vi "WVDIAL+HSRL_v5.6.vi"() -> ()   [LabVIEW 2012]
uses:
  C:/Users/eol-lidar/Desktop/20171016_WVDIALLabviewSlimmed/DLLs/PowerMeterCommands.dll
  DLLs/PowerMeterCommands.dll
  <vilib>/DAQmx/write.llb/DAQmx Write (Digital 1D Bool NChan 1Samp 1Line).vi
  <vilib>/DAQmx/miscellaneous.llb/DAQmx Fill In Error Info.vi
  <vilib>/Analysis/baseanly.llb/Mean (DBL).vi
  WVD-MCSupdate/WVDMCSupdate/Subroutines/AMCS_Data.vi
  Shared Telescope WV DIAL Code/Libraries and VIs/Scalar_Data.vi
  <vilib>/Analysis/NI_AALBase.lvlib
  Shared Telescope WV DIAL Code/Libraries and VIs/Scalar_Data_2.vi
  Shared Telescope WV DIAL Code/Libraries and VIs/Scalar_Data_4.vi
  Shared Telescope WV DIAL Code/Libraries and VIs/Scalar_Data_3.vi
  DLLs/CLDevIFace.dll
panel:
  out "sigma_off_total":dbl[](array[numeric])=[5.561752182192097e-25, 5.543502425482937e-25, 5.525286776509028e-25, 5.507105267834132e-25, 5.488957932126663e-25, 5.470844802256444e-25, 5.452765911101733e-25, 5.434721291706492e-25, 5.416710977203383e-25, 5.398735000734361e-25, 5.380793395556204e-25, 5.362886194923337e-25, 5.345013432148163e-25, 5.327175140545496e-25, 5.309371353401882e-25, 5.2916021040427205e-25, 5.273867425735806e-25, 5.256167351714557e-25, 5.238501915156585e-25, 5.220871149168608e-25, 5.2032750867970615e-25, 5.185713760965108e-25, 5.16818720451498e-25, 5.150695450167362e-25, 5.133238530494676e-25, 5.115816477960978e-25, 5.098429324843519e-25, 5.081077103253636e-25, 5.063759845141784e-25, 5.046477582239893e-25, 5.0292303461145e-25, 5.012018168074178e-25, 4.994841079208481e-25, 4.977699110405206e-25, 4.960592292252991e-25, 4.943520655119366e-25, 4.9264842290519855e-25, 4.909483043867978e-25, 4.892517129052874e-25, 4.875586513787884e-25, 4.858691226971689e-25, 4.841831297166355e-25, 4.825006752543411e-25, 4.808217621002523e-25, 4.791463930057659e-25, 4.774745706846224e-25, 4.7580629781515705e-25, 4.741415770356795e-25, 4.724804109451955e-25, 4.708228021047316e-25, 4.6916875303125385e-25, 4.67518266200415e-25, 4.6587134404804e-25, 4.642279889605549e-25, 4.625882032864318e-25, 4.609519893243784e-25, 4.593193493288615e-25, 4.576902855057731e-25, 4.560648000174122e-25, 4.544428949731033e-25, 4.528245724384268e-25, 4.512098344233702e-25, 4.495986828926446e-25, 4.479911197575997e-25, 4.463871468777747e-25, 4.447867660625189e-25, 4.43189979068954e-25, 4.415967875975391e-25, 4.400071932975711e-25, 4.384211977618739e-25, 4.36838802531331e-25, 4.352600090892456e-25, 4.336848188647951e-25, 4.321132332291639e-25, 4.305452534971783e-25, 4.289808809279486e-25, 4.2742011672071225e-25, 4.258629620199571e-25, 4.243094179083304e-25, 4.227594854132745e-25, 4.212131655002161e-25, 4.196704590788522e-25, 4.181313669960296e-25, 4.165958900404223e-25, 4.150640289409102e-25, 4.1353578436580916e-25, 4.12011156923498e-25, 4.104901471585589e-25, 4.089727555606462e-25, 4.0745898255287632e-25, 4.059488284993571e-25, 4.0444229370438294e-25, 4.0293937840896656e-25, 4.014400827940419e-25, 3.999444069755499e-25, 3.9845235101354183e-25, 3.969639149014037e-25, 3.9547909857346956e-25, 3.939979019023365e-25, 3.925203246968599e-25, 3.9104636670814153e-25, 3.8957602762028764e-25, 3.8810930706173083e-25, 3.866462045949355e-25, 3.85186719722267e-25, 3.837308518864686e-25, 3.8227860046637432e-25, 3.80829964782557e-25, 3.793849440915136e-25, 3.779435375918537e-25, 3.7650574441937656e-25, 3.750715636524266e-25, 3.7364099430430667e-25, 3.7221403533351837e-25, 3.7079068563566637e-25, 3.693709440478561e-25, 3.6795480934616738e-25, 3.6654228024909808e-25, 3.651333554181692e-25, 3.6372803345242974e-25, 3.6232631289607184e-25, 3.609281922331212e-25, 3.5953366989007554e-25, 3.5814274423905253e-25, 3.5675541359037734e-25, 3.5537167620271367e-25, 3.539915302741494e-25, 3.5261497395062725e-25, 3.512420053194509e-25, 3.4987262241518894e-25, 3.4850682321588814e-25, 3.471446056456973e-25, 3.4578596757510757e-25, 3.4443090682164883e-25, 3.430794211490976e-25, 3.4173150826695617e-25, 3.40387165836129e-25, 3.390463914606158e-25, 3.37709182699569e-25, 3.3637553705486374e-25, 3.350454519816831e-25, 3.337189248846164e-25, 3.323959531178655e-25, 3.3107653398769254e-25, 3.29760664750051e-25, 3.2844834261511436e-25, 3.271395647443673e-25, 3.2583432825129606e-25, 3.2453263020474272e-25, 3.2323446762705243e-25, 3.2193983749323496e-25, 3.2064873673450423e-25, 3.193611622390686e-25, 3.180771108479372e-25, 3.167965793620153e-25, 3.1551956453621976e-25, 3.1424606308521448e-25, 3.12976071680503e-25, 3.117095869534258e-25, 3.104466054941991e-25, 3.091871238497953e-25, 3.0793113853283025e-25, 3.0667864601217453e-25, 3.0542964272015646e-25, 3.0418412505014397e-25, 3.029420893588374e-25, 3.0170353196359345e-25, 3.0046844914894554e-25, 2.992368371589509e-25, 2.980086922059933e-25, 2.9678401046518705e-25, 2.9556278807888944e-25, 2.943450211532379e-25, 2.9313070576457556e-25, 2.9191983795267953e-25, 2.907124137258925e-25, 2.895084290635122e-25, 2.8830787991081537e-25, 2.8711076218309027e-25, 2.859170717652124e-25, 2.8472680451222477e-25, 2.8353995625196194e-25, 2.8235652277975173e-25, 2.8117649986558313e-25, 2.7999988325219016e-25, 2.7882666865307774e-25, 2.7765685175696382e-25, 2.7649042822429354e-25, 2.7532739369120183e-25, 2.741677437688488e-25, 2.730114740426547e-25, 2.718585800741375e-25, 2.7070905740222066e-25, 2.69562901540157e-25, 2.6842010798079194e-25, 2.6728067219283387e-25, 2.661445896234197e-25, 2.6501185569798014e-25, 2.6388246582293247e-25, 2.6275641538023513e-25, 2.616336997356157e-25, 2.60514314231774e-25, 2.593982541945556e-25, 2.5828551492935465e-25, 2.5717609172346685e-25, 2.560699798464901e-25, 2.549671745497334e-25, 2.538676710668411e-25, 2.5277146461645525e-25, 2.516785503976567e-25, 2.505889235961241e-25, 2.4950257938010373e-25, 2.4841951290291143e-25, 2.473397193030522e-25, 2.462631937044531e-25, 2.451899312145577e-25, 2.4411992693046025e-25, 2.430531759322844e-25, 2.4198967328846266e-25, 2.4092941405420186e-25, 2.39872393272301e-25, 2.388186059712237e-25, 2.3776804717002872e-25, 2.367207118736947e-25, 2.356765950782586e-25, 2.3463569176525954e-25, 2.335979969081922e-25, 2.325635054684053e-25, 2.3153221239689333e-25, 2.3050411263537554e-25, 2.294792011154746e-25, 2.284574727588212e-25, 2.274389224766938e-25, 2.264235451747459e-25, 2.2541133574601266e-25, 2.244022890765239e-25, 2.23396400044333e-25, 2.2239366351836315e-25, 2.21394074360395e-25, 2.203976274244917e-25, 2.1940431755605105e-25, 2.1841413959462833e-25, 2.1742708837184026e-25, 2.1644315871301047e-25, 2.154623454360858e-25, 2.144846433525735e-25, 2.135100472690121e-25, 2.1253855198334254e-25, 2.115701522900455e-25, 2.1060484297541854e-25, 2.0964261882209755e-25, 2.086834746060555e-25, 2.077274050997275e-25, 2.0677440506727251e-25, 2.058244692709451e-25, 2.048775924672437e-25, 2.0393376940616113e-25, 2.029929948357508e-25, 2.02055263498564e-25, 2.0112057013347119e-25, 2.0018890947358364e-25, 1.9926027625051027e-25, 1.9833466518985033e-25, 1.9741207101473141e-25, 1.9649248844463167e-25, 1.955759121953354e-25, 1.9466233697862308e-25, 1.9375175750525877e-25, 1.9284416848027954e-25, 1.919395646078448e-25, 1.9103794058885478e-25, 1.9013929112014526e-25, 1.8924361089835089e-25, 1.883508946160345e-25, 1.874611369639862e-25, 1.865743326301891e-25, 1.856904763013215e-25, 1.8480956266241805e-25, 1.839315863955293e-25, 1.8305654218173796e-25, 1.821844247006056e-25, 1.813152286297103e-25, 1.8044894864538793e-25, 1.7958557942351787e-25, 1.7872511563801019e-25, 1.7786755196193276e-25, 1.7701288306748196e-25, 1.76161103626729e-25, 1.7531220831027008e-25, 1.7446619178844077e-25, 1.7362304873139562e-25, 1.7278277380850455e-25, 1.719453616897912e-25, 1.711108070452065e-25, 1.7027910454420425e-25, 1.6945024885607005e-25, 1.6862423465142029e-25, 1.6780105660194305e-25, 1.6698070937813746e-25, 1.6616318765208027e-25, 1.6534848609801538e-25, 1.6453659938919535e-25, 1.6372752220073944e-25, 1.6292124920939515e-25, 1.6211777509352618e-25, 1.6131709453201433e-25, 1.6051920220608325e-25, 1.5972409280010035e-25, 1.5893176099733145e-25, 1.5814220148607808e-25, 1.5735540895495118e-25, 1.5657137809645292e-25, 1.5579010360478875e-25, 1.550115801761175e-25, 1.5423580251066348e-25, 1.5346276531215311e-25, 1.526924632848639e-25, 1.5192489113829988e-25, 1.5116004358516276e-25, 1.5039791534159869e-25, 1.4963850112671256e-25, 1.4888179566389964e-25, 1.481277936803633e-25, 1.473764899079385e-25, 1.4662787908173867e-25, 1.458819559412238e-25, 1.4513871523192763e-25, 1.4439815170135076e-25, 1.4366026010455229e-25, 1.4292503519884967e-25, 1.421924717483398e-25, 1.4146256452148893e-25, 1.4073530829242735e-25, 1.4001069783998057e-25, 1.3928872794854995e-25, 1.3856939340929826e-25, 1.3785268901741972e-25, 1.371386095751444e-25, 1.3642714988960654e-25, 1.3571830477488732e-25, 1.3501206905045525e-25, 1.3430843754217699e-25, 1.3360740508330465e-25, 1.3290896651114226e-25, 1.322131166719735e-25, 1.3151985041651617e-25, 1.308291626038556e-25, 1.3014104809867663e-25, 1.294555017723453e-25, 1.2877251850416015e-25, 1.280920931788039e-25, 1.2741422068882974e-25, 1.267388959336285e-25, 1.260661138194001e-25, 1.2539586925949367e-25, 1.2472815717427464e-25, 1.2406297249099328e-25, 1.23400310144304e-25, 1.2274016507553443e-25, 1.220825322337212e-25, 1.2142740657460956e-25, 1.2077478306075468e-25, 1.2012465666234459e-25, 1.1947702235651984e-25, 1.1883187512715506e-25, 1.1818920996493988e-25, 1.1754902186795484e-25, 1.1691130584132554e-25, 1.1627605689635239e-25, 1.156432700517033e-25, 1.1501294033236773e-25, 1.143850627699186e-25, 1.1375963240293268e-25, 1.131366442760479e-25, 1.1251609344039169e-25, 1.1189797495335014e-25, 1.1128228387839706e-25, 1.1066901528543347e-25, 1.100581642493591e-25, 1.0944972585195393e-25, 1.0884369518037427e-25, 1.0824006732660947e-25, 1.0763883738871878e-25, 1.0704000047033016e-25, 1.0644355167879396e-25, 1.058494861281882e-25, 1.0525779893576156e-25, 1.0466848522431205e-25, 1.0408154012094954e-25, 1.0349695875632433e-25, 1.0291473626612958e-25, 1.0233486778924381e-25, 1.0175734846887679e-25, 1.0118217345080934e-25, 1.0060933788495056e-25, 1.0003883692372729e-25, 9.947066572272632e-26, 9.890481943993125e-26, 9.834129323618544e-26, 9.778008227479568e-26, 9.722118172005153e-26, 9.666458673879376e-26, 9.611029249960303e-26, 9.555829417190759e-26, 9.500858692692185e-26, 9.446116593589411e-26, 9.391602637156888e-26, 9.337316340648176e-26, 9.283257221454584e-26, 9.229424796819011e-26, 9.17581858406868e-26, 9.122438100471338e-26, 9.069282863168144e-26, 9.01635238930959e-26, 8.963646195839229e-26, 8.911163799659836e-26, 8.858904717444121e-26, 8.806868465731863e-26, 8.755054560835323e-26, 8.703462518861524e-26, 8.652091855685159e-26, 8.600942086956594e-26, 8.550012727921081e-26, 8.499303293699853e-26, 8.448813298920711e-26, 8.398542258011812e-26, 8.348489684944643e-26, 8.298655093369726e-26, 8.249037996503694e-26, 8.199637907189584e-26, 8.150454337804106e-26, 8.101486800303504e-26, 8.052734806197629e-26, 8.004197866463189e-26, 7.955875491608392e-26, 7.907767191664241e-26, 7.859872476080315e-26, 7.812190853848199e-26, 7.76472183334557e-26, 7.717464922419652e-26, 7.670419628338345e-26, 7.62358545780929e-26, 7.576961916930796e-26, 7.530548511159635e-26, 7.484344745429333e-26, 7.438350123996826e-26, 7.39256415048854e-26, 7.346986327918026e-26, 7.301616158686927e-26, 7.256453144491495e-26, 7.211496786429527e-26, 7.166746584904671e-26, 7.122202039700718e-26, 7.077862649933649e-26, 7.033727914027225e-26, 6.989797329796322e-26, 6.946070394367306e-26, 6.902546604198178e-26, 6.859225455065896e-26, 6.81610644215122e-26, 6.773189059918994e-26, 6.730472802212255e-26, 6.687957162190584e-26, 6.645641632404418e-26, 6.603525704747876e-26, 6.561608870483044e-26, 6.519890620235893e-26, 6.478370444033405e-26, 6.437047831236655e-26, 6.395922270652735e-26, 6.354993250480589e-26, 6.31426025832298e-26, 6.273722781218477e-26, 6.233380305619138e-26, 6.19323231744663e-26, 6.153278302067075e-26, 6.113517744339678e-26, 6.07395012854635e-26, 6.03457493853967e-26, 5.995391657673181e-26, 5.956399768781814e-26, 5.917598754274775e-26, 5.878988096104469e-26, 5.840567275833304e-26, 5.802335774556795e-26, 5.764293073036093e-26, 5.726438651607821e-26, 5.688771990296189e-26, 5.651292568756978e-26, 5.613999866325389e-26, 5.576893362060895e-26, 5.539972534712775e-26, 5.503236862770957e-26, 5.466685824518614e-26, 5.430318897948391e-26, 5.394135560916683e-26, 5.358135291063287e-26, 5.32231756587805e-26, 5.286681862685396e-26, 5.251227658682356e-26, 5.215954431039021e-26, 5.180861656749257e-26, 5.145948812799119e-26, 5.111215376115772e-26, 5.0766608236094594e-26, 5.042284632198532e-26, 5.008086278798998e-26, 4.9740652403889376e-26, 4.940220993989596e-26, 4.906553016678205e-26, 4.8730607856508595e-26, 4.8397437781971205e-26, 4.806601471760013e-26, 4.77363334387833e-26, 4.740838872286381e-26, 4.7082175348572594e-26, 4.6757688096656775e-26, 4.643492174989336e-26, 4.611387109292415e-26, 4.5794530912563533e-26, 4.547689599781122e-26, 4.5160961140154586e-26, 4.484672113314862e-26, 4.453417077278691e-26, 4.422330485756757e-26, 4.3914118187998816e-26, 4.360660556710048e-26, 4.330076179997986e-26, 4.299658169393312e-26, 4.269406005832397e-26, 4.2393191704061123e-26, 4.209397144390232e-26, 4.179639409188714e-26, 4.150045446321139e-26, 4.120614737376086e-26, 4.0913467639878655e-26, 4.0622410078074736e-26, 4.0332969504153414e-26, 4.0045140732752307e-26, 3.975891857729729e-26, 3.9474297848629725e-26, 3.919127335477734e-26, 3.8909839899739583e-26, 3.862999228300389e-26, 3.835172529819719e-26, 3.80750337323718e-26, 3.779991236448816e-26, 3.752635596434186e-26, 3.725435929114848e-26, 3.6983917092082905e-26, 3.6715024100514326e-26, 3.64476750344056e-26, 3.618186459428844e-26, 3.591758746135901e-26, 3.565483829498213e-26, 3.5393611730607343e-26, 3.513390237722922e-26, 3.4875704814322724e-26]
  out "sigma_on_total":dbl[](array[numeric])=[3.4515002360178425e-23, 3.453572235363748e-23, 3.455588140684375e-23, 3.457547684705289e-23, 3.4594506038607345e-23, 3.461296638484173e-23, 3.463085532323546e-23, 3.46481703306302e-23, 3.466490892310268e-23, 3.4681068653051854e-23, 3.469664711519079e-23, 3.471164194154948e-23, 3.4726050806113556e-23, 3.4739871423950697e-23, 3.475310154887194e-23, 3.476573898025495e-23, 3.4777781557893985e-23, 3.4789227163142567e-23, 3.4800073722238876e-23, 3.481031920535573e-23, 3.481996162632877e-23, 3.482899904309283e-23, 3.4837429558845977e-23, 3.484525132322997e-23, 3.485246252980516e-23, 3.4859061420906976e-23, 3.486504628361222e-23, 3.4870415453115073e-23, 3.4875167311632143e-23, 3.4879300290303973e-23, 3.488281286654148e-23, 3.4885703569731826e-23, 3.488797097473508e-23, 3.488961370836255e-23, 3.489063044589183e-23, 3.4891019912944045e-23, 3.4890780885821923e-23, 3.488991219184056e-23, 3.488841270806428e-23, 3.488628136476675e-23, 3.4883517142573345e-23, 3.488011907512697e-23, 3.487608624697385e-23, 3.487141779623187e-23, 3.486611291324836e-23, 3.486017084165558e-23, 3.4853590878616424e-23, 3.4846372374239696e-23, 3.4838514731789615e-23, 3.4830017410372377e-23, 3.482087992184721e-23, 3.4811101831825777e-23, 3.480068276235606e-23, 3.4789622387923395e-23, 3.477792043894559e-23, 3.4765576701942813e-23, 3.4752591015444286e-23, 3.473896327688835e-23, 3.4724693436809294e-23, 3.470978150062252e-23, 3.4694227532161045e-23, 3.4678031646883943e-23, 3.466119402056769e-23, 3.4643714880731176e-23, 3.462559451186541e-23, 3.4606833256372457e-23, 3.4587431510225346e-23, 3.456738972648089e-23, 3.4546708412648005e-23, 3.452538813332637e-23, 3.4503429510209843e-23, 3.448083321760521e-23, 3.4457599987727524e-23, 3.443373060978343e-23, 3.4409225926316653e-23, 3.438408683672287e-23, 3.4358314294459105e-23, 3.433190931148268e-23, 3.4304872951794084e-23, 3.427720633676941e-23, 3.4248910642306304e-23, 3.421998709867614e-23, 3.419043699128879e-23, 3.4160261661462425e-23, 3.412946250347978e-23, 3.409804096531635e-23, 3.4065998551237755e-23, 3.4033336817878806e-23, 3.400005737588303e-23, 3.396616188873896e-23, 3.3931652074420655e-23, 3.3896529703262367e-23, 3.38607965976923e-23, 3.382445463385435e-23, 3.378750573753358e-23, 3.3749951890516246e-23, 3.371179512172702e-23, 3.367303751357746e-23, 3.363368120070749e-23, 3.3593728364854914e-23, 3.355318124026283e-23, 3.3512042110452034e-23, 3.347031330978982e-23, 3.342799721924958e-23, 3.338509627086632e-23, 3.334161294444553e-23, 3.3297549766181377e-23, 3.325290931214395e-23, 3.3207694203964155e-23, 3.3161907110354505e-23, 3.311555074667654e-23, 3.306862787449936e-23, 3.302114129917655e-23, 3.297309387233545e-23, 3.2924488490428247e-23, 3.2875328092275295e-23, 3.282561566055147e-23, 3.27753542222894e-23, 3.2724546846397307e-23, 3.2673196642148416e-23, 3.262130676264614e-23, 3.256888040031936e-23, 3.251592078838197e-23, 3.246243120029814e-23, 3.240841494924143e-23, 3.2353875385536375e-23, 3.2298815898103865e-23, 3.224323991591418e-23, 3.218715090138306e-23, 3.2130552355831734e-23, 3.2073447815888415e-23, 3.2015840852899003e-23, 3.195773507537017e-23, 3.189913412129057e-23, 3.1840041667650374e-23, 3.178046141970931e-23, 3.1720397118491994e-23, 3.16598525330712e-23, 3.1598831468073684e-23, 3.153733775594661e-23, 3.147537525835796e-23, 3.141294786658458e-23, 3.135005950291899e-23, 3.12867141139156e-23, 3.122291567586735e-23, 3.1158668191103796e-23, 3.109397568836599e-23, 3.102884221909099e-23, 3.0963271863917515e-23, 3.0897268723854685e-23, 3.083083692473897e-23, 3.076398061453296e-23, 3.069670396369062e-23, 3.062901116552433e-23, 3.0560906430420534e-23, 3.0492393992351233e-23, 3.0423478103089006e-23, 3.035416303359352e-23, 3.028445307334954e-23, 3.021435252662646e-23, 3.0143865718994697e-23, 3.007299698845757e-23, 3.0001750689917396e-23, 2.993013119246171e-23, 2.9858142879727496e-23, 2.978579014924072e-23, 2.971307741073149e-23, 2.964000908547624e-23, 2.956658960666605e-23, 2.9492823419775624e-23, 2.941871497781172e-23, 2.934426874578359e-23, 2.9269489195956677e-23, 2.9194380809253694e-23, 2.911894807358691e-23, 2.904319548628236e-23, 2.8967127546285775e-23, 2.889074876374468e-23, 2.8814063649158965e-23, 2.8737076719899763e-23, 2.8659792496518843e-23, 2.858221550314507e-23, 2.8504350265844524e-23, 2.842620131099115e-23, 2.8347773170754424e-23, 2.82690703723236e-23, 2.8190097447468315e-23, 2.811085892584043e-23, 2.8031359334384736e-23, 2.795160320181344e-23, 2.787159505092985e-23, 2.7791339403111763e-23, 2.771084077772887e-23, 2.763010368753301e-23, 2.75491326421318e-23, 2.746793214641421e-23, 2.7386506697984487e-23, 2.730486078862673e-23, 2.722299890475956e-23, 2.7140925523887364e-23, 2.7058645116074616e-23, 2.697616214341637e-23, 2.6893481058516993e-23, 2.681060630397897e-23, 2.672754231388484e-23, 2.664429351030695e-23, 2.656086430480396e-23, 2.6477259099906563e-23, 2.63934822816981e-23, 2.630953822627762e-23, 2.62254312982857e-23, 2.614116584649427e-23, 2.6056746207296864e-23, 2.597217670130493e-23, 2.5887461635852605e-23, 2.5802605303570342e-23, 2.5717611979999804e-23, 2.563248592513051e-23, 2.5547231382007618e-23, 2.5461852579237722e-23, 2.5376353725722492e-23, 2.5290739013185455e-23, 2.52050126148148e-23, 2.5119178687776108e-23, 2.5033241368970833e-23, 2.494720477372477e-23, 2.486107300311006e-23, 2.4774850133032473e-23, 2.468854022251904e-23, 2.4602147308589812e-23, 2.4515675408789892e-23, 2.4429128518009252e-23, 2.434251060912738e-23, 2.4255825636481401e-23, 2.4169077528001048e-23, 2.408227019153271e-23, 2.3995407511716315e-23, 2.390849335157963e-23, 2.382153154758751e-23, 2.3734525916855995e-23, 2.364748024942069e-23, 2.3560398311727402e-23, 2.347328384730596e-23, 2.3386140574674015e-23, 2.329897218619409e-23, 2.3211782352450444e-23, 2.3124574714679822e-23, 2.3037352891909005e-23, 2.295012047616546e-23, 2.2862881033206724e-23, 2.2775638104148126e-23, 2.268839520345904e-23, 2.2601155819694246e-23, 2.2513923411731382e-23, 2.2426701417601178e-23, 2.2339493242652746e-23, 2.2252302268385215e-23, 2.2165131848713943e-23, 2.207798530984225e-23, 2.1990865951904698e-23, 2.1903777045307318e-23, 2.1816721834153286e-23, 2.172970353524044e-23, 2.1642725336208165e-23, 2.1555790398068828e-23, 2.146890185249782e-23, 2.138206280436143e-23, 2.1295276329034764e-23, 2.1208545474925844e-23, 2.1121873260820957e-23, 2.103526267755169e-23, 2.0948716689634593e-23, 2.086223822840444e-23, 2.077583020218935e-23, 2.0689495485230986e-23, 2.060323692781895e-23, 2.0517057348655242e-23, 2.0430959539052178e-23, 2.034494626206417e-23, 2.0259020249983245e-23, 2.0173184208498126e-23, 2.0087440813365583e-23, 2.0001792712897014e-23, 1.991624252549357e-23, 1.9830792842125428e-23, 1.974544622308171e-23, 1.9660205201265445e-23, 1.9575072282200615e-23, 1.949004994082927e-23, 1.9405140623986183e-23, 1.9320346750432794e-23, 1.923567071169047e-23, 1.915111486810961e-23, 1.9066681553707904e-23, 1.8982373073047866e-23, 1.8898191704453675e-23, 1.881413969535917e-23, 1.873021926709263e-23, 1.8646432612590997e-23, 1.8562781895712654e-23, 1.8479269254414894e-23, 1.8395896797739073e-23, 1.831266660592076e-23, 1.8229580733541875e-23, 1.8146641207318404e-23, 1.806385002545182e-23, 1.7981209160004765e-23, 1.7898720555487374e-23, 1.7816386128971637e-23, 1.7734207770209112e-23, 1.7652187343968405e-23, 1.7570326685697343e-23, 1.748862760682514e-23, 1.740709188899069e-23, 1.73257212915044e-23, 1.7244517544151243e-23, 1.7163482351713297e-23, 1.7082617393360188e-23, 1.7001924321344786e-23, 1.692140476400989e-23, 1.6841060321633093e-23, 1.6760892570856573e-23, 1.6680903062681705e-23, 1.660109332262017e-23, 1.6521464851544674e-23, 1.6442019124440084e-23, 1.636275759264924e-23, 1.6283681683313138e-23, 1.6204792797459998e-23, 1.6126092313608594e-23, 1.6047581584489582e-23, 1.596926194062211e-23, 1.5891134687741356e-23, 1.5813201107651e-23, 1.57354624590593e-23, 1.5657919978398576e-23, 1.5580574876658608e-23, 1.5503428344213284e-23, 1.5426481547000454e-23, 1.5349735628683665e-23, 1.5273191711461729e-23, 1.5196850893628633e-23, 1.5120714252353987e-23, 1.5044782842549766e-23, 1.496905769768598e-23, 1.4893539828685258e-23, 1.4818230226012358e-23, 1.4743129858566772e-23, 1.466823967323771e-23, 1.4593560597590975e-23, 1.451909353690664e-23, 1.444483937747518e-23, 1.4370798983051104e-23, 1.4296973199357064e-23, 1.4223362849950735e-23, 1.4149968740688154e-23, 1.4076791656234235e-23, 1.4003832362073226e-23, 1.393109160467734e-23, 1.385857011048832e-23, 1.3786268587886926e-23, 1.371418772558386e-23, 1.3642328195156863e-23, 1.3570690647116186e-23, 1.3499275716936324e-23, 1.3428084018813628e-23, 1.3357116150507314e-23, 1.3286372692908264e-23, 1.3215854207921409e-23, 1.3145561240370374e-23, 1.3075494317602393e-23, 1.3005653950228148e-23, 1.2936040632287998e-23, 1.2866654840864186e-23, 1.279749703626037e-23, 1.2728567662180764e-23, 1.2659867146998256e-23, 1.25913959017358e-23, 1.2523154323507594e-23, 1.2455142791347836e-23, 1.2387361670712388e-23, 1.2319811310943876e-23, 1.2252492045988474e-23, 1.2185404195095507e-23, 1.2118548062976809e-23, 1.2051923938926186e-23, 1.1985532098038971e-23, 1.1919372801369668e-23, 1.1853446295576834e-23, 1.178775281309274e-23, 1.1722292572798084e-23, 1.1657065779169588e-23, 1.1592072624964016e-23, 1.1527313286848077e-23, 1.1462787931079687e-23, 1.139849670866529e-23, 1.1334439759006425e-23, 1.127061720758601e-23, 1.1207029169063776e-23, 1.1143675744010233e-23, 1.1080557021981866e-23, 1.1017673079256681e-23, 1.0955023980440454e-23, 1.0892609779081287e-23, 1.0830430516392804e-23, 1.076848622235415e-23, 1.0706776914923493e-23, 1.0645302601586044e-23, 1.0584063279021457e-23, 1.0523058931873951e-23, 1.0462289534286939e-23, 1.0401755050939685e-23, 1.0341455434019563e-23, 1.0281390627428863e-23, 1.0221560563765352e-23, 1.0161965164931961e-23, 1.0102604343605913e-23, 1.0043478003355295e-23, 9.984586037022776e-24, 9.925928328181409e-24, 9.867504750832607e-24, 9.809315169968762e-24, 9.75135944169672e-24, 9.693637412519841e-24, 9.63614892031981e-24, 9.578893794477301e-24, 9.521871855164951e-24, 9.465082914311581e-24, 9.408526775719018e-24, 9.352203234772622e-24, 9.29611207816474e-24, 9.240253085636872e-24, 9.184626028473818e-24, 9.129230670035649e-24, 9.074066766274049e-24, 9.019134065058834e-24, 8.964432307866704e-24, 8.909961227543955e-24, 8.855720551151387e-24, 8.80170999774117e-24, 8.74792927963555e-24, 8.694378102530001e-24, 8.641056164469263e-24, 8.587963157847659e-24, 8.535098768003274e-24, 8.482462674444791e-24, 8.430054549473157e-24, 8.377874059403957e-24, 8.325920865386509e-24, 8.274194620959618e-24, 8.22269497505898e-24, 8.171421569946106e-24, 8.120374042744336e-24, 8.069552024466193e-24, 8.018955141170296e-24, 7.968583012653601e-24, 7.918435254636004e-24, 7.868511476078817e-24, 7.818811281362761e-24, 7.769334270699e-24, 7.720080038178343e-24, 7.671048173562992e-24, 7.62223826136358e-24, 7.573649881599091e-24, 7.525282610203139e-24, 7.477136017792332e-24, 7.429209670743598e-24, 7.381503131591651e-24, 7.334015957500456e-24, 7.286747702596049e-24, 7.239697915806835e-24, 7.192866142852962e-24, 7.146251925366177e-24, 7.099854800662283e-24, 7.053674302444568e-24, 7.007709960568416e-24, 6.961961301421992e-24, 6.916427847693127e-24, 6.871109118744303e-24, 6.826004630381647e-24, 6.781113894340264e-24, 6.736436420426319e-24, 6.691971713924284e-24, 6.647719277729405e-24, 6.603678611242115e-24, 6.559849211017784e-24, 6.5162305705432474e-24, 6.472822180305278e-24, 6.429623528416676e-24, 6.386634099554385e-24, 6.34385337614641e-24, 6.301280837596942e-24, 6.2589159614474176e-24, 6.2167582215217655e-24, 6.174807090439789e-24, 6.133062037235496e-24, 6.091522529571197e-24, 6.0501880321847015e-24, 6.009058008010654e-24, 5.968131917184469e-24, 5.927409218405094e-24, 5.8868893679427144e-24, 5.846571819704099e-24, 5.806456026305333e-24, 5.76654143809886e-24, 5.726827503485023e-24, 5.687313669212257e-24, 5.647999380175983e-24, 5.608884079470536e-24, 5.569967208682166e-24, 5.531248207691008e-24, 5.492726514720866e-24, 5.454401566388544e-24, 5.416272798222205e-24, 5.378339643992548e-24, 5.3406015362316215e-24, 5.3030579058109185e-24, 5.2657081824525174e-24, 5.228551794992721e-24, 5.191588170509665e-24, 5.154816734830585e-24, 5.118236913241346e-24, 5.081848129623247e-24, 5.0456498062843654e-24, 5.0096413655378555e-24, 4.9738222277620295e-24, 4.938191812756974e-24, 4.902749539556105e-24, 4.867494826246496e-24, 4.8324270897980386e-24, 4.7975457465251376e-24, 4.7628502123229794e-24, 4.7283399018695166e-24, 4.6940142290838214e-24, 4.659872607969946e-24, 4.625914450817829e-24, 4.592139170464571e-24, 4.5585461781112564e-24, 4.525134884962285e-24, 4.49190470184733e-24, 4.4588550388605404e-24, 4.4259853055918835e-24, 4.393294911349112e-24, 4.360783264993124e-24, 4.328449775343777e-24, 4.2962938500795836e-24, 4.264314897642654e-24, 4.232512325393204e-24, 4.200885540575948e-24, 4.169433950522323e-24, 4.138156962127184e-24, 4.107053982061292e-24, 4.0761244169749535e-24, 4.0453676735180176e-24, 4.014783158012066e-24, 3.984370276655627e-24, 3.954128435720719e-24, 3.924057041741254e-24]
  out "FileHour":i32=22
  out "L_Count":i32=2279
  out "background start":u32=534
  in  "Tab Control 2":enum32{"WV ND ", "Aerosol Backscatter"}(tab)
  out "Absolute Humdity":dbl[][](graph)=[[2.381637996198332, 3.2289304662519207, 3.7399508862716324, 2.9391297670300416, 3.541243431316799, 3.6903758226189978, 2.985510135495457, 3.271802799342691, 3.0570815242212315, 2.728847864410741, 3.073021424734379, 3.243072414368595, 3.1548970439889157, 3.282553159546102, 3.108115688416444, 2.722753101265902, 2.8449703706793494, 3.206528613382733, 3.3476157130731745, 3.7190707194892743, 3.6779958509768855, 2.7102752010337867, 2.1544952515278166, 1.4465403162714228, 0.7114767801380684, 0.6298686521869906, 0.7518894516657683, 1.0869728077475849, 1.0965823199341656, 1.3419805753992218, 1.7357331019053095, 1.331267180889126, 1.6812045362627965, 1.7505545925065586, 1.0515797250761254, 1.8248068084521747, 1.229507265807658, 0.5932832152277314, 1.3793197306303144, 0.8025994248365454, 1.313331659994041, 1.0877069837557727, 0.6676059805515389, 1.108268188194286, 1.218310374753867, 0.9302230718225697, 0.5379773620409434, 0.40864508327626387, 0.4878195780051225, 0.6158457328090234, 0.11371277866873461, -0.21554539012342172, -0.2406042501222398, -0.20617359320538328, 0.18486916184575064, 0.12017721733703236, 0.2321649548288094, 0.5605674714389408, 0.3258630233758466, -0.3184085423773992, 0.5396974021515508, 1.4630150688505692, 1.3990688136693945, 0.9030393856696112, 0.526395588284596, 0.9275740265066234, 1.1599331759526064, 0.5100558681034059, 0.09120297180026139, 0.8941505360141835, 0.2729880366179525, 0.06592897868761208, 0.4494387103915796, 0.47986401248106203, 0.6036626512429464, 0.8075827814717941, 0.39580615117043777, 0.7330008432298232, 2.3807348332184937, 1.9103595505677082, 0.0038875758198880076, -0.5099538555154887, -0.2631995404689374, -0.06897603937656993, 1.077598454394292, 0.4811274468413941, 0.8743567150048569, 1.2133377410991968, -2.058173207390024, -2.768533001862221, -0.24709157558471373, -0.2813196490058808, -0.762592251504898, -0.9310225611607561, -1.9782833951773926, -2.308433360075538, -2.641473972541387, -2.4409629901461876, 0.7310950717981377, 3.055251966138101, 1.0625831441621862, -0.14282321715115798, 1.6125338803763605, 2.273348316609188, 0.5762806799617023, 3.783642625574112, 3.794462892171507, 0.3213956058161953, 0.6052989532593476, 0.6410723860892351, 1.071873965770129, 0.9457697955061203, 0.6818176903636604, 0.07395127869072624, -0.5063844607054439, -1.1437899792745225, 2.5340085201026783, 4.357418369352322, 0.6619021916765269, -0.598536929925543, 2.0392887388158476, 2.963311635184338, -0.19409867099506645, -1.019543939477428, 3.284669801197826, 5.053322162029661, 0.5318597562673084, -1.046234519869084, -1.4725750000538156, -3.0965262150405803, -2.4717454851967853, -2.5919741810617096, -3.454274629674715, 0.5381779942126864, -3.5639021358857397, -8.604218550497471, -3.291035594836002, -4.988396563367619, -3.4959011235715116, 3.6822742352793214, 4.5654685349418145, 5.450258155777445, 2.2660863701994107, -4.357142477299314, 3.245574805662169, 7.1420821928675515, 4.687963483201633, 9.84865044186338, 11.603666387771154, 1.3270168499770503, -7.363398139201385, -5.662559010638185, -2.185982348357743, 4.237560848170052, -0.7781152449815046, 0.06900190966136914, -5.112922938956167, -10.248000167321203, -0.7763806780948262, 2.4864790924400806, 1.3458208096776678, -6.375691421917362, 2.7130755986099464, 0.4685593105266804, -4.7583718927506125, 4.893114538127965, 4.338410371047717, -1.9047313519649718, -17.235906530849263, -1.7515646091788906, 15.01473259833217, -0.6559241650564018, -3.381324785057165, 20.523279814816366, 9.418262237736784, 0.6649187522986425, 14.442556008930413, 11.661941009672843, 16.26228369553192, 2.257363451517956, -24.30439045179676, -3.526848266787906, 1.507238317359721, -30.281969291655145, -7.1860637324352155, -8.150116400348827, -6.805358486050646, 17.076841478693954, 16.08424187184452, -9.842881804327654, 6.9974061489486985, 18.014302013509113, 33.52813996759658, -4.3504280928807, -20.329535445003472, -12.706033450227912, 14.841641652177197, -11.014476311441456, -28.652963020018287, -8.835026833040136, -1.1989865463180107, 2.1484394027063125, -14.42847616268741, 20.906355235181202, 44.663295303649214, 52.21277086785295, -33.657330483484074, -41.06737656742905, -15.423109696690162, -9.500704088407685, -10.012361466780659, -16.236466802115963, -1.4084185649673422, -10.619205977347402, -17.973707045135473, -33.01855410212323, 6.0910465995465835, 43.68920448903066, 51.12449140459259, 16.703087852725265, 20.806562818676078, 22.660425459835764, -22.723998594167576, 8.62012287770647, -9.242581553788519, -28.14728762961585, -14.597899966279824, -33.224649735096314, -47.41764866110292, 6.700691596414805, 0.26259793424826255, -23.53025640997093, -35.21546365539503, -75.06437932526299, -31.34745866627544, 11.90853495698821, 13.946592746287827, 1.572271714831353, -3.4881021595916346, -23.070503031187805, -20.737126810032358, 0.39821197087017257, 22.83349305653667, 48.52973190147717, 58.32063867763403, 24.980866356079414, -26.425123000085613, -36.01285461898413, 20.42955755833331, 28.179388150526847, 7.326674672301561, -7.570510880112455, -3.7813689490425424, 15.273239476125202, -13.887091245376999, -9.632858013398996, 16.23568393754438, 34.44331113665626, -16.007414207586113, -25.033654717417868, 10.345654751811987, 16.178632683864706, 22.74327279177682, 13.83131940280649, -26.923571079117785, -47.01299670772383, -7.03102275473792, 7.756783960569631, 38.507482457635646, 12.401593380017964, -40.242006647285045, -35.42995801579476, -19.48535326169341, 13.726928327433772, 7.089603424795179, -9.761657671358787, 30.12572887455403, 5.603956914061026, 15.269052044730138, 39.027215874792205, 28.840850555686185, 9.222119781455913, -6.65875991656153, -52.02758693606492, -24.846772329704105, 26.784665497281033, -29.139711335385233, -60.34533371175373, -95.47692172161051, -20.80364767289969, 13.071657310729377, 32.09252154822125, 11.327643976237049, -1.1746406371192744, 14.821401879518556, 21.869358735257315, -48.40890329377097, 71.70201659410256, 54.26836963273803, -43.929656476547315, -34.517339162747625, -11.183500473546477, 8.16745102755325, 3.5594686047745956, -38.42135327716965, -31.872424510428615, 63.202643858023535, 32.06953455083959, -34.96580601597051, 80.98624804001545, 25.430674707201966, 75.40979957665618, -25.683154067233602, -3.039912556079691, 8.10545244225573, -10.025258739410638, 3.4175561609064777, -94.93347989371179, -18.265867245088412, -110.12143596454362, -20.08363221861497, -81.23907731671687, 25.67338142600785, 11.180698708528315, 53.88801706666816, 82.40024181051014, -24.94794083844046, 64.49693631878343, 82.45151274073672, 23.058155973673617, -55.48688090973129, -11.11936432118781, -52.90874007929736, -10.973448949850733, -35.70404161475429, -79.95994214207809, 79.17644734372716, -47.43996392613031, -63.345899291707084, -1.191569829716015, -51.02579528666298, -16.153598403212513, 59.62335798742518, 44.7938082279846, 35.44272396048698, 26.94391947838042, -81.1231522685912, -37.84608979644942, 79.79513034602873, 27.015501282691233, 101.9886816354312, 1.8567663888741248, 61.1787817112004, 53.27385093417791, 23.918505153010667, 78.42963739321138, 52.41899623229256, -27.76254219474436, -139.76423693070285, -57.369729863336204, -15.75787273988757, -13.900964408545683, -71.2248658979622, -22.326171055405933, -12.538393340975478, -91.23134278655108, -96.71489984592516, 83.61518327624235, 94.01183863967185, -115.51887637839579, -2.8131316684122636, 72.2926822594888, -88.46187718011109, -159.9439857495639, -13.689247148005327, -3.39740618852503, 37.93357297565678, -58.040480173884674, -4.0319312642523135, 158.43820753192094, 36.45062064189213, 28.105591708306047, 154.2957712970144, 122.36412897340807, -124.53229738474322, -56.414573288126846, 24.562350024992103, 95.68918845312272, 67.32794654593681, 44.2881958238465, 35.28861431188373, -30.895984285777292, -118.6165047925672, -17.206766248824636, 149.66599715426307, 94.87002753655919, 125.1362981137479, -57.05477535151939, -108.75623218396714, -156.14973267680034, -118.02049838814683, -45.955138077034555, 94.56117041525165, 22.830201855771985, -50.124240804188766, -0.31036721421730357, -57.36131884949238, 38.81579523823493, 44.29287287978949, 38.5229738338614, 80.79744934280897, 66.13977496552239, 64.29527155177475, -3.009742211798789, 7.091320437039029, -24.145705616003966, -90.45440826714311, -42.22868312890451, 17.4251196909393, 102.86666168297742, -8.193221973854076, -38.10169748406272, -331.44637318920684, -36.14864657498966, -52.08585880605683, -90.12533066952986, -35.8680778149411, -95.8562186667981, -81.59466027176232, -20.664876741135952, -97.56611771145663, -11.243026138770166, 214.69116109499527, -1.2842625977559836, 116.96436728507435, 146.3214589160713, -12.741894974641909, 147.18139330660117, 45.02329654566495, -80.50134037378051, 128.14312863671353, -16.284511482675764, -54.726810070514134, 25.585495034388693, -41.53572548733546, -171.02855146077312, 6.859434938582148, 20.665605828627164, 26.300796764085817, 141.9391976593194, 50.921562772433845, -15.402541734093683, 102.3422300212664, 72.80006285923778, -98.31980003330196, 83.10862914577454, -102.53128072443756, -27.06618359203802, -87.0910710676119, 102.23065521840873, -141.36626971150534, 29.471403724026768, 24.368156479861653, -59.406444870838705, 125.46252216898323, 54.36235619467443, 176.91956044616694, 32.004214794350126, 68.89696634113477, -318.953893641183, 10.918586272433357, 27.93870692723572, -59.96302949556338, -123.4612683447811, -0.3712090888008344, 282.51585058458556, 143.28700749891587, -203.76527384318103, -11.250946010935081, 212.27613615561046, 81.29553615072341, -58.95943360687757, -3.1407015001953793, 146.8378190474621, 107.90240668299298, -262.0484867540934, -262.08868454546376, 248.88675628753427, -2.2883295180231973, 175.48444627220957, -15.13787689666532, 179.9025790965365, -3.1161348684158456, -178.09898915184024, -110.33016689473364, 26.144560408860073, 217.1929959862786, -116.84600312970869, -125.72476717428505, -208.87350762275165, -40.086703269976596, -105.61606531370143, 25.31258223173439, 153.0181503103424, 73.43534127268488, 106.93587454995877, -63.047066135509986, -33.78992823908888, 169.32406945401812, -30.4620039262772, -61.53725751389104, -117.9786292018291, 23.125015797048416, 2.8560249402634366, -115.06719331548341, -172.20968894415537, 42.87702950061471, -91.71407795095956, -34.680200011577824, 152.6778383484745, 183.69312698179476, 40.303525079241524, -153.93410879084288, 10.779576458921726, -112.08159639995125, -80.75175743647412, -79.79059986535235, 248.44403429336876, 65.1693445550873, -155.7732008790998, -237.64454159760322, -130.0929874697878, 273.1707767339364, -63.309773797398535, -100.25386201485678, 157.43990871668723, 89.85074006724048, 29.329162137021854, -590.6810937724066, -61.80604440043233, -39.55170394991537, 151.82089601349833, -244.4747118832092, -111.7902591189255, 106.16177698531308, -125.24240636587366, -163.00303972060732, -187.55493907889863, 660.8082006393893, 167.28564433594212, 526.9020197583936, 103.18712729766843, 171.25658826096995, 230.69797456981095, 197.36345656629953, 138.85917774757226, 150.7674633526593, 0.0, 0.0, 0.0]] caption="Water Vapor Number Density"
  out "Backscatter coef":dbl[][](graph)=[[-5.631855190887778, -6.004505832929174, -6.173141462421788, -6.078638032820708, -5.996551688969127, -6.105979495519012, -6.322610972848886, -6.303696465062151, -6.288864858626744, -6.311829041360893, -6.258887612466116, -6.260252489100467, -6.289601096396406, -6.332700564965553, -6.310221686509206, -6.2482411447374595, -6.288055902535426, -6.286567832734827, -6.288434201879805, -6.423709465041304, -6.503944258551364, -6.526852329894633, -6.587215931775179, -6.573298865738327, -6.586513067404876, -6.6601086370892935, -6.630820925781226, -6.534421336016373, -6.562727741301405, -6.624785444539913, -6.652701895089165, -6.6541773323998665, -6.620108344892257, -6.597410791666123, -6.567384053963737, -6.55193578071735, -6.625602824074351, -6.630359347182261, -6.570115275093481, -6.583952405367042, -6.603436398148079, -6.637802785486154, -6.677589288122656, -6.676677525795413, -6.61510175427215, -6.6171486759339615, -6.574656376388106, -6.488298768765658, -6.515881617061782, -6.545811977677873, -6.468302654464445, -6.468495466328282, -6.588155799923826, -6.499010244011781, -6.424944472398059, -6.586199196925285, -6.643764222023246, -6.48814552290357, -6.528263219652093, -6.675590947657935, -6.7804550168819056, -6.751235102841602, -6.649222918507316, -6.539532403878219, -6.656615933093949, -6.761077450990051, -6.585247119876417, -6.670006797218612, -6.75788870154134, -6.5870257008287005, -6.545564027689246, -6.7299359562097125, -7.135024055994977, -7.215149643358638, -6.854636415994818, -6.796590024058724, -6.5604425353718145, -6.410273733030975, -6.8478558149875, -6.892474319695937, -6.579276253604049, -7.068141789335968, -7.367417948315361, -6.932773718138186, -7.261023712130762, -7.055370746341504, -6.5034973786801205, -7.1119104731081935, nan, nan, nan, nan, -6.441762019443648, -5.912355400683733, -6.9229064427310805, -6.902451674354379, -6.164144503892496, -6.247704912397094, -6.105250273825426, -6.218886162995463, -6.513408609804659, -7.176545729189657, -7.086102682274419, -5.561615277652527, -5.929472655508007, -6.326458185475832, -6.632963512267925, -6.751768726712177, -7.939996215141689, nan, -7.1691130442663304, -6.927686116158072, -6.512795857098227, -7.006013506427372, nan, -6.225145208098167, -5.858248272801253, -5.102261787898304, -5.683091032278954, -7.208255278368322, nan, -6.237850707893898, nan, -7.163584196102564, -7.224277394558059, -7.870430197902702, nan, nan, -6.575413882094829, -5.4824337698020775, -5.701309152242779, -6.569531822381552, -6.599583135587987, -6.2615020091653015, -5.893609876994032, nan, nan, nan, nan, nan, -6.986035931251345, -6.3686603148487, -6.6040587369138075, -6.702981929100622, -7.145160152250116, nan, nan, nan, -6.846401330698514, nan, -6.2872744724089324, -7.650475678042142, nan, -6.477813114080004, -6.495952174506119, nan, nan, nan, -7.327276260680452, nan, nan, nan, nan, nan, nan, -6.4360860644722475, nan, -6.739302957071822, -6.620344252274687, nan, nan, -7.342053382683826, nan, nan, nan, -6.813502475183624, -6.299168979184704, nan, nan, -7.061425074297989, nan, -5.773901271518503, nan, nan, -7.759495288610495, -7.293918710005261, -5.164805336225902, nan, nan, nan, nan, nan, -6.5030440314757545, nan, nan, nan, nan, nan, nan, -6.384903928378213, nan, -7.7426075194097645, nan, nan, nan, -6.693585731491109, nan, nan, nan, nan, -6.771954742159877, nan, nan, -7.915242555896809, nan, nan, -6.317201159457019, -7.630453791704001, nan, -6.534738599371669, nan, nan, nan, -6.583623532523205, nan, -5.833878627455628, nan, nan, -7.124785351423516, nan, nan, nan, nan, nan, nan, nan, -6.974027607755967, nan, nan, -6.507767808873869, -7.07367509848339, nan, nan, -6.996616570963682, nan, nan, nan, nan, nan, nan, nan, nan, nan, -7.418158532656198, -7.484831295607282, -7.482545387943841, -6.906082474082935, nan, nan, nan, nan, -7.105790650402792, -8.155656322021034, nan, nan, nan, nan, nan, nan, nan, nan, nan, nan, nan, nan, nan, nan, nan, nan, nan, -7.042938522975961, -7.413375974158198, nan, nan, nan, nan, nan, nan, -6.994090849523267, nan, nan, nan, -6.535157746532564, nan, nan, nan, nan, nan, nan, nan, nan, nan, nan, nan, nan, nan, nan, nan, nan, nan, -7.46469034767263, nan, nan, -8.472193641099159, nan, -7.316818398476609, nan, nan, nan, nan, nan, nan, nan, nan, nan, nan, nan, nan, nan, -7.124072437581559, -7.621081871158111, nan, nan, nan, nan, -7.5903746783508845, nan, -6.76132154536757, nan, nan, nan, -7.271475055397208, nan, nan, nan, nan, nan, nan, nan, nan, nan, nan, nan, nan, nan, nan, nan, nan, nan, nan, nan, -8.255758145797417, -6.310691801166498, nan, nan, nan, nan, -7.3075891148250145, nan, nan, nan, nan, nan, nan, nan, nan, nan, nan, nan, nan, nan, nan, nan, -8.333917805548376, nan, nan, -7.296582116935124, nan, nan, nan, -7.5706519811759225, nan, nan, nan, nan, nan, nan, nan, nan, nan, nan, nan, nan, -7.373591110768092, nan, nan, nan, nan, nan, nan, nan, nan, nan, nan, -6.311706474847402, nan, nan, nan, nan, nan, nan, nan, nan, -8.570267286699906, -7.764743296282475, nan, nan, nan, nan, nan, -8.144558427236914, -6.950431398641365, nan, nan, nan, nan, nan, nan, nan, nan, nan, -6.650097903374695, nan, nan, nan, nan, -8.794277230786085, nan, -7.438402511856436, -7.19132416465763, nan, nan, nan, nan, nan, nan, nan, nan, nan, nan, nan, nan, nan, nan, nan, nan, nan, nan, nan, nan, -7.383162941423935, nan, nan, -9.242717255013817, -6.524427661404665, nan, nan, nan, -7.197402994328144, nan, -7.533421740784625, nan, -8.090441008431089, nan, nan, nan, nan, nan, -7.5924533560723715, nan, nan, nan, nan, nan, nan, nan, nan, nan, nan, nan, -6.993295014332601, nan, -7.656933273874152, nan, nan, nan, nan, nan, nan, nan, nan, nan, -7.379854918316114, -6.977291067186793, nan, nan, -8.680201899389235, nan, -7.879368276945829, nan, nan, nan, nan, -7.6114646321313755, nan, -7.5294829014839095, -7.075963061488881, -6.689275007256416, nan, nan, -6.696788739356793, -8.047336490153569, nan, nan, nan, nan, nan, -8.247890855928638, nan, nan, nan, -8.163907420317033, nan, nan, nan, nan, nan, nan, nan, nan, nan, nan, nan, nan, nan, nan, nan, nan, 0.0, 0.0]] caption="Water Vapor Number Density"
  out "CH3 RingBuffer short":dbl[][](array[numeric])=[[95.56, 39.56, 42.56, 48.56, 64.56, 87.56, 139.56, 208.56, 315.56, 391.56, 464.56, 503.56, 501.56, 545.56, 575.56, 544.56, 504.56, 504.56, 483.56, 432.56, 381.56, 345.56, 328.56, 311.56, 279.56, 293.56, 273.56, 268.56, 256.56, 284.56, 271.56, 284.56, 285.56, 243.56, 257.56, 222.56, 269.56, 211.56, 174.56, 220.56, 219.56, 194.56, 194.56, 170.56, 179.56, 170.56, 152.56, 163.56, 154.56, 144.56, 119.56, 115.56, 127.56, 128.56, 127.56, 106.56, 104.56, 125.56, 84.56, 90.56, 85.56, 66.56, 76.56, 78.56, 94.56, 71.56, 61.56, 51.56, 50.56, 56.56, 75.56, 43.56, 40.56, 24.56, 48.56, 41.56, 25.56, 31.56, 32.56, 37.56, 26.56, 21.56, 26.56, 21.56, 23.56, 26.56, 29.56, 34.56, 14.559999999999999, 31.56, 16.56, 16.56, 18.56, 13.559999999999999, 21.56, 19.56, 7.559999999999999, 15.559999999999999, 16.56, 15.559999999999999, 15.559999999999999, 30.56, 18.56, 16.56, 4.559999999999999, 12.559999999999999, 8.559999999999999, 5.559999999999999, 13.559999999999999, 10.559999999999999, 14.559999999999999, 7.559999999999999, 13.559999999999999, 2.5599999999999987, 7.559999999999999, 11.559999999999999, 9.559999999999999, 8.559999999999999, 10.559999999999999, 7.559999999999999, 9.559999999999999, 8.559999999999999, 1.5599999999999987, 3.5599999999999987, -1.4400000000000013, 18.56, 2.5599999999999987, 2.5599999999999987, 1.5599999999999987, 7.559999999999999, 11.559999999999999, 13.559999999999999, 4.559999999999999, 6.559999999999999, 1.5599999999999987, 13.559999999999999, 5.559999999999999, 7.559999999999999, 1.5599999999999987, 3.5599999999999987, 3.5599999999999987, 0.5599999999999987, 6.559999999999999, 14.559999999999999, -5.440000000000001, 4.559999999999999, -0.4400000000000013, -2.4400000000000013, -1.4400000000000013, 2.5599999999999987, 10.559999999999999, 14.559999999999999, 10.559999999999999, 9.559999999999999, 4.559999999999999, -2.4400000000000013, 7.559999999999999, -5.440000000000001, -0.4400000000000013, 3.5599999999999987, -2.4400000000000013, -3.4400000000000013, 9.559999999999999, -0.4400000000000013, 7.559999999999999, 2.5599999999999987, 0.5599999999999987, 1.5599999999999987, 8.559999999999999, -2.4400000000000013, -3.4400000000000013, -2.4400000000000013, 1.5599999999999987, -0.4400000000000013, -2.4400000000000013, -3.4400000000000013, 9.559999999999999, -4.440000000000001, 9.559999999999999, 5.559999999999999, -2.4400000000000013, 6.559999999999999, 0.5599999999999987, 1.5599999999999987, -7.440000000000001, 8.559999999999999, -0.4400000000000013, 4.559999999999999, 2.5599999999999987, 2.5599999999999987, 2.5599999999999987, -7.440000000000001, -0.4400000000000013, 0.5599999999999987, 2.5599999999999987, -4.440000000000001, -2.4400000000000013, -6.440000000000001, -1.4400000000000013, 1.5599999999999987, 4.559999999999999, -1.4400000000000013, 3.5599999999999987, -1.4400000000000013, -4.440000000000001, 2.5599999999999987, 9.559999999999999, 7.559999999999999, 7.559999999999999, 1.5599999999999987, -4.440000000000001, -5.440000000000001, -8.440000000000001, 2.5599999999999987, 3.5599999999999987, -9.440000000000001, 3.5599999999999987, 1.5599999999999987, 1.5599999999999987, 6.559999999999999, 6.559999999999999, -1.4400000000000013, 1.5599999999999987, 2.5599999999999987, 7.559999999999999, -1.4400000000000013, -2.4400000000000013, 3.5599999999999987, -3.4400000000000013, -1.4400000000000013, 7.559999999999999, 0.5599999999999987, 3.5599999999999987, -5.440000000000001, 6.559999999999999, -3.4400000000000013, 0.5599999999999987, 0.5599999999999987, -0.4400000000000013, 10.559999999999999, 1.5599999999999987, -0.4400000000000013, -2.4400000000000013, -1.4400000000000013, 2.5599999999999987, 7.559999999999999, 12.559999999999999, 2.5599999999999987, -3.4400000000000013, 8.559999999999999, -1.4400000000000013, 2.5599999999999987, -2.4400000000000013, -2.4400000000000013, 6.559999999999999, -5.440000000000001, -3.4400000000000013, 10.559999999999999, 1.5599999999999987, -2.4400000000000013, 0.5599999999999987, 1.5599999999999987, 5.559999999999999, 1.5599999999999987, 3.5599999999999987, 1.5599999999999987, -2.4400000000000013, 1.5599999999999987, -3.4400000000000013, -0.4400000000000013, -4.440000000000001, 0.5599999999999987, 3.5599999999999987, -3.4400000000000013, 3.5599999999999987, -4.440000000000001, -5.440000000000001, -0.4400000000000013, -0.4400000000000013, 4.559999999999999, -0.4400000000000013, -1.4400000000000013, 8.559999999999999, -1.4400000000000013, 1.5599999999999987, -1.4400000000000013, -0.4400000000000013, 5.559999999999999, -3.4400000000000013, 7.559999999999999, 2.5599999999999987, 9.559999999999999, -3.4400000000000013, -1.4400000000000013, -1.4400000000000013, -1.4400000000000013, 2.5599999999999987, -4.440000000000001, -2.4400000000000013, -5.440000000000001, 3.5599999999999987, -4.440000000000001, -5.440000000000001, 3.5599999999999987, 3.5599999999999987, -5.440000000000001, 4.559999999999999, 1.5599999999999987, 3.5599999999999987, -0.4400000000000013, -5.440000000000001, 11.559999999999999, 2.5599999999999987, 1.5599999999999987, -8.440000000000001, 6.559999999999999, -2.4400000000000013, -3.4400000000000013, 4.559999999999999, 3.5599999999999987, 6.559999999999999, -2.4400000000000013, 5.559999999999999, -3.4400000000000013, 10.559999999999999, -1.4400000000000013, -2.4400000000000013, -1.4400000000000013, -5.440000000000001, 3.5599999999999987, -4.440000000000001, -2.4400000000000013, 6.559999999999999, 8.559999999999999, -4.440000000000001, 1.5599999999999987, 6.559999999999999, 3.5599999999999987, 2.5599999999999987, 5.559999999999999, 4.559999999999999, 5.559999999999999, 2.5599999999999987, 1.5599999999999987, 5.559999999999999, -3.4400000000000013, -7.440000000000001, 3.5599999999999987, 2.5599999999999987, 0.5599999999999987, 1.5599999999999987, 1.5599999999999987, -6.440000000000001, -0.4400000000000013, -0.4400000000000013, -0.4400000000000013, 1.5599999999999987, 2.5599999999999987, -1.4400000000000013, 9.559999999999999, 2.5599999999999987, -3.4400000000000013, 9.559999999999999, 1.5599999999999987, 2.5599999999999987, 2.5599999999999987, 2.5599999999999987, -1.4400000000000013, -3.4400000000000013, -0.4400000000000013, 6.559999999999999, -7.440000000000001, -0.4400000000000013, 3.5599999999999987, 0.5599999999999987, 2.5599999999999987, 7.559999999999999, -3.4400000000000013, 3.5599999999999987, 8.559999999999999, 3.5599999999999987, 3.5599999999999987, -0.4400000000000013, -1.4400000000000013, 3.5599999999999987, -1.4400000000000013, 3.5599999999999987, 1.5599999999999987, -1.4400000000000013, 2.5599999999999987, -4.440000000000001, 0.5599999999999987, 6.559999999999999, -0.4400000000000013, -2.4400000000000013, 5.559999999999999, -3.4400000000000013, 4.559999999999999, 2.5599999999999987, 8.559999999999999, -1.4400000000000013, -2.4400000000000013, -2.4400000000000013, 16.56, -4.440000000000001, 2.5599999999999987, -1.4400000000000013, 8.559999999999999, 0.5599999999999987, -9.440000000000001, -4.440000000000001, 4.559999999999999, -0.4400000000000013, 6.559999999999999, -2.4400000000000013, 1.5599999999999987, -1.4400000000000013, -6.440000000000001, -3.4400000000000013, 6.559999999999999, -4.440000000000001, -1.4400000000000013, 3.5599999999999987, 2.5599999999999987, -0.4400000000000013, -0.4400000000000013, -1.4400000000000013, -2.4400000000000013, -0.4400000000000013, 6.559999999999999, 0.5599999999999987, -5.440000000000001, 4.559999999999999, -5.440000000000001, -0.4400000000000013, 0.5599999999999987, 0.5599999999999987, -0.4400000000000013, 0.5599999999999987, 5.559999999999999, -7.440000000000001, -5.440000000000001, -1.4400000000000013, 3.5599999999999987, -7.440000000000001, 4.559999999999999, -3.4400000000000013, 6.559999999999999, 4.559999999999999, -3.4400000000000013, -5.440000000000001, 2.5599999999999987, -1.4400000000000013, -4.440000000000001, 3.5599999999999987, 3.5599999999999987, -3.4400000000000013, 6.559999999999999, -3.4400000000000013, -0.4400000000000013, 4.559999999999999, 3.5599999999999987, -3.4400000000000013, 2.5599999999999987, 1.5599999999999987, -3.4400000000000013, -6.440000000000001, -5.440000000000001, 3.5599999999999987, -2.4400000000000013, 1.5599999999999987, 6.559999999999999, -7.440000000000001, -1.4400000000000013, -7.440000000000001, 4.559999999999999, -2.4400000000000013, 0.5599999999999987, 11.559999999999999, 3.5599999999999987, 4.559999999999999, -10.440000000000001, -0.4400000000000013, 3.5599999999999987, 2.5599999999999987, -0.4400000000000013, 1.5599999999999987, 4.559999999999999, 7.559999999999999, -1.4400000000000013, -6.440000000000001, 0.5599999999999987, 4.559999999999999, -0.4400000000000013, -4.440000000000001, -1.4400000000000013, 4.559999999999999, 5.559999999999999, -3.4400000000000013, 2.5599999999999987, -4.440000000000001, 4.559999999999999, 2.5599999999999987, -0.4400000000000013, -5.440000000000001, 4.559999999999999, 5.559999999999999, 2.5599999999999987, 1.5599999999999987, 2.5599999999999987, 2.5599999999999987, 2.5599999999999987, 4.559999999999999, 2.5599999999999987, 1.5599999999999987, -6.440000000000001, 1.5599999999999987, 9.559999999999999, 3.5599999999999987, -1.4400000000000013, 8.559999999999999, 7.559999999999999, 2.5599999999999987, 0.5599999999999987, 9.559999999999999, -1.4400000000000013, -3.4400000000000013, -2.4400000000000013, -1.4400000000000013, 8.559999999999999, -0.4400000000000013, -4.440000000000001, 1.5599999999999987, 2.5599999999999987, -5.440000000000001, 0.5599999999999987, 0.5599999999999987, -1.4400000000000013, 0.5599999999999987, -2.4400000000000013, -4.440000000000001, 0.5599999999999987, 0.5599999999999987, 9.559999999999999, -3.4400000000000013, 7.559999999999999, 2.5599999999999987, 2.5599999999999987, 2.5599999999999987, -2.4400000000000013, -1.4400000000000013, 4.559999999999999, 2.5599999999999987, -5.440000000000001, -6.440000000000001, -1.4400000000000013, -1.4400000000000013, 1.5599999999999987, -0.4400000000000013, -17.44], [76.12, 28.119999999999997, 40.12, 58.12, 70.12, 116.12, 132.12, 257.12, 262.12, 355.12, 466.12, 503.12, 544.12, 558.12, 548.12, 556.12, 557.12, 510.12, 474.12, 512.12, 387.12, 341.12, 329.12, 329.12, 291.12, 265.12, 291.12, 283.12, 296.12, 259.12, 234.12, 254.12, 226.12, 239.12, 234.12, 246.12, 237.12, 233.12, 235.12, 175.12, 211.12, 186.12, 165.12, 148.12, 171.12, 175.12, 127.12, 122.12, 136.12, 135.12, 122.12, 117.12, 133.12, 116.12, 127.12, 101.12, 97.12, 96.12, 85.12, 80.12, 84.12, 88.12, 81.12, 56.12, 65.12, 67.12, 74.12, 62.12, 55.12, 50.12, 46.12, 48.12, 53.12, 43.12, 40.12, 33.12, 38.12, 31.119999999999997, 31.119999999999997, 28.119999999999997, 28.119999999999997, 29.119999999999997, 18.119999999999997, 31.119999999999997, 27.119999999999997, 23.119999999999997, 33.12, 34.12, 28.119999999999997, 24.119999999999997, 29.119999999999997, 15.12, 11.12, 16.119999999999997, 16.119999999999997, 22.119999999999997, 19.119999999999997, 10.12, 20.119999999999997, 23.119999999999997, 10.12, 19.119999999999997, 14.12, 13.12, 10.12, 15.12, 8.12, 15.12, 21.119999999999997, 3.119999999999999, -1.8800000000000008, 13.12, 13.12, 15.12, 9.12, 3.119999999999999, 20.119999999999997, 17.119999999999997, 9.12, 24.119999999999997, 2.119999999999999, 14.12, 5.119999999999999, 7.119999999999999, -2.880000000000001, 10.12, 11.12, 7.119999999999999, 2.119999999999999, 20.119999999999997, 10.12, 2.119999999999999, 12.12, 12.12, -0.8800000000000008, 8.12, 15.12, 6.119999999999999, 0.11999999999999922, -1.8800000000000008, 11.12, 12.12, 10.12, 5.119999999999999, 7.119999999999999, 7.119999999999999, 7.119999999999999, 7.119999999999999, 5.119999999999999, 11.12, 7.119999999999999, 4.119999999999999, 5.119999999999999, 2.119999999999999, 3.119999999999999, 12.12, 3.119999999999999, -4.880000000000001, 10.12, 8.12, 6.119999999999999, 3.119999999999999, 8.12, -3.880000000000001, 0.11999999999999922, 10.12, 12.12, 3.119999999999999, 11.12, -3.880000000000001, -0.8800000000000008, 5.119999999999999, 8.12, -4.880000000000001, 8.12, 5.119999999999999, 15.12, 3.119999999999999, 6.119999999999999, 10.12, 8.12, -2.880000000000001, 2.119999999999999, 13.12, 3.119999999999999, 8.12, 4.119999999999999, -1.8800000000000008, -0.8800000000000008, -0.8800000000000008, -5.880000000000001, 7.119999999999999, -5.880000000000001, 7.119999999999999, 11.12, -1.8800000000000008, -2.880000000000001, 5.119999999999999, -3.880000000000001, 0.11999999999999922, 7.119999999999999, 2.119999999999999, 0.11999999999999922, -3.880000000000001, 6.119999999999999, 7.119999999999999, 4.119999999999999, 1.1199999999999992, 4.119999999999999, 10.12, 1.1199999999999992, 2.119999999999999, 2.119999999999999, 3.119999999999999, 2.119999999999999, 8.12, 9.12, 3.119999999999999, -1.8800000000000008, -1.8800000000000008, -0.8800000000000008, 3.119999999999999, 0.11999999999999922, 7.119999999999999, 2.119999999999999, 8.12, 4.119999999999999, 0.11999999999999922, 2.119999999999999, -1.8800000000000008, 2.119999999999999, 1.1199999999999992, 6.119999999999999, 2.119999999999999, -2.880000000000001, 2.119999999999999, 1.1199999999999992, 4.119999999999999, 7.119999999999999, 2.119999999999999, 1.1199999999999992, 5.119999999999999, 4.119999999999999, 2.119999999999999, 2.119999999999999, 1.1199999999999992, 2.119999999999999, 8.12, 16.119999999999997, 7.119999999999999, -5.880000000000001, -2.880000000000001, 5.119999999999999, 6.119999999999999, 7.119999999999999, 1.1199999999999992, 11.12, 6.119999999999999, 1.1199999999999992, 7.119999999999999, 5.119999999999999, 1.1199999999999992, 8.12, 5.119999999999999, -5.880000000000001, 3.119999999999999, 4.119999999999999, 1.1199999999999992, -4.880000000000001, 2.119999999999999, -0.8800000000000008, -1.8800000000000008, -1.8800000000000008, 3.119999999999999, -3.880000000000001, 0.11999999999999922, 3.119999999999999, 0.11999999999999922, 1.1199999999999992, 3.119999999999999, -2.880000000000001, 1.1199999999999992, -0.8800000000000008, 6.119999999999999, 5.119999999999999, -4.880000000000001, 3.119999999999999, -2.880000000000001, 4.119999999999999, 1.1199999999999992, 6.119999999999999, 4.119999999999999, -2.880000000000001, -0.8800000000000008, -0.8800000000000008, 8.12, 1.1199999999999992, 4.119999999999999, 2.119999999999999, 5.119999999999999, 6.119999999999999, 4.119999999999999, 6.119999999999999, 8.12, -5.880000000000001, -1.8800000000000008, 4.119999999999999, 5.119999999999999, 6.119999999999999, -0.8800000000000008, 4.119999999999999, 2.119999999999999, 5.119999999999999, -1.8800000000000008, 5.119999999999999, 1.1199999999999992, -0.8800000000000008, 4.119999999999999, -0.8800000000000008, 9.12, 7.119999999999999, -4.880000000000001, 2.119999999999999, 10.12, -5.880000000000001, -2.880000000000001, 4.119999999999999, 7.119999999999999, 9.12, 1.1199999999999992, -10.88, 5.119999999999999, 4.119999999999999, 2.119999999999999, -0.8800000000000008, -3.880000000000001, 3.119999999999999, 2.119999999999999, 2.119999999999999, -4.880000000000001, 10.12, 1.1199999999999992, 0.11999999999999922, 1.1199999999999992, -2.880000000000001, -5.880000000000001, 2.119999999999999, 11.12, 3.119999999999999, 2.119999999999999, 2.119999999999999, 9.12, 6.119999999999999, 9.12, 3.119999999999999, 3.119999999999999, -3.880000000000001, 3.119999999999999, -0.8800000000000008, 0.11999999999999922, 5.119999999999999, 5.119999999999999, 1.1199999999999992, 5.119999999999999, 12.12, 9.12, 6.119999999999999, 4.119999999999999, 3.119999999999999, 1.1199999999999992, 6.119999999999999, -0.8800000000000008, -0.8800000000000008, 3.119999999999999, 3.119999999999999, 5.119999999999999, 1.1199999999999992, -1.8800000000000008, -2.880000000000001, 0.11999999999999922, -4.880000000000001, -0.8800000000000008, 0.11999999999999922, 1.1199999999999992, -3.880000000000001, 2.119999999999999, 3.119999999999999, 6.119999999999999, 5.119999999999999, 1.1199999999999992, 3.119999999999999, -0.8800000000000008, -0.8800000000000008, 2.119999999999999, 6.119999999999999, 2.119999999999999, 7.119999999999999, 1.1199999999999992, 0.11999999999999922, 5.119999999999999, -2.880000000000001, -3.880000000000001, -0.8800000000000008, 2.119999999999999, 2.119999999999999, 6.119999999999999, 8.12, 8.12, 2.119999999999999, 6.119999999999999, 6.119999999999999, -2.880000000000001, -3.880000000000001, 5.119999999999999, 4.119999999999999, -0.8800000000000008, 5.119999999999999, 2.119999999999999, 6.119999999999999, -8.88, 5.119999999999999, 10.12, 1.1199999999999992, -1.8800000000000008, -1.8800000000000008, -1.8800000000000008, 2.119999999999999, -3.880000000000001, -2.880000000000001, 7.119999999999999, 7.119999999999999, 6.119999999999999, 6.119999999999999, -1.8800000000000008, 1.1199999999999992, 2.119999999999999, -1.8800000000000008, -0.8800000000000008, -4.880000000000001, -1.8800000000000008, 4.119999999999999, -1.8800000000000008, 0.11999999999999922, 0.11999999999999922, -0.8800000000000008, 2.119999999999999, 1.1199999999999992, -0.8800000000000008, 1.1199999999999992, -0.8800000000000008, 0.11999999999999922, -3.880000000000001, 3.119999999999999, 7.119999999999999, 7.119999999999999, -1.8800000000000008, -3.880000000000001, 0.11999999999999922, 2.119999999999999, 4.119999999999999, 0.11999999999999922, 8.12, 7.119999999999999, 0.11999999999999922, 5.119999999999999, 2.119999999999999, 2.119999999999999, 2.119999999999999, 7.119999999999999, 0.11999999999999922, 8.12, 9.12, 1.1199999999999992, -1.8800000000000008, 9.12, 4.119999999999999, 3.119999999999999, -1.8800000000000008, -2.880000000000001, -0.8800000000000008, 5.119999999999999, 1.1199999999999992, 10.12, 14.12, 3.119999999999999, 7.119999999999999, -8.88, 4.119999999999999, 1.1199999999999992, -1.8800000000000008, -1.8800000000000008, 7.119999999999999, 6.119999999999999, 6.119999999999999, -2.880000000000001, 2.119999999999999, 6.119999999999999, 1.1199999999999992, 1.1199999999999992, -0.8800000000000008, -0.8800000000000008, 11.12, 4.119999999999999, 7.119999999999999, 9.12, 1.1199999999999992, 4.119999999999999, 4.119999999999999, -0.8800000000000008, 0.11999999999999922, 1.1199999999999992, 0.11999999999999922, -2.880000000000001, -4.880000000000001, 7.119999999999999, -0.8800000000000008, 3.119999999999999, 7.119999999999999, -1.8800000000000008, -0.8800000000000008, 9.12, -0.8800000000000008, 5.119999999999999, 12.12, 7.119999999999999, 2.119999999999999, -7.880000000000001, 2.119999999999999, 5.119999999999999, 2.119999999999999, 6.119999999999999, 1.1199999999999992, -0.8800000000000008, -5.880000000000001, -5.880000000000001, -0.8800000000000008, -4.880000000000001, 0.11999999999999922, 8.12, 0.11999999999999922, 0.11999999999999922, 0.11999999999999922, -2.880000000000001, 10.12, -3.880000000000001, 3.119999999999999, -5.880000000000001, -6.880000000000001, -1.8800000000000008, 0.11999999999999922, -1.8800000000000008, 0.11999999999999922, -2.880000000000001, 5.119999999999999, 3.119999999999999, 5.119999999999999, 5.119999999999999, 3.119999999999999, -5.880000000000001, -15.88], [76.12, 28.119999999999997, 40.12, 58.12, 70.12, 116.12, 132.12, 257.12, 262.12, 355.12, 466.12, 503.12, 544.12, 558.12, 548.12, 556.12, 557.12, 510.12, 474.12, 512.12, 387.12, 341.12, 329.12, 329.12, 291.12, 265.12, 291.12, 283.12, 296.12, 259.12, 234.12, 254.12, 226.12, 239.12, 234.12, 246.12, 237.12, 233.12, 235.12, 175.12, 211.12, 186.12, 165.12, 148.12, 171.12, 175.12, 127.12, 122.12, 136.12, 135.12, 122.12, 117.12, 133.12, 116.12, 127.12, 101.12, 97.12, 96.12, 85.12, 80.12, 84.12, 88.12, 81.12, 56.12, 65.12, 67.12, 74.12, 62.12, 55.12, 50.12, 46.12, 48.12, 53.12, 43.12, 40.12, 33.12, 38.12, 31.119999999999997, 31.119999999999997, 28.119999999999997, 28.119999999999997, 29.119999999999997, 18.119999999999997, 31.119999999999997, 27.119999999999997, 23.119999999999997, 33.12, 34.12, 28.119999999999997, 24.119999999999997, 29.119999999999997, 15.12, 11.12, 16.119999999999997, 16.119999999999997, 22.119999999999997, 19.119999999999997, 10.12, 20.119999999999997, 23.119999999999997, 10.12, 19.119999999999997, 14.12, 13.12, 10.12, 15.12, 8.12, 15.12, 21.119999999999997, 3.119999999999999, -1.8800000000000008, 13.12, 13.12, 15.12, 9.12, 3.119999999999999, 20.119999999999997, 17.119999999999997, 9.12, 24.119999999999997, 2.119999999999999, 14.12, 5.119999999999999, 7.119999999999999, -2.880000000000001, 10.12, 11.12, 7.119999999999999, 2.119999999999999, 20.119999999999997, 10.12, 2.119999999999999, 12.12, 12.12, -0.8800000000000008, 8.12, 15.12, 6.119999999999999, 0.11999999999999922, -1.8800000000000008, 11.12, 12.12, 10.12, 5.119999999999999, 7.119999999999999, 7.119999999999999, 7.119999999999999, 7.119999999999999, 5.119999999999999, 11.12, 7.119999999999999, 4.119999999999999, 5.119999999999999, 2.119999999999999, 3.119999999999999, 12.12, 3.119999999999999, -4.880000000000001, 10.12, 8.12, 6.119999999999999, 3.119999999999999, 8.12, -3.880000000000001, 0.11999999999999922, 10.12, 12.12, 3.119999999999999, 11.12, -3.880000000000001, -0.8800000000000008, 5.119999999999999, 8.12, -4.880000000000001, 8.12, 5.119999999999999, 15.12, 3.119999999999999, 6.119999999999999, 10.12, 8.12, -2.880000000000001, 2.119999999999999, 13.12, 3.119999999999999, 8.12, 4.119999999999999, -1.8800000000000008, -0.8800000000000008, -0.8800000000000008, -5.880000000000001, 7.119999999999999, -5.880000000000001, 7.119999999999999, 11.12, -1.8800000000000008, -2.880000000000001, 5.119999999999999, -3.880000000000001, 0.11999999999999922, 7.119999999999999, 2.119999999999999, 0.11999999999999922, -3.880000000000001, 6.119999999999999, 7.119999999999999, 4.119999999999999, 1.1199999999999992, 4.119999999999999, 10.12, 1.1199999999999992, 2.119999999999999, 2.119999999999999, 3.119999999999999, 2.119999999999999, 8.12, 9.12, 3.119999999999999, -1.8800000000000008, -1.8800000000000008, -0.8800000000000008, 3.119999999999999, 0.11999999999999922, 7.119999999999999, 2.119999999999999, 8.12, 4.119999999999999, 0.11999999999999922, 2.119999999999999, -1.8800000000000008, 2.119999999999999, 1.1199999999999992, 6.119999999999999, 2.119999999999999, -2.880000000000001, 2.119999999999999, 1.1199999999999992, 4.119999999999999, 7.119999999999999, 2.119999999999999, 1.1199999999999992, 5.119999999999999, 4.119999999999999, 2.119999999999999, 2.119999999999999, 1.1199999999999992, 2.119999999999999, 8.12, 16.119999999999997, 7.119999999999999, -5.880000000000001, -2.880000000000001, 5.119999999999999, 6.119999999999999, 7.119999999999999, 1.1199999999999992, 11.12, 6.119999999999999, 1.1199999999999992, 7.119999999999999, 5.119999999999999, 1.1199999999999992, 8.12, 5.119999999999999, -5.880000000000001, 3.119999999999999, 4.119999999999999, 1.1199999999999992, -4.880000000000001, 2.119999999999999, -0.8800000000000008, -1.8800000000000008, -1.8800000000000008, 3.119999999999999, -3.880000000000001, 0.11999999999999922, 3.119999999999999, 0.11999999999999922, 1.1199999999999992, 3.119999999999999, -2.880000000000001, 1.1199999999999992, -0.8800000000000008, 6.119999999999999, 5.119999999999999, -4.880000000000001, 3.119999999999999, -2.880000000000001, 4.119999999999999, 1.1199999999999992, 6.119999999999999, 4.119999999999999, -2.880000000000001, -0.8800000000000008, -0.8800000000000008, 8.12, 1.1199999999999992, 4.119999999999999, 2.119999999999999, 5.119999999999999, 6.119999999999999, 4.119999999999999, 6.119999999999999, 8.12, -5.880000000000001, -1.8800000000000008, 4.119999999999999, 5.119999999999999, 6.119999999999999, -0.8800000000000008, 4.119999999999999, 2.119999999999999, 5.119999999999999, -1.8800000000000008, 5.119999999999999, 1.1199999999999992, -0.8800000000000008, 4.119999999999999, -0.8800000000000008, 9.12, 7.119999999999999, -4.880000000000001, 2.119999999999999, 10.12, -5.880000000000001, -2.880000000000001, 4.119999999999999, 7.119999999999999, 9.12, 1.1199999999999992, -10.88, 5.119999999999999, 4.119999999999999, 2.119999999999999, -0.8800000000000008, -3.880000000000001, 3.119999999999999, 2.119999999999999, 2.119999999999999, -4.880000000000001, 10.12, 1.1199999999999992, 0.11999999999999922, 1.1199999999999992, -2.880000000000001, -5.880000000000001, 2.119999999999999, 11.12, 3.119999999999999, 2.119999999999999, 2.119999999999999, 9.12, 6.119999999999999, 9.12, 3.119999999999999, 3.119999999999999, -3.880000000000001, 3.119999999999999, -0.8800000000000008, 0.11999999999999922, 5.119999999999999, 5.119999999999999, 1.1199999999999992, 5.119999999999999, 12.12, 9.12, 6.119999999999999, 4.119999999999999, 3.119999999999999, 1.1199999999999992, 6.119999999999999, -0.8800000000000008, -0.8800000000000008, 3.119999999999999, 3.119999999999999, 5.119999999999999, 1.1199999999999992, -1.8800000000000008, -2.880000000000001, 0.11999999999999922, -4.880000000000001, -0.8800000000000008, 0.11999999999999922, 1.1199999999999992, -3.880000000000001, 2.119999999999999, 3.119999999999999, 6.119999999999999, 5.119999999999999, 1.1199999999999992, 3.119999999999999, -0.8800000000000008, -0.8800000000000008, 2.119999999999999, 6.119999999999999, 2.119999999999999, 7.119999999999999, 1.1199999999999992, 0.11999999999999922, 5.119999999999999, -2.880000000000001, -3.880000000000001, -0.8800000000000008, 2.119999999999999, 2.119999999999999, 6.119999999999999, 8.12, 8.12, 2.119999999999999, 6.119999999999999, 6.119999999999999, -2.880000000000001, -3.880000000000001, 5.119999999999999, 4.119999999999999, -0.8800000000000008, 5.119999999999999, 2.119999999999999, 6.119999999999999, -8.88, 5.119999999999999, 10.12, 1.1199999999999992, -1.8800000000000008, -1.8800000000000008, -1.8800000000000008, 2.119999999999999, -3.880000000000001, -2.880000000000001, 7.119999999999999, 7.119999999999999, 6.119999999999999, 6.119999999999999, -1.8800000000000008, 1.1199999999999992, 2.119999999999999, -1.8800000000000008, -0.8800000000000008, -4.880000000000001, -1.8800000000000008, 4.119999999999999, -1.8800000000000008, 0.11999999999999922, 0.11999999999999922, -0.8800000000000008, 2.119999999999999, 1.1199999999999992, -0.8800000000000008, 1.1199999999999992, -0.8800000000000008, 0.11999999999999922, -3.880000000000001, 3.119999999999999, 7.119999999999999, 7.119999999999999, -1.8800000000000008, -3.880000000000001, 0.11999999999999922, 2.119999999999999, 4.119999999999999, 0.11999999999999922, 8.12, 7.119999999999999, 0.11999999999999922, 5.119999999999999, 2.119999999999999, 2.119999999999999, 2.119999999999999, 7.119999999999999, 0.11999999999999922, 8.12, 9.12, 1.1199999999999992, -1.8800000000000008, 9.12, 4.119999999999999, 3.119999999999999, -1.8800000000000008, -2.880000000000001, -0.8800000000000008, 5.119999999999999, 1.1199999999999992, 10.12, 14.12, 3.119999999999999, 7.119999999999999, -8.88, 4.119999999999999, 1.1199999999999992, -1.8800000000000008, -1.8800000000000008, 7.119999999999999, 6.119999999999999, 6.119999999999999, -2.880000000000001, 2.119999999999999, 6.119999999999999, 1.1199999999999992, 1.1199999999999992, -0.8800000000000008, -0.8800000000000008, 11.12, 4.119999999999999, 7.119999999999999, 9.12, 1.1199999999999992, 4.119999999999999, 4.119999999999999, -0.8800000000000008, 0.11999999999999922, 1.1199999999999992, 0.11999999999999922, -2.880000000000001, -4.880000000000001, 7.119999999999999, -0.8800000000000008, 3.119999999999999, 7.119999999999999, -1.8800000000000008, -0.8800000000000008, 9.12, -0.8800000000000008, 5.119999999999999, 12.12, 7.119999999999999, 2.119999999999999, -7.880000000000001, 2.119999999999999, 5.119999999999999, 2.119999999999999, 6.119999999999999, 1.1199999999999992, -0.8800000000000008, -5.880000000000001, -5.880000000000001, -0.8800000000000008, -4.880000000000001, 0.11999999999999922, 8.12, 0.11999999999999922, 0.11999999999999922, 0.11999999999999922, -2.880000000000001, 10.12, -3.880000000000001, 3.119999999999999, -5.880000000000001, -6.880000000000001, -1.8800000000000008, 0.11999999999999922, -1.8800000000000008, 0.11999999999999922, -2.880000000000001, 5.119999999999999, 3.119999999999999, 5.119999999999999, 5.119999999999999, 3.119999999999999, -5.880000000000001, -15.88], [70.08, 46.08, 28.08, 50.08, 46.08, 91.08, 142.07999999999998, 203.07999999999998, 328.08, 371.08, 455.08, 481.08, 539.08, 538.08, 552.08, 571.08, 535.08, 512.08, 483.08, 480.08, 372.08, 326.08, 354.08, 282.08, 289.08, 290.08, 252.07999999999998, 250.07999999999998, 287.08, 265.08, 240.07999999999998, 248.07999999999998, 240.07999999999998, 269.08, 232.07999999999998, 217.07999999999998, 218.07999999999998, 191.07999999999998, 221.07999999999998, 229.07999999999998, 181.07999999999998, 215.07999999999998, 177.07999999999998, 168.07999999999998, 183.07999999999998, 157.07999999999998, 147.07999999999998, 153.07999999999998, 157.07999999999998, 135.07999999999998, 133.07999999999998, 123.08, 107.08, 124.08, 130.07999999999998, 100.08, 74.08, 78.08, 95.08, 77.08, 83.08, 56.08, 78.08, 72.08, 58.08, 45.08, 50.08, 45.08, 49.08, 52.08, 46.08, 50.08, 41.08, 32.08, 29.08, 48.08, 32.08, 23.08, 26.08, 21.08, 25.08, 26.08, 18.08, 23.08, 32.08, 17.08, 20.08, 11.079999999999998, 17.08, 8.079999999999998, 17.08, 10.079999999999998, 20.08, 20.08, 21.08, 5.079999999999998, 12.079999999999998, 21.08, 4.079999999999998, 7.079999999999998, 7.079999999999998, 16.08, 8.079999999999998, 6.079999999999998, 8.079999999999998, 15.079999999999998, 9.079999999999998, 4.079999999999998, 4.079999999999998, 4.079999999999998, 6.079999999999998, 7.079999999999998, -0.9200000000000017, 11.079999999999998, 3.0799999999999983, 7.079999999999998, 14.079999999999998, 13.079999999999998, 11.079999999999998, 8.079999999999998, -0.9200000000000017, 15.079999999999998, 5.079999999999998, 10.079999999999998, 0.0799999999999983, -0.9200000000000017, -2.9200000000000017, 4.079999999999998, 3.0799999999999983, -5.920000000000002, 5.079999999999998, 2.0799999999999983, 10.079999999999998, 8.079999999999998, 8.079999999999998, 4.079999999999998, 14.079999999999998, -4.920000000000002, -0.9200000000000017, 7.079999999999998, -0.9200000000000017, 11.079999999999998, 1.0799999999999983, 0.0799999999999983, 0.0799999999999983, 15.079999999999998, 3.0799999999999983, -2.9200000000000017, 2.0799999999999983, 4.079999999999998, -1.9200000000000017, 2.0799999999999983, -1.9200000000000017, -5.920000000000002, 19.08, -4.920000000000002, 0.0799999999999983, 6.079999999999998, 7.079999999999998, -2.9200000000000017, 2.0799999999999983, -4.920000000000002, -3.9200000000000017, -2.9200000000000017, 2.0799999999999983, 5.079999999999998, -2.9200000000000017, 4.079999999999998, 2.0799999999999983, 1.0799999999999983, 3.0799999999999983, 6.079999999999998, 0.0799999999999983, 7.079999999999998, -2.9200000000000017, -5.920000000000002, 5.079999999999998, 5.079999999999998, -4.920000000000002, 3.0799999999999983, 0.0799999999999983, 3.0799999999999983, 4.079999999999998, 1.0799999999999983, 0.0799999999999983, 9.079999999999998, 4.079999999999998, 0.0799999999999983, 0.0799999999999983, 3.0799999999999983, 2.0799999999999983, 7.079999999999998, -5.920000000000002, 1.0799999999999983, 5.079999999999998, 6.079999999999998, 1.0799999999999983, 7.079999999999998, -1.9200000000000017, 3.0799999999999983, 0.0799999999999983, 5.079999999999998, -8.920000000000002, -0.9200000000000017, -1.9200000000000017, 2.0799999999999983, 2.0799999999999983, -0.9200000000000017, 4.079999999999998, -1.9200000000000017, 5.079999999999998, -5.920000000000002, 4.079999999999998, -1.9200000000000017, 1.0799999999999983, 7.079999999999998, 1.0799999999999983, -5.920000000000002, -2.9200000000000017, 1.0799999999999983, 2.0799999999999983, -1.9200000000000017, 1.0799999999999983, 7.079999999999998, -0.9200000000000017, 2.0799999999999983, -1.9200000000000017, -5.920000000000002, 0.0799999999999983, -3.9200000000000017, 1.0799999999999983, 2.0799999999999983, -5.920000000000002, -2.9200000000000017, -2.9200000000000017, -0.9200000000000017, 5.079999999999998, 3.0799999999999983, -4.920000000000002, 3.0799999999999983, 0.0799999999999983, -0.9200000000000017, -9.920000000000002, 7.079999999999998, 8.079999999999998, -2.9200000000000017, -4.920000000000002, -3.9200000000000017, 5.079999999999998, 0.0799999999999983, -4.920000000000002, -1.9200000000000017, -0.9200000000000017, 0.0799999999999983, 7.079999999999998, -7.920000000000002, 2.0799999999999983, -2.9200000000000017, -2.9200000000000017, -5.920000000000002, 1.0799999999999983, 10.079999999999998, -0.9200000000000017, -2.9200000000000017, 5.079999999999998, 9.079999999999998, -0.9200000000000017, 2.0799999999999983, -1.9200000000000017, -2.9200000000000017, 4.079999999999998, 2.0799999999999983, -4.920000000000002, -4.920000000000002, 4.079999999999998, 6.079999999999998, -1.9200000000000017, 0.0799999999999983, 1.0799999999999983, -4.920000000000002, -2.9200000000000017, -7.920000000000002, -3.9200000000000017, -0.9200000000000017, 2.0799999999999983, -4.920000000000002, 0.0799999999999983, -1.9200000000000017, -2.9200000000000017, 0.0799999999999983, 0.0799999999999983, 3.0799999999999983, 1.0799999999999983, -4.920000000000002, 2.0799999999999983, -3.9200000000000017, -5.920000000000002, -7.920000000000002, -3.9200000000000017, -4.920000000000002, -4.920000000000002, -1.9200000000000017, 3.0799999999999983, 2.0799999999999983, 5.079999999999998, -0.9200000000000017, -1.9200000000000017, -1.9200000000000017, 3.0799999999999983, -0.9200000000000017, 0.0799999999999983, 1.0799999999999983, -9.920000000000002, -5.920000000000002, 0.0799999999999983, -0.9200000000000017, 3.0799999999999983, 3.0799999999999983, -6.920000000000002, -2.9200000000000017, -0.9200000000000017, -3.9200000000000017, -4.920000000000002, -0.9200000000000017, -6.920000000000002, 8.079999999999998, -5.920000000000002, -1.9200000000000017, -2.9200000000000017, -1.9200000000000017, -6.920000000000002, -7.920000000000002, -8.920000000000002, 5.079999999999998, 4.079999999999998, 2.0799999999999983, 1.0799999999999983, 4.079999999999998, 0.0799999999999983, -1.9200000000000017, 3.0799999999999983, -3.9200000000000017, 0.0799999999999983, -0.9200000000000017, 6.079999999999998, 1.0799999999999983, 7.079999999999998, -8.920000000000002, 5.079999999999998, 8.079999999999998, 2.0799999999999983, -2.9200000000000017, -3.9200000000000017, 5.079999999999998, -3.9200000000000017, 1.0799999999999983, -1.9200000000000017, 1.0799999999999983, 0.0799999999999983, 3.0799999999999983, 3.0799999999999983, -7.920000000000002, 11.079999999999998, 6.079999999999998, -6.920000000000002, -4.920000000000002, -3.9200000000000017, 3.0799999999999983, 11.079999999999998, 4.079999999999998, -6.920000000000002, 1.0799999999999983, -7.920000000000002, -1.9200000000000017, -5.920000000000002, 4.079999999999998, -1.9200000000000017, -5.920000000000002, -7.920000000000002, -0.9200000000000017, 11.079999999999998, -0.9200000000000017, -4.920000000000002, -0.9200000000000017, -2.9200000000000017, 6.079999999999998, 8.079999999999998, 5.079999999999998, -1.9200000000000017, 5.079999999999998, -0.9200000000000017, -5.920000000000002, -0.9200000000000017, -2.9200000000000017, -2.9200000000000017, -1.9200000000000017, 5.079999999999998, 1.0799999999999983, -2.9200000000000017, 8.079999999999998, 1.0799999999999983, 3.0799999999999983, 1.0799999999999983, 3.0799999999999983, 7.079999999999998, -3.9200000000000017, -0.9200000000000017, -3.9200000000000017, 1.0799999999999983, -1.9200000000000017, -1.9200000000000017, 0.0799999999999983, 1.0799999999999983, 0.0799999999999983, -3.9200000000000017, -3.9200000000000017, 3.0799999999999983, -0.9200000000000017, 7.079999999999998, -8.920000000000002, -7.920000000000002, -3.9200000000000017, 0.0799999999999983, -6.920000000000002, 2.0799999999999983, 5.079999999999998, -4.920000000000002, -1.9200000000000017, -10.920000000000002, 4.079999999999998, 9.079999999999998, 1.0799999999999983, -0.9200000000000017, -5.920000000000002, -2.9200000000000017, -5.920000000000002, 5.079999999999998, -4.920000000000002, -5.920000000000002, 3.0799999999999983, -3.9200000000000017, -5.920000000000002, -3.9200000000000017, -6.920000000000002, -9.920000000000002, 1.0799999999999983, 2.0799999999999983, -0.9200000000000017, -4.920000000000002, -7.920000000000002, -4.920000000000002, -0.9200000000000017, 1.0799999999999983, 1.0799999999999983, 5.079999999999998, 1.0799999999999983, 6.079999999999998, 5.079999999999998, 2.0799999999999983, 1.0799999999999983, 0.0799999999999983, 2.0799999999999983, -1.9200000000000017, 4.079999999999998, -3.9200000000000017, 1.0799999999999983, -2.9200000000000017, 0.0799999999999983, -7.920000000000002, -4.920000000000002, 0.0799999999999983, 0.0799999999999983, -1.9200000000000017, 1.0799999999999983, 3.0799999999999983, -0.9200000000000017, -5.920000000000002, -5.920000000000002, -4.920000000000002, -3.9200000000000017, -4.920000000000002, -2.9200000000000017, -2.9200000000000017, -2.9200000000000017, -2.9200000000000017, 1.0799999999999983, -5.920000000000002, -8.920000000000002, -1.9200000000000017, -5.920000000000002, 11.079999999999998, 0.0799999999999983, -0.9200000000000017, -2.9200000000000017, -1.9200000000000017, -2.9200000000000017, 2.0799999999999983, -4.920000000000002, -1.9200000000000017, 3.0799999999999983, -0.9200000000000017, -2.9200000000000017, 1.0799999999999983, -3.9200000000000017, 6.079999999999998, -1.9200000000000017, 1.0799999999999983, 3.0799999999999983, -4.920000000000002, -0.9200000000000017, -3.9200000000000017, -2.9200000000000017, -4.920000000000002, -9.920000000000002, -5.920000000000002, 2.0799999999999983, 2.0799999999999983, 3.0799999999999983, 2.0799999999999983, -9.920000000000002, -1.9200000000000017, -9.920000000000002, -0.9200000000000017, -1.9200000000000017, 2.0799999999999983, -6.920000000000002, 0.0799999999999983, 1.0799999999999983, 1.0799999999999983, 2.0799999999999983, -6.920000000000002, -7.920000000000002, 3.0799999999999983, -1.9200000000000017, 1.0799999999999983, -0.9200000000000017, 10.079999999999998, -4.920000000000002, 3.0799999999999983, -1.9200000000000017, -4.920000000000002, -3.9200000000000017, 2.0799999999999983, 5.079999999999998, -3.9200000000000017, 0.0799999999999983, 6.079999999999998, 1.0799999999999983, -10.920000000000002, 6.079999999999998, -3.9200000000000017, -0.9200000000000017, 2.0799999999999983, 1.0799999999999983, 1.0799999999999983, 5.079999999999998, -6.920000000000002, 1.0799999999999983, -1.9200000000000017, -18.92], [70.08, 46.08, 28.08, 50.08, 46.08, 91.08, 142.07999999999998, 203.07999999999998, 328.08, 371.08, 455.08, 481.08, 539.08, 538.08, 552.08, 571.08, 535.08, 512.08, 483.08, 480.08, 372.08, 326.08, 354.08, 282.08, 289.08, 290.08, 252.07999999999998, 250.07999999999998, 287.08, 265.08, 240.07999999999998, 248.07999999999998, 240.07999999999998, 269.08, 232.07999999999998, 217.07999999999998, 218.07999999999998, 191.07999999999998, 221.07999999999998, 229.07999999999998, 181.07999999999998, 215.07999999999998, 177.07999999999998, 168.07999999999998, 183.07999999999998, 157.07999999999998, 147.07999999999998, 153.07999999999998, 157.07999999999998, 135.07999999999998, 133.07999999999998, 123.08, 107.08, 124.08, 130.07999999999998, 100.08, 74.08, 78.08, 95.08, 77.08, 83.08, 56.08, 78.08, 72.08, 58.08, 45.08, 50.08, 45.08, 49.08, 52.08, 46.08, 50.08, 41.08, 32.08, 29.08, 48.08, 32.08, 23.08, 26.08, 21.08, 25.08, 26.08, 18.08, 23.08, 32.08, 17.08, 20.08, 11.079999999999998, 17.08, 8.079999999999998, 17.08, 10.079999999999998, 20.08, 20.08, 21.08, 5.079999999999998, 12.079999999999998, 21.08, 4.079999999999998, 7.079999999999998, 7.079999999999998, 16.08, 8.079999999999998, 6.079999999999998, 8.079999999999998, 15.079999999999998, 9.079999999999998, 4.079999999999998, 4.079999999999998, 4.079999999999998, 6.079999999999998, 7.079999999999998, -0.9200000000000017, 11.079999999999998, 3.0799999999999983, 7.079999999999998, 14.079999999999998, 13.079999999999998, 11.079999999999998, 8.079999999999998, -0.9200000000000017, 15.079999999999998, 5.079999999999998, 10.079999999999998, 0.0799999999999983, -0.9200000000000017, -2.9200000000000017, 4.079999999999998, 3.0799999999999983, -5.920000000000002, 5.079999999999998, 2.0799999999999983, 10.079999999999998, 8.079999999999998, 8.079999999999998, 4.079999999999998, 14.079999999999998, -4.920000000000002, -0.9200000000000017, 7.079999999999998, -0.9200000000000017, 11.079999999999998, 1.0799999999999983, 0.0799999999999983, 0.0799999999999983, 15.079999999999998, 3.0799999999999983, -2.9200000000000017, 2.0799999999999983, 4.079999999999998, -1.9200000000000017, 2.0799999999999983, -1.9200000000000017, -5.920000000000002, 19.08, -4.920000000000002, 0.0799999999999983, 6.079999999999998, 7.079999999999998, -2.9200000000000017, 2.0799999999999983, -4.920000000000002, -3.9200000000000017, -2.9200000000000017, 2.0799999999999983, 5.079999999999998, -2.9200000000000017, 4.079999999999998, 2.0799999999999983, 1.0799999999999983, 3.0799999999999983, 6.079999999999998, 0.0799999999999983, 7.079999999999998, -2.9200000000000017, -5.920000000000002, 5.079999999999998, 5.079999999999998, -4.920000000000002, 3.0799999999999983, 0.0799999999999983, 3.0799999999999983, 4.079999999999998, 1.0799999999999983, 0.0799999999999983, 9.079999999999998, 4.079999999999998, 0.0799999999999983, 0.0799999999999983, 3.0799999999999983, 2.0799999999999983, 7.079999999999998, -5.920000000000002, 1.0799999999999983, 5.079999999999998, 6.079999999999998, 1.0799999999999983, 7.079999999999998, -1.9200000000000017, 3.0799999999999983, 0.0799999999999983, 5.079999999999998, -8.920000000000002, -0.9200000000000017, -1.9200000000000017, 2.0799999999999983, 2.0799999999999983, -0.9200000000000017, 4.079999999999998, -1.9200000000000017, 5.079999999999998, -5.920000000000002, 4.079999999999998, -1.9200000000000017, 1.0799999999999983, 7.079999999999998, 1.0799999999999983, -5.920000000000002, -2.9200000000000017, 1.0799999999999983, 2.0799999999999983, -1.9200000000000017, 1.0799999999999983, 7.079999999999998, -0.9200000000000017, 2.0799999999999983, -1.9200000000000017, -5.920000000000002, 0.0799999999999983, -3.9200000000000017, 1.0799999999999983, 2.0799999999999983, -5.920000000000002, -2.9200000000000017, -2.9200000000000017, -0.9200000000000017, 5.079999999999998, 3.0799999999999983, -4.920000000000002, 3.0799999999999983, 0.0799999999999983, -0.9200000000000017, -9.920000000000002, 7.079999999999998, 8.079999999999998, -2.9200000000000017, -4.920000000000002, -3.9200000000000017, 5.079999999999998, 0.0799999999999983, -4.920000000000002, -1.9200000000000017, -0.9200000000000017, 0.0799999999999983, 7.079999999999998, -7.920000000000002, 2.0799999999999983, -2.9200000000000017, -2.9200000000000017, -5.920000000000002, 1.0799999999999983, 10.079999999999998, -0.9200000000000017, -2.9200000000000017, 5.079999999999998, 9.079999999999998, -0.9200000000000017, 2.0799999999999983, -1.9200000000000017, -2.9200000000000017, 4.079999999999998, 2.0799999999999983, -4.920000000000002, -4.920000000000002, 4.079999999999998, 6.079999999999998, -1.9200000000000017, 0.0799999999999983, 1.0799999999999983, -4.920000000000002, -2.9200000000000017, -7.920000000000002, -3.9200000000000017, -0.9200000000000017, 2.0799999999999983, -4.920000000000002, 0.0799999999999983, -1.9200000000000017, -2.9200000000000017, 0.0799999999999983, 0.0799999999999983, 3.0799999999999983, 1.0799999999999983, -4.920000000000002, 2.0799999999999983, -3.9200000000000017, -5.920000000000002, -7.920000000000002, -3.9200000000000017, -4.920000000000002, -4.920000000000002, -1.9200000000000017, 3.0799999999999983, 2.0799999999999983, 5.079999999999998, -0.9200000000000017, -1.9200000000000017, -1.9200000000000017, 3.0799999999999983, -0.9200000000000017, 0.0799999999999983, 1.0799999999999983, -9.920000000000002, -5.920000000000002, 0.0799999999999983, -0.9200000000000017, 3.0799999999999983, 3.0799999999999983, -6.920000000000002, -2.9200000000000017, -0.9200000000000017, -3.9200000000000017, -4.920000000000002, -0.9200000000000017, -6.920000000000002, 8.079999999999998, -5.920000000000002, -1.9200000000000017, -2.9200000000000017, -1.9200000000000017, -6.920000000000002, -7.920000000000002, -8.920000000000002, 5.079999999999998, 4.079999999999998, 2.0799999999999983, 1.0799999999999983, 4.079999999999998, 0.0799999999999983, -1.9200000000000017, 3.0799999999999983, -3.9200000000000017, 0.0799999999999983, -0.9200000000000017, 6.079999999999998, 1.0799999999999983, 7.079999999999998, -8.920000000000002, 5.079999999999998, 8.079999999999998, 2.0799999999999983, -2.9200000000000017, -3.9200000000000017, 5.079999999999998, -3.9200000000000017, 1.0799999999999983, -1.9200000000000017, 1.0799999999999983, 0.0799999999999983, 3.0799999999999983, 3.0799999999999983, -7.920000000000002, 11.079999999999998, 6.079999999999998, -6.920000000000002, -4.920000000000002, -3.9200000000000017, 3.0799999999999983, 11.079999999999998, 4.079999999999998, -6.920000000000002, 1.0799999999999983, -7.920000000000002, -1.9200000000000017, -5.920000000000002, 4.079999999999998, -1.9200000000000017, -5.920000000000002, -7.920000000000002, -0.9200000000000017, 11.079999999999998, -0.9200000000000017, -4.920000000000002, -0.9200000000000017, -2.9200000000000017, 6.079999999999998, 8.079999999999998, 5.079999999999998, -1.9200000000000017, 5.079999999999998, -0.9200000000000017, -5.920000000000002, -0.9200000000000017, -2.9200000000000017, -2.9200000000000017, -1.9200000000000017, 5.079999999999998, 1.0799999999999983, -2.9200000000000017, 8.079999999999998, 1.0799999999999983, 3.0799999999999983, 1.0799999999999983, 3.0799999999999983, 7.079999999999998, -3.9200000000000017, -0.9200000000000017, -3.9200000000000017, 1.0799999999999983, -1.9200000000000017, -1.9200000000000017, 0.0799999999999983, 1.0799999999999983, 0.0799999999999983, -3.9200000000000017, -3.9200000000000017, 3.0799999999999983, -0.9200000000000017, 7.079999999999998, -8.920000000000002, -7.920000000000002, -3.9200000000000017, 0.0799999999999983, -6.920000000000002, 2.0799999999999983, 5.079999999999998, -4.920000000000002, -1.9200000000000017, -10.920000000000002, 4.079999999999998, 9.079999999999998, 1.0799999999999983, -0.9200000000000017, -5.920000000000002, -2.9200000000000017, -5.920000000000002, 5.079999999999998, -4.920000000000002, -5.920000000000002, 3.0799999999999983, -3.9200000000000017, -5.920000000000002, -3.9200000000000017, -6.920000000000002, -9.920000000000002, 1.0799999999999983, 2.0799999999999983, -0.9200000000000017, -4.920000000000002, -7.920000000000002, -4.920000000000002, -0.9200000000000017, 1.0799999999999983, 1.0799999999999983, 5.079999999999998, 1.0799999999999983, 6.079999999999998, 5.079999999999998, 2.0799999999999983, 1.0799999999999983, 0.0799999999999983, 2.0799999999999983, -1.9200000000000017, 4.079999999999998, -3.9200000000000017, 1.0799999999999983, -2.9200000000000017, 0.0799999999999983, -7.920000000000002, -4.920000000000002, 0.0799999999999983, 0.0799999999999983, -1.9200000000000017, 1.0799999999999983, 3.0799999999999983, -0.9200000000000017, -5.920000000000002, -5.920000000000002, -4.920000000000002, -3.9200000000000017, -4.920000000000002, -2.9200000000000017, -2.9200000000000017, -2.9200000000000017, -2.9200000000000017, 1.0799999999999983, -5.920000000000002, -8.920000000000002, -1.9200000000000017, -5.920000000000002, 11.079999999999998, 0.0799999999999983, -0.9200000000000017, -2.9200000000000017, -1.9200000000000017, -2.9200000000000017, 2.0799999999999983, -4.920000000000002, -1.9200000000000017, 3.0799999999999983, -0.9200000000000017, -2.9200000000000017, 1.0799999999999983, -3.9200000000000017, 6.079999999999998, -1.9200000000000017, 1.0799999999999983, 3.0799999999999983, -4.920000000000002, -0.9200000000000017, -3.9200000000000017, -2.9200000000000017, -4.920000000000002, -9.920000000000002, -5.920000000000002, 2.0799999999999983, 2.0799999999999983, 3.0799999999999983, 2.0799999999999983, -9.920000000000002, -1.9200000000000017, -9.920000000000002, -0.9200000000000017, -1.9200000000000017, 2.0799999999999983, -6.920000000000002, 0.0799999999999983, 1.0799999999999983, 1.0799999999999983, 2.0799999999999983, -6.920000000000002, -7.920000000000002, 3.0799999999999983, -1.9200000000000017, 1.0799999999999983, -0.9200000000000017, 10.079999999999998, -4.920000000000002, 3.0799999999999983, -1.9200000000000017, -4.920000000000002, -3.9200000000000017, 2.0799999999999983, 5.079999999999998, -3.9200000000000017, 0.0799999999999983, 6.079999999999998, 1.0799999999999983, -10.920000000000002, 6.079999999999998, -3.9200000000000017, -0.9200000000000017, 2.0799999999999983, 1.0799999999999983, 1.0799999999999983, 5.079999999999998, -6.920000000000002, 1.0799999999999983, -1.9200000000000017, -18.92]]
  in  "?":T1(tab)=enum."Raw Counts WV offline"
  out "NRB WV Offline":dbl[][](graph)=[[9.748472800266532e-06, 5.0372226189685124e-05, 0.000162213658027644, 0.00041985973250955786, 0.00097235721004923, 0.0020663692899652686, 0.0039991701845159015, 0.007118970291173257, 0.011413712157636093, 0.016761938699585737, 0.0230665756726796, 0.029878933075533045, 0.036990509612321254, 0.04453154822122842, 0.05242772133561194, 0.06019117437993257, 0.06744770267689784, 0.07276552005008248, 0.07535935355283363, 0.07605240361408463, 0.0759353796130153, 0.07471657915495665, 0.07335374037200824, 0.07317369073855624, 0.0731757502428157, 0.07518525639035022, 0.07904902658339757, 0.08273246616274091, 0.08638094095490742, 0.09062262702857289, 0.09505525269332155, 0.09818753152237104, 0.10099769100794488, 0.10468329665790409, 0.10801375071302727, 0.11105164191489127, 0.11347115936903837, 0.11556294945398175, 0.11797676358119881, 0.11926310547926207, 0.11986753704005482, 0.1219901747922792, 0.1234448273935287, 0.12412304257965061, 0.12560043000434015, 0.12703408169589148, 0.13025640560830024, 0.1296860630926595, 0.129349131296115, 0.1316453203933485, 0.13153215096874696, 0.13114775871807402, 0.13172337235506895, 0.13045895604723456, 0.1301834688356291, 0.13132484659257573, 0.12886828674000286, 0.12605778630708728, 0.1260438382374272, 0.1281232178323105, 0.12655214582716462, 0.12385574007297452, 0.12117459587987349, 0.11717694477798667, 0.114218332332916, 0.11099050914498809, 0.10910378733993187, 0.10831552582575234, 0.10660143067413612, 0.10241438367180009, 0.09925430543004427, 0.09715011398665005, 0.09514422305653167, 0.09322280424225186, 0.08944537027147066, 0.08590613256337537, 0.08261821446827151, 0.08220558040753174, 0.08253512853431853, 0.081004795716341, 0.07805112992468188, 0.0748749703034283, 0.07186727370506621, 0.07215479691729551, 0.07297799487388945, 0.06965827982465335, 0.06626109791761776, 0.0691570762709819, 0.07058274042480488, 0.06712632642257751, 0.06871274070671493, 0.06663135367863768, 0.06663213869580317, 0.0670698941239992, 0.06366541771127536, 0.06354600421305173, 0.06348974794659003, 0.06310163873444442, 0.06337313737412924, 0.062037777537366876, 0.06356419136068275, 0.06382478038488479, 0.05932521540718684, 0.05627826387200987, 0.05332457615047566, 0.05553229602731323, 0.0583323481464287, 0.05775412770205614, 0.05642643685199394, 0.05525686662474926, 0.053887528866082425, 0.05193402457019617, 0.05189953915486178, 0.05177118534183911, 0.05154492591190042, 0.05504287888892559, 0.05646022821425235, 0.0490750663985394, 0.04682579602965382, 0.05002021513993977, 0.04705715240227577, 0.04564447259794862, 0.047836302578748685, 0.04921894106606058, 0.051707525119877064, 0.05117147541386723, 0.04836856602745608, 0.04791521241764385, 0.04669169312328514, 0.04318629873950716, 0.04226410740200536, 0.04811597627603741, 0.04379517584139457, 0.03890590645577133, 0.040891174567268394, 0.039352249497504654, 0.03897840020564977, 0.039524666919816286, 0.041863500703495087, 0.04218682659121029, 0.041598892131525914, 0.03827257870901242, 0.037133323081506596, 0.040196645183117705, 0.03946807364535187, 0.038290698899193544, 0.04059253970744207, 0.03717582402988755, 0.03504503243887363, 0.036279969763350475, 0.03786558697329307, 0.03972473366481077, 0.03518116861915791, 0.03391046804993847, 0.0378929450599597, 0.03882780868536266, 0.03000461012404495, 0.02449520904567828, 0.029389157689312925, 0.03099530463875866, 0.03182342742056474, 0.03057709818142377, 0.03078250613511755, 0.030845672220814774, 0.02696228995931792, 0.03002134001274165, 0.031402543803566704, 0.028724629173382973, 0.028955862617072562, 0.027829635072127466, 0.026480077875895947, 0.02883554088733459, 0.03467535948353092, 0.02643024306237674, 0.019386083541421684, 0.02611218976005994, 0.02342716537295639, 0.025138841136918055, 0.028305336743879344, 0.025284390525779278, 0.019157393189434564, 0.02524461019397857, 0.03670352061357465, 0.02933473354672988, 0.02336102810701446, 0.022531434654566553, 0.018943615608582424, 0.02011471672631707, 0.031137015808314343, 0.03076118390354845, 0.024139692621457647, 0.02876801766488665, 0.027028192782106407, 0.028928728908742027, 0.03126092313096124, 0.02572069117183131, 0.023250766050392273, 0.02134007898366918, 0.017992705358663083, 0.012957531153950595, 0.015827178373507365, 0.018060368685652486, 0.02049676988282659, 0.027863189395224194, 0.022053558088049794, 0.017122467003644202, 0.024050623767124184, 0.03190052840146169, 0.0285621799387345, 0.026133083780907996, 0.0355562700258741, 0.040934862619831584, 0.02599757169418167, 0.007369729072920344, 0.005389180728984952, 0.013105795540254494, 0.027474455348150392, 0.02791419178848161, 0.021040507313989598, 0.018960803774108484, 0.025311932831042848, 0.03171169266410968, 0.020519080396121145, 0.017562628912759885, 0.0199644939596786, 0.030400189615917044, 0.038733902333224136, 0.033449002342567105, 0.017192813873118808, 0.01803317211882512, 0.02570593072652359, 0.016382767836578962, 0.018011078426507874, 0.016809262465707787, 0.012488042811980272, 0.009689219637239717, 0.020099805984051894, 0.01997430182546375, 0.004201290612045081, 0.00078120129582252, 0.006089733807262544, 0.013243091701961305, 0.013737795050055337, 0.015326278741908395, 0.021401377635119977, 0.012106116168599837, 0.016182844587705008, 0.02650057523747294, 0.01563741720313049, 0.015681764566359703, 0.021476519407525554, 0.02131672276965664, 0.010718029714751016, 0.00264182792514413, 0.010718556354803522, 0.014990603273134308, 0.021223529007125257, 0.022083468554994008, 0.011057462188951556, 0.017225869168403254, 0.018780023230657462, 0.018745168890085692, 0.01906894242364831, 0.024667703442812286, 0.023755958744844145, 0.012309150112261805, 0.01770106029198504, 0.025046206272770908, 0.024006698337057895, 0.01829121019020196, 0.00731711795518149, 0.0009069279347923446, 0.017339228899483035, 0.025886509440764673, 0.026371677285841763, 0.025073690059648858, 0.011046818891248514, 0.009614935284226241, 0.013541700405457794, 0.023045190924709608, 0.021974409435864078, 0.006471287780504446, 0.02333277247614725, 0.028336438419634614, 0.015401508878097863, 0.025750158498142994, 0.021956075126148302, 0.004478090960507314, -0.010848270783005341, -0.00916870510774881, 0.008105692215866368, 0.0011563949181772881, -0.004993170685271582, -0.0013075534607345678, -0.0013164635096536848, 0.007015517067404128, 0.010744053048286012, 0.03861091282234107, 0.036422104360270734, 0.009553777102586609, -0.00680552437150194, -0.021717954324143224, 0.001963524509800547, 0.02559834111471714, 0.033167232894744464, 0.017876936132595368, 0.004473893631059187, 0.018235097523713967, 0.02408148629815813, 0.005814990866969563, 0.003456039730618414, 0.007413612507405712, 0.013849259404667105, 0.006480336547268271, -0.0039595793931106555, 0.012813793099451305, 0.02731029063179255, 0.025768473280852237, 0.0008493142537772154, 0.007130976195850999, 0.005697489461299915, 0.0111415896791271, 0.02250349596491675, -0.005968742418450371, -0.0036639955667015574, 0.00532198901782691, 0.02808438707007371, 0.02390709428856152, -0.017587939328537826, 0.0031811431250178533, 0.014202043236324029, 0.006957115726611781, 0.02174931191882205, 0.0034042082277176387, -0.013552087535458198, -0.018344324224966575, -0.001421797901953285, 0.026429967974688624, -0.002787526731116808, -0.013808894769244861, -0.0032754363512004373, 0.005094553812464665, 0.017551851934552432, -0.005802446529902196, -0.007543635793354201, 0.003497095779197744, 0.0005338815277823271, -0.011781570354678925, 0.005940595620726085, 0.02738144968528805, 0.0170948157280786, 0.02914952792061579, 0.04036562498906577, 0.0026801406993885767, -0.008480327336336538, 0.011800658677393985, -0.0069141073825147205, 0.006418075581323811, 0.0353626453255764, 0.02119392455338507, 0.02726014334962578, 0.03715240203822589, 0.016221597767418012, -0.0009676040738129287, -0.002362824209170887, 0.003563687547521733, -0.007833814796078515, -0.016000349245178243, 0.02670605795145352, 0.043275954257899006, 0.01586749531826351, 0.002598696513423454, -0.0068220033063375665, 0.01703720894899675, 0.017861993255752016, -0.0001106200648171446, -0.003818181694018804, -0.010173781497964754, -0.0017982765757774916, 0.002523359733844531, 0.014841375717479207, 0.024053742676176063, 0.00677186536028385, -0.002615219415181097, 0.014188144078326805, 0.028640544259606236, 0.014531249230272996, 0.012643207205608986, 0.032047534584016275, 0.026063546754845356, 0.002870933935055271, 0.007895432414462644, 0.023041980632556927, 0.028018028547576075, 0.017783363411377685, 0.008466390722209139, -0.0173882987487479, -0.05156012755205645, -0.00697576024151881, 0.04452711477486673, 0.034055257423916054, 0.02453091786336174, 0.011733502220623736, 0.013920294725557588, 0.01719785450898298, -0.0016337008066818904, -0.001641758504974932, 0.02201236824432719, 0.05004381677091647, 0.014775275641376505, 0.014406860266983098, 0.04945246077727454, 0.026781528614159122, -0.016003671008945928, -0.03135353468814051, 0.006183645864102918, 0.046804957571617345, 0.04657399349683907, 0.03580750840753616, 0.029997502117489704, 0.006102046168893726, -0.004319610083311249, 0.004060104574077678, 0.005017100292681805, 0.037782578345210344, 0.01689761657412853, -0.01892668738759807, 0.0027233253992371737, -0.00014400341889012812, 0.018904322580871644, 0.00833336631525141, -0.0025797651895792645, 0.017946506629120673, -0.004077502885129058, 0.015398237390799681, 0.020675082408243638, 0.0020919401846347377, 0.006604797677880668, 0.03277295127882503, 0.03595211477706779, -0.03464438211342852, -0.05238073192311515, 0.004964967943170736, 0.0278678725106764, 0.01998798953230833, -0.008456561449478909, 0.00870300009160727, 0.03884177942378451, -0.01672075283552095, -0.05508624895335171, -0.02880635231545434, 0.005968046510685425, 0.019642670657239764, 0.06381208503756766, 0.013876938243529195, -0.059547800684956465, -0.031212049526229073, -0.007823544195646693, 0.013572505722628291, 0.029084715646215443, 0.003990906331145688, 0.010131945720249514, -0.00296329348810934, -0.027402570370228786, 0.004342440069432064, 0.013706447078023905, -0.008702854222868333, -0.03301830652102339, -0.03660171505376773, -0.03963867022817906, 0.0061910296481667605, 0.0262639928898694, -0.019431328572938753, -0.05086403326518871, -0.036661512837107425, 0.00484579430483467, 0.022669306398666794, 0.011739769756000634, 0.02196216539366083, 0.010335902579303058, 0.05050740762742822, 0.06798721484383423, 0.009248584639812932, 0.003177102270038192, 0.017607723197185652, 0.01090393629132112, -0.028949385778199433, -0.020993860637128294, 0.006985106751123873, 0.022043108867765174, 0.030307382629946224, 0.02474881525806438, 0.010586387346240927, 0.01285709468635182, 0.001405950780664786, 0.028040326441361917, 0.020100426580335815, -0.02024599210711805, 0.017989482026473484, -0.004433897934266949, -0.021145306490160394, 0.04581200111698051, 0.054573388133573784, 0.009739032580745858, 0.0027936316658016664, 0.05188733210953194, 0.037343046621283814, 0.025375047934424612, 0.0568967079202993, 0.03371593400724599, 0.07266852960704986, 0.10987466426863662, 0.057794472488052966, 0.03459142269009697, 0.05409542220304495, 0.015069427617235008, -0.01868323405453398, 0.023584539328951236, 0.045805879636446376, 0.06079298876091565, 0.049345468306829676, -0.03894546595711354, -0.04658558846697308, -0.006302051629734852, 0.007692007098669576, 0.043080880568933805, 0.060991990126627586, 0.0423184290340551, 0.014743489624987206, 0.02029407713718578, -0.008310059279973242, 0.0112202950807729, 0.05016283549672845, 0.03510450813898451, 0.05165979683211343, 0.020381505809218502, -0.007746802108806152, 0.011852272955009888, -0.030157573104291565, -0.06829645362083113, -0.005954233658534257, 0.035398014148402275, 0.0562924168242942, 0.05765773801544471, -0.00023240808024213095, -0.025891994103805105, 0.0060090052063114605, -0.02960661547686603, -0.034431382977071524, 0.030138862235568695, 0.019162680466278333, 0.006516722458955687, -0.007417710967674415, 0.037383053717509, 0.0628249313755978, 0.019915180434260406, -0.04434312424850089, -0.11758979067019729, 0.0, 0.0]] caption="Water Vapor Number Density"
  out "NRB HSRL Combined":dbl[][](graph)=[[2.2695626807423936e-05, 5.7825220079270064e-05, 0.00015742286300517112, 0.0003542975828255901, 0.000787270089794345, 0.0016891836112965734, 0.003512942899764533, 0.006634370426473158, 0.010691718725240969, 0.01641864087933985, 0.02288715998769279, 0.029306160747604223, 0.03618401554830513, 0.04280809034115865, 0.049688752204761856, 0.05564745303160648, 0.05994336531955179, 0.06345015108229356, 0.06880014197975923, 0.06831276544962156, 0.062408931809091274, 0.0645581523002176, 0.06749774663492815, 0.06767261425724833, 0.07021014995851434, 0.07379697578736114, 0.07759052058673033, 0.08540069780735585, 0.09154305295739187, 0.09072999692552892, 0.09520538831179273, 0.1013656610331658, 0.10654976621096018, 0.11182385097761598, 0.1131165329759155, 0.11915977926971602, 0.12105031551464815, 0.12236890579968368, 0.1270288883228458, 0.1283739421123255, 0.13274544080657835, 0.13058061282624647, 0.12269322623506652, 0.12915487746624588, 0.1376534068193933, 0.12820258580391822, 0.12327800278556038, 0.13222013776268257, 0.1350362182134283, 0.12964395195602393, 0.1257405333817877, 0.12837108710285464, 0.1347977143498602, 0.14384710863009556, 0.1372807166618981, 0.11818130233159549, 0.11795246438646964, 0.12186196955566032, 0.11662334493842298, 0.11705945410110956, 0.11365438076835246, 0.11362049990668613, 0.11418412691962952, 0.10911395522018633, 0.10605205539888528, 0.10401517142140292, 0.10188066873852607, 0.09564626200142483, 0.09754151805368302, 0.10058248637126148, 0.09930314624039749, 0.09578457808853226, 0.08480933424052038, 0.07808357516197806, 0.08663774502206754, 0.08418258659642527, 0.07145749334654686, 0.06877014355133508, 0.06956101889032913, 0.06780237035863111, 0.06847385580175683, 0.06116654476402323, 0.06212461587547134, 0.07558626305787428, 0.0708484643167193, 0.07077669377961161, 0.07780080206708481, 0.07014009337275298, 0.06269232459309353, 0.06538563673643384, 0.05738494090087131, 0.049316232061406146, 0.056868288743986604, 0.06331969189182361, 0.06040723355940888, 0.05224553138283072, 0.05482235674217514, 0.054066747330198776, 0.05440354599136194, 0.049598911730383534, 0.06064265809513942, 0.06717796214159229, 0.04927603462951031, 0.04086389679124908, 0.049470990510644984, 0.05130303224260035, 0.03919648766728223, 0.049581399212128695, 0.0416114863928341, 0.022837286828631048, 0.03441655232170179, 0.04245117768151879, 0.046733538752661834, 0.04449275515101755, 0.033295226586791904, 0.05825898705557959, 0.07922085545187625, 0.06577038232944504, 0.06856343329673217, 0.047597757977041744, 0.04551076083527019, 0.05212906013558983, 0.035705059003115075, 0.018724814824564274, 0.018412630634695896, 0.034966662381579264, 0.027900391666778344, 0.023824237393078, 0.0314078752161363, 0.051867041579319775, 0.04320449024241481, 0.048670887724481145, 0.06683075724301081, 0.04449870664398313, 0.03870458789403695, 0.07425126588903734, 0.05464584185513839, 0.007440379200439226, 0.01059243630105301, 0.029272662551022042, 0.05553408625174526, 0.06029590482388896, 0.043427715656798996, 0.02770236542948132, 0.047963557215643146, 0.0578632414001878, 0.022059826500649637, 0.016322017466696988, 0.04015280067782085, 0.047783441844490064, 0.04303413032889391, 0.03996594017417364, 0.017443485522183607, 0.04756346808605609, 0.057646304120309876, 0.02484371964088155, 0.010601019131733226, 0.030401032601484287, 0.04771483043922493, 0.02815066801250639, 0.007064504749934788, 0.011286995257138494, 0.004101888025226123, -0.0022032859026500547, 0.04816689073466177, 0.056350138384117766, 0.038356913529105405, 0.05660445788753782, 0.030281775858684964, -0.008058397290816501, 0.02409262253491745, 0.044183798413746735, 0.02583826699439479, 0.014213494870408875, 0.0035219324630137924, 0.0548032179025485, 0.07640576142115349, 0.0298492006624736, 0.05542541071332661, 0.05859874518991917, 0.026992866415869177, 0.025987340421971553, 0.05661114896579767, 0.03856272457002181, 0.056507274068756934, 0.08028527588214339, 0.023303006006329362, 0.0026726282337830192, 0.011142255551226802, 0.0027297951346640726, 0.022873768594151526, -0.00447169885568289, -0.010386409712305329, 0.07696305008799015, 0.05828815793782281, -0.003146989561131933, 0.01821943197336828, 0.007596585989011763, -0.007922975986752023, 0.04240996583969043, 0.05079139295392891, -0.0017355885208677874, -0.04070324949782166, -0.011604092098775765, 0.041246560182902306, 0.07173551666256352, 0.050493619844229405, 0.05439070381324177, 0.0721196271321365, 0.045020054082958436, -0.008907320873366499, -0.01607215991125327, 0.01593855099450408, 0.02691062876160374, 0.05629257058178222, 0.08254451622098732, 0.036943541635376706, -0.02260972321680323, -0.005817793750472192, 0.02653454360390071, 0.01908189248732684, 0.009549794507765936, 0.06839438319369222, 0.08086690804949875, 0.057662982377048484, 0.042083197858946125, -0.012338811176529182, -0.014495076981515746, -0.024949004612666827, 0.0019167464789003363, 0.04396588458280258, 0.023148576159130553, -0.006585396570534078, -0.026050374641429123, -0.013223832157112, 0.02614727210669483, 0.06176542467165903, 0.042208927930222066, 0.056062933116182344, 0.05653306047674415, 0.027266943967770442, -0.014023368156615788, 0.006790745796195966, 0.09360712606321431, 0.06364145498818546, 0.02602666533230426, 0.04305868249759223, 0.12092641147685072, 0.15120921873896193, -0.00019692040896413662, -0.07463327489665034, -0.0027011276695713153, 0.04013396162229779, 0.11414270422910705, 0.040770998679715564, 0.010117856660815957, 0.10384737082352256, 0.039114313321848886, -0.005495189680088796, 0.03439820534707865, 0.09905583956627603, 0.11874229559019975, 0.07061206623274723, 0.021739890901662975, 0.0772219008272758, 0.08337946196406672, 0.03346762570407511, -0.02568455886137983, -0.05437447847890524, -0.0002296879650157666, 0.008445852800528848, -0.026456983777014987, -0.050133293290274196, -0.00910691360919185, 0.03550322200999707, 0.014760675806013677, -0.009307426798439995, 0.01193158621482087, 0.015083303998843608, -0.03421145913542102, -0.0842112034454656, -0.05036139892242393, 0.0249817223717758, 0.07916198829535202, -0.016250693783589624, -0.04857886705351524, 0.006228545580253325, -0.01659461428360798, 0.029341702872269056, 0.082542194203024, 0.1298066930265029, 0.056819111330711956, -0.06789076045865451, -0.04112225477585228, 0.027145230798284268, -0.00027605405682882487, -0.06628319636469578, -0.06323296967110408, -0.03901197268068591, 0.003261005351626281, 0.021124095529170838, 0.046409081663830794, 0.1335009406018737, 0.09434406617076388, -0.033266123970815575, -0.00767054129909802, 0.06280662910264909, 0.11178853072190664, 0.06738818966959964, -0.0040875908453924725, 0.07969161602543522, 0.04186561752442042, -0.08133370491689472, -0.046907420888055114, 0.03485866389891042, 0.03508034005834819, 0.05113374640713886, -0.0003186140709774208, 0.019718298817157087, 0.14083502260319097, -0.004382824644121588, -0.08199496333556747, 0.06130576880228309, -0.0003307506696227073, -0.025292300074150387, 0.012221939410261349, 0.012297035635513527, 0.06745570352877385, 0.038026068421083026, -0.1633158904927156, -0.20745292864672107, -0.04809851877222762, 0.0869976510099023, 0.10948961969693873, -0.00035359028633600014, 0.05744703832638745, 0.1383037522639789, 0.10312859223945016, -0.004888137643531199, 0.10435265977102022, 0.1416064121107673, 0.013451079464618619, 0.02279692748243152, 0.06487586264279327, -0.005062700316054524, -0.009806981525938945, 0.08972415089241771, 0.12840041257624676, 0.19150499801171667, 0.14917987877270572, 0.1160665121454807, 0.05816847894117919, 0.12720870565132353, 0.127930455724717, 0.02938338582425972, -0.010382050942826342, 0.004617909678437976, 0.0399774933643356, 0.06558099265291191, 0.17824432548216354, 0.05091565100716451, 0.12861663849157048, 0.30059976079657946, 0.19266456040242083, 0.12551002898175878, 0.09454291780962588, 0.10566987362923938, 0.20225617618926578, 0.18726794445969808, 0.08044512790338788, -0.011275374588290303, -0.1366856385378571, -0.06619114934413384, 0.005068182050711975, 0.08817257499938486, 0.14989378326380184, -0.07321588540862344, -0.2086543287157022, -0.06268071685804862, 0.13035055424684536, 0.09101666957856502, -0.057929993842317534, -0.06401077460606856, -0.06434547089633473, 0.02872165998931917, 0.2401316532155436, 0.29446910315550945, 0.17147290901669907, 0.11871846214204677, 0.08937694634116361, -0.07875463682398216, -0.06100267655619283, 0.005596211283925861, 0.011738572784618059, 0.06095805317940195, 0.16626403007792231, 0.18572776330904223, 0.03693271849320402, 0.20014456448252368, 0.18854533769928597, -0.057503101323634676, -0.03869668034256092, 0.15940065657929758, 0.2630495309352477, 0.1351455973219054, 0.12932161712945606, 0.19520216652843134, 0.15682418062990805, 0.039002437326466896, 0.019331815413309993, 0.01942623195378785, -0.04733095466201925, 0.0733581578271169, 0.10071565480006625, -0.06837116025803253, 0.04716465159541355, 0.07478602035774103, 0.13019759769225553, -0.042038736031412234, -0.27149154538968495, 0.006422042772528818, 0.11867346854731783, -0.06398574894892836, -0.10676945576082887, 0.042113660499955664, -0.007719038878859979, -0.15136924010444625, -0.30357436336047927, 0.006668429843540581, 0.4509376388257295, 0.3067011756986518, 0.1758167284570595, -0.0448949401051113, -0.18604434134319436, -0.0825722366696434, -0.0005989405129991361, -0.03820718671786184, -0.24993069436785284, -0.09927768894339166, 0.007014784845276089, -0.21507127333461495, -0.23143529653353428, -0.14746807018983532, -0.30340565358243154, -0.1410038829232961, 0.10905258833705608, 0.04658651012227343, -0.0006323634201718005, -0.1911873214082381, -0.28773724447124255, -0.17687358435342376, -0.0006437060357281345, 0.15291384597897287, 0.3240715935844779, 0.2439599908574667, 0.023913030159322, 0.14740059304265993, 0.1810931951556093, 0.12380029212427801, 0.12434031456798303, 0.2420660677086958, 0.25993102077356245, 0.15129647606625826, 0.12651215673548424, 0.05892992321108944, -0.04344642239789708, -0.07798952658609189, 0.007935982623717718, -0.08732175225151453, 0.051503986737385224, 0.3750089252507248, 0.13968667696826992, -0.10643992015765022, 0.1231751057592974, 0.2481052527469435, 0.026056665134361258, -0.2068154296884945, -0.17169052861035897, -0.09108519309486565, -0.009800009685519518, -0.08273564856771688, -0.000731989393474925, 0.3667950959446587, 0.26682270814257514, 0.17528061352281768, -0.1123711426840345, -0.30897923757078294, 0.008628765093974323, -0.10434538673368633, -0.04803683074718216, 0.25560592436496027, 0.2852502414052497, 0.20025607244927168, -0.07765731720559793, -0.16482054218424283, 0.1736321662923118, 0.1840615966230531, -0.06915275992081855, 0.018828856463337634, -0.010633691065016833, 0.12772165592192442, 0.3366660348037716, 0.1885325656150264, 0.3093393966230825, 0.2804345355425564, 0.19078816947147695, 0.3332815874968885, 0.07033271686228043, -0.09264843498503487, -0.021307059164161174, -0.06252639704295594, -0.14536404553755367, -0.39467107057004114, -0.24014437395664504, -0.0008356514474802043, 0.08305177329994802, 0.4413081892933228, 0.358468822410308, -0.20240687521671055, -0.0008519564573424408, 0.09535974388898107, -0.03305301624869506, 0.34387561999196115, 0.5290440071679154, 0.18367385485700277, -0.3277604476961577, -0.1649440090946469, 0.16381895206295172, 0.3077230893471797, 0.16506235520863155, -0.22297926253867476, -0.13464974126152085, -0.07921460304327922, -0.3153463012788162, -0.2038067738402748, 0.08961466506663462, -0.0009085718626012407, 0.13588356484577313, 0.19360040630171899, -0.23060193770158832, -0.24298329153897322, -0.09348179830674685, 0.4519712052546777, 0.24383141282765058, -0.059425821127370985, 0.19866164141333423, -0.07164671065454638, -0.3794039084431849, -0.15526276184342755, -0.03669403493500633, -0.12052578095804288, 0.047042105041156995, 0.09538932358738884, 0.1078224408082438, 0.25379193790629423, 0.16947898081684817, 0.06011716168005588, -0.07455727072461783, 0.0, 0.0]] caption="Water Vapor Number Density"
  out "CH 1 (WV off) counts display":dbl[][](graph)=[[15.08, 29.08, 26.08, 43.08, 60.08, 105.08, 122.08, 179.08, 259.08, 310.08, 381.08, 419.08, 425.08, 421.08, 491.08, 482.08, 490.08, 476.08, 466.08, 430.08, 412.08, 353.08, 298.08, 309.08, 286.08, 233.08, 228.08, 234.08, 227.08, 238.08, 217.08, 205.08, 199.08, 219.08, 217.08, 173.08, 208.08, 160.08, 176.08, 145.08, 159.08, 169.08, 167.08, 136.08, 132.08, 146.08, 137.08, 149.08, 137.08, 124.08, 101.08, 121.08, 84.08, 96.08, 96.08, 98.08, 95.08, 85.08, 87.08, 87.08, 78.08, 75.08, 79.08, 74.08, 58.08, 51.08, 71.08, 59.08, 56.08, 52.08, 50.08, 56.08, 39.08, 48.08, 37.08, 47.08, 26.08, 34.08, 29.08, 39.08, 37.08, 35.08, 35.08, 28.08, 25.08, 25.08, 32.08, 22.08, 12.08, 18.08, 26.08, 7.08, 21.08, 17.08, 21.08, 24.08, 12.08, 14.08, 22.08, 9.08, 13.08, 19.08, 8.08, 10.08, 9.08, 6.08, 6.08, 6.08, 12.08, 18.08, 10.08, 5.08, 11.08, 5.08, 6.08, 4.08, 8.08, 9.08, 7.08, 3.08, 4.08, 13.08, 2.08, 9.08, -3.92, 14.08, 11.08, -1.92, 1.08, 14.08, 2.08, 6.08, 8.08, -1.92, 5.08, 4.08, 9.08, 5.08, 8.08, 8.08, 17.08, 5.08, 7.08, 5.08, 3.08, 9.08, -1.92, 1.08, -8.92, 1.08, -2.92, 4.08, -5.92, -1.92, -2.92, 6.08, 1.08, 8.08, 0.08000000000000007, 4.08, 11.08, -1.92, 4.08, 0.08000000000000007, 7.08, 6.08, 4.08, 0.08000000000000007, -1.92, 3.08, 4.08, -1.92, 1.08, 2.08, 5.08, -7.92, 0.08000000000000007, -3.92, 1.08, 1.08, 0.08000000000000007, 8.08, -1.92, -0.9199999999999999, -1.92, 1.08, -5.92, 3.08, 7.08, 9.08, 2.08, 3.08, 3.08, 5.08, 4.08, 0.08000000000000007, 0.08000000000000007, 1.08, -1.92, -1.92, 2.08, -2.92, 0.08000000000000007, -5.92, -3.92, -0.9199999999999999, -1.92, 2.08, -3.92, -0.9199999999999999, -0.9199999999999999, -3.92, 1.08, -4.92, 0.08000000000000007, 2.08, 0.08000000000000007, 0.08000000000000007, 1.08, 3.08, -1.92, -1.92, -4.92, -2.92, -3.92, 3.08, 6.08, -5.92, -2.92, 4.08, -2.92, 5.08, 4.08, -1.92, -3.92, 9.08, -8.92, -3.92, 7.08, -2.92, 2.08, 4.08, 4.08, 0.08000000000000007, -5.92, 1.08, -4.92, -5.92, -3.92, 0.08000000000000007, 1.08, -0.9199999999999999, -0.9199999999999999, -1.92, 4.08, -4.92, -4.92, -2.92, -1.92, -0.9199999999999999, -3.92, 0.08000000000000007, 6.08, 8.08, -1.92, 5.08, -0.9199999999999999, 11.08, 6.08, 8.08, -4.92, 1.08, -0.9199999999999999, -1.92, 0.08000000000000007, -5.92, -3.92, 3.08, 0.08000000000000007, -1.92, 0.08000000000000007, -1.92, -2.92, 2.08, -5.92, 2.08, 6.08, -2.92, -4.92, -3.92, 1.08, -3.92, -1.92, -8.92, -2.92, 2.08, -2.92, -3.92, -4.92, 3.08, -4.92, 2.08, 4.08, -0.9199999999999999, -4.92, 9.08, 8.08, 2.08, -0.9199999999999999, 5.08, 3.08, 3.08, -3.92, -1.92, 5.08, 6.08, 5.08, -0.9199999999999999, -1.92, 2.08, 4.08, -4.92, -1.92, -0.9199999999999999, -2.92, 0.08000000000000007, 3.08, 0.08000000000000007, -1.92, 5.08, -1.92, 2.08, -1.92, 0.08000000000000007, 4.08, 2.08, 0.08000000000000007, 1.08, -1.92, -0.9199999999999999, -8.92, -0.9199999999999999, -1.92, -1.92, 1.08, 2.08, -3.92, 3.08, -1.92, -0.9199999999999999, -0.9199999999999999, -3.92, 1.08, -3.92, 6.08, -0.9199999999999999, 0.08000000000000007, -1.92, -1.92, -3.92, -0.9199999999999999, 0.08000000000000007, 2.08, -0.9199999999999999, -2.92, 3.08, -2.92, -5.92, -2.92, 3.08, -2.92, 3.08, -2.92, 5.08, -0.9199999999999999, 1.08, 1.08, 0.08000000000000007, -4.92, 6.08, -2.92, -2.92, -1.92, 2.08, -4.92, -2.92, -0.9199999999999999, 5.08, 2.08, -3.92, -1.92, 0.08000000000000007, -2.92, 3.08, -1.92, -1.92, 2.08, 5.08, 3.08, -0.9199999999999999, 6.08, 4.08, -8.92, -0.9199999999999999, 3.08, 10.08, 6.08, -0.9199999999999999, 0.08000000000000007, -2.92, 3.08, -2.92, 0.08000000000000007, -0.9199999999999999, -2.92, -0.9199999999999999, 1.08, -3.92, 4.08, 2.08, -5.92, 0.08000000000000007, -2.92, 7.08, 2.08, 2.08, -1.92, 2.08, 4.08, -2.92, -0.9199999999999999, 2.08, -2.92, -2.92, 1.08, -2.92, -4.92, 7.08, 2.08, 1.08, -2.92, 8.08, 0.08000000000000007, -0.9199999999999999, 0.08000000000000007, 2.08, -0.9199999999999999, -1.92, -2.92, 0.08000000000000007, 7.08, 6.08, 1.08, -3.92, 0.08000000000000007, 1.08, -2.92, -3.92, -2.92, 5.08, 3.08, -5.92, -0.9199999999999999, 0.08000000000000007, -3.92, -0.9199999999999999, 1.08, 0.08000000000000007, -3.92, -1.92, 3.08, -0.9199999999999999, -2.92, 1.08, 0.08000000000000007, 4.08, 0.08000000000000007, 2.08, -1.92, 7.08, 0.08000000000000007, -3.92, -4.92, 3.08, -1.92, 2.08, -1.92, 0.08000000000000007, -2.92, -1.92, 1.08, -4.92, 0.08000000000000007, -5.92, 11.08, -2.92, -1.92, -7.92, 0.08000000000000007, 4.08, 1.08, 3.08, -3.92, 11.08, 0.08000000000000007, 2.08, -6.92, -2.92, -0.9199999999999999, 0.08000000000000007, -5.92, -1.92, -3.92, -4.92, -0.9199999999999999, 3.08, -0.9199999999999999, -5.92, 0.08000000000000007, 7.08, 0.08000000000000007, 6.08, -4.92, 6.08, 1.08, 8.08, 4.08, -2.92, 2.08, 3.08, -2.92, -4.92, 0.08000000000000007, 2.08, 1.08, 3.08, 2.08, -4.92, 0.08000000000000007, 3.08, -2.92, -5.92, 4.08, 1.08, 3.08, 3.08, -1.92, 2.08, -0.9199999999999999, -0.9199999999999999, -1.92, 2.08, -1.92, -1.92, -3.92, -0.9199999999999999, 10.08, -3.92, -2.92, -15.92]] caption="Water Vapor Number Density"
  out "CH 3 (HSRL comb) counts display":dbl[][](graph)=[[95.56, 39.56, 42.56, 48.56, 64.56, 87.56, 139.56, 208.56, 315.56, 391.56, 464.56, 503.56, 501.56, 545.56, 575.56, 544.56, 504.56, 504.56, 483.56, 432.56, 381.56, 345.56, 328.56, 311.56, 279.56, 293.56, 273.56, 268.56, 256.56, 284.56, 271.56, 284.56, 285.56, 243.56, 257.56, 222.56, 269.56, 211.56, 174.56, 220.56, 219.56, 194.56, 194.56, 170.56, 179.56, 170.56, 152.56, 163.56, 154.56, 144.56, 119.56, 115.56, 127.56, 128.56, 127.56, 106.56, 104.56, 125.56, 84.56, 90.56, 85.56, 66.56, 76.56, 78.56, 94.56, 71.56, 61.56, 51.56, 50.56, 56.56, 75.56, 43.56, 40.56, 24.56, 48.56, 41.56, 25.56, 31.56, 32.56, 37.56, 26.56, 21.56, 26.56, 21.56, 23.56, 26.56, 29.56, 34.56, 14.559999999999999, 31.56, 16.56, 16.56, 18.56, 13.559999999999999, 21.56, 19.56, 7.559999999999999, 15.559999999999999, 16.56, 15.559999999999999, 15.559999999999999, 30.56, 18.56, 16.56, 4.559999999999999, 12.559999999999999, 8.559999999999999, 5.559999999999999, 13.559999999999999, 10.559999999999999, 14.559999999999999, 7.559999999999999, 13.559999999999999, 2.5599999999999987, 7.559999999999999, 11.559999999999999, 9.559999999999999, 8.559999999999999, 10.559999999999999, 7.559999999999999, 9.559999999999999, 8.559999999999999, 1.5599999999999987, 3.5599999999999987, -1.4400000000000013, 18.56, 2.5599999999999987, 2.5599999999999987, 1.5599999999999987, 7.559999999999999, 11.559999999999999, 13.559999999999999, 4.559999999999999, 6.559999999999999, 1.5599999999999987, 13.559999999999999, 5.559999999999999, 7.559999999999999, 1.5599999999999987, 3.5599999999999987, 3.5599999999999987, 0.5599999999999987, 6.559999999999999, 14.559999999999999, -5.440000000000001, 4.559999999999999, -0.4400000000000013, -2.4400000000000013, -1.4400000000000013, 2.5599999999999987, 10.559999999999999, 14.559999999999999, 10.559999999999999, 9.559999999999999, 4.559999999999999, -2.4400000000000013, 7.559999999999999, -5.440000000000001, -0.4400000000000013, 3.5599999999999987, -2.4400000000000013, -3.4400000000000013, 9.559999999999999, -0.4400000000000013, 7.559999999999999, 2.5599999999999987, 0.5599999999999987, 1.5599999999999987, 8.559999999999999, -2.4400000000000013, -3.4400000000000013, -2.4400000000000013, 1.5599999999999987, -0.4400000000000013, -2.4400000000000013, -3.4400000000000013, 9.559999999999999, -4.440000000000001, 9.559999999999999, 5.559999999999999, -2.4400000000000013, 6.559999999999999, 0.5599999999999987, 1.5599999999999987, -7.440000000000001, 8.559999999999999, -0.4400000000000013, 4.559999999999999, 2.5599999999999987, 2.5599999999999987, 2.5599999999999987, -7.440000000000001, -0.4400000000000013, 0.5599999999999987, 2.5599999999999987, -4.440000000000001, -2.4400000000000013, -6.440000000000001, -1.4400000000000013, 1.5599999999999987, 4.559999999999999, -1.4400000000000013, 3.5599999999999987, -1.4400000000000013, -4.440000000000001, 2.5599999999999987, 9.559999999999999, 7.559999999999999, 7.559999999999999, 1.5599999999999987, -4.440000000000001, -5.440000000000001, -8.440000000000001, 2.5599999999999987, 3.5599999999999987, -9.440000000000001, 3.5599999999999987, 1.5599999999999987, 1.5599999999999987, 6.559999999999999, 6.559999999999999, -1.4400000000000013, 1.5599999999999987, 2.5599999999999987, 7.559999999999999, -1.4400000000000013, -2.4400000000000013, 3.5599999999999987, -3.4400000000000013, -1.4400000000000013, 7.559999999999999, 0.5599999999999987, 3.5599999999999987, -5.440000000000001, 6.559999999999999, -3.4400000000000013, 0.5599999999999987, 0.5599999999999987, -0.4400000000000013, 10.559999999999999, 1.5599999999999987, -0.4400000000000013, -2.4400000000000013, -1.4400000000000013, 2.5599999999999987, 7.559999999999999, 12.559999999999999, 2.5599999999999987, -3.4400000000000013, 8.559999999999999, -1.4400000000000013, 2.5599999999999987, -2.4400000000000013, -2.4400000000000013, 6.559999999999999, -5.440000000000001, -3.4400000000000013, 10.559999999999999, 1.5599999999999987, -2.4400000000000013, 0.5599999999999987, 1.5599999999999987, 5.559999999999999, 1.5599999999999987, 3.5599999999999987, 1.5599999999999987, -2.4400000000000013, 1.5599999999999987, -3.4400000000000013, -0.4400000000000013, -4.440000000000001, 0.5599999999999987, 3.5599999999999987, -3.4400000000000013, 3.5599999999999987, -4.440000000000001, -5.440000000000001, -0.4400000000000013, -0.4400000000000013, 4.559999999999999, -0.4400000000000013, -1.4400000000000013, 8.559999999999999, -1.4400000000000013, 1.5599999999999987, -1.4400000000000013, -0.4400000000000013, 5.559999999999999, -3.4400000000000013, 7.559999999999999, 2.5599999999999987, 9.559999999999999, -3.4400000000000013, -1.4400000000000013, -1.4400000000000013, -1.4400000000000013, 2.5599999999999987, -4.440000000000001, -2.4400000000000013, -5.440000000000001, 3.5599999999999987, -4.440000000000001, -5.440000000000001, 3.5599999999999987, 3.5599999999999987, -5.440000000000001, 4.559999999999999, 1.5599999999999987, 3.5599999999999987, -0.4400000000000013, -5.440000000000001, 11.559999999999999, 2.5599999999999987, 1.5599999999999987, -8.440000000000001, 6.559999999999999, -2.4400000000000013, -3.4400000000000013, 4.559999999999999, 3.5599999999999987, 6.559999999999999, -2.4400000000000013, 5.559999999999999, -3.4400000000000013, 10.559999999999999, -1.4400000000000013, -2.4400000000000013, -1.4400000000000013, -5.440000000000001, 3.5599999999999987, -4.440000000000001, -2.4400000000000013, 6.559999999999999, 8.559999999999999, -4.440000000000001, 1.5599999999999987, 6.559999999999999, 3.5599999999999987, 2.5599999999999987, 5.559999999999999, 4.559999999999999, 5.559999999999999, 2.5599999999999987, 1.5599999999999987, 5.559999999999999, -3.4400000000000013, -7.440000000000001, 3.5599999999999987, 2.5599999999999987, 0.5599999999999987, 1.5599999999999987, 1.5599999999999987, -6.440000000000001, -0.4400000000000013, -0.4400000000000013, -0.4400000000000013, 1.5599999999999987, 2.5599999999999987, -1.4400000000000013, 9.559999999999999, 2.5599999999999987, -3.4400000000000013, 9.559999999999999, 1.5599999999999987, 2.5599999999999987, 2.5599999999999987, 2.5599999999999987, -1.4400000000000013, -3.4400000000000013, -0.4400000000000013, 6.559999999999999, -7.440000000000001, -0.4400000000000013, 3.5599999999999987, 0.5599999999999987, 2.5599999999999987, 7.559999999999999, -3.4400000000000013, 3.5599999999999987, 8.559999999999999, 3.5599999999999987, 3.5599999999999987, -0.4400000000000013, -1.4400000000000013, 3.5599999999999987, -1.4400000000000013, 3.5599999999999987, 1.5599999999999987, -1.4400000000000013, 2.5599999999999987, -4.440000000000001, 0.5599999999999987, 6.559999999999999, -0.4400000000000013, -2.4400000000000013, 5.559999999999999, -3.4400000000000013, 4.559999999999999, 2.5599999999999987, 8.559999999999999, -1.4400000000000013, -2.4400000000000013, -2.4400000000000013, 16.56, -4.440000000000001, 2.5599999999999987, -1.4400000000000013, 8.559999999999999, 0.5599999999999987, -9.440000000000001, -4.440000000000001, 4.559999999999999, -0.4400000000000013, 6.559999999999999, -2.4400000000000013, 1.5599999999999987, -1.4400000000000013, -6.440000000000001, -3.4400000000000013, 6.559999999999999, -4.440000000000001, -1.4400000000000013, 3.5599999999999987, 2.5599999999999987, -0.4400000000000013, -0.4400000000000013, -1.4400000000000013, -2.4400000000000013, -0.4400000000000013, 6.559999999999999, 0.5599999999999987, -5.440000000000001, 4.559999999999999, -5.440000000000001, -0.4400000000000013, 0.5599999999999987, 0.5599999999999987, -0.4400000000000013, 0.5599999999999987, 5.559999999999999, -7.440000000000001, -5.440000000000001, -1.4400000000000013, 3.5599999999999987, -7.440000000000001, 4.559999999999999, -3.4400000000000013, 6.559999999999999, 4.559999999999999, -3.4400000000000013, -5.440000000000001, 2.5599999999999987, -1.4400000000000013, -4.440000000000001, 3.5599999999999987, 3.5599999999999987, -3.4400000000000013, 6.559999999999999, -3.4400000000000013, -0.4400000000000013, 4.559999999999999, 3.5599999999999987, -3.4400000000000013, 2.5599999999999987, 1.5599999999999987, -3.4400000000000013, -6.440000000000001, -5.440000000000001, 3.5599999999999987, -2.4400000000000013, 1.5599999999999987, 6.559999999999999, -7.440000000000001, -1.4400000000000013, -7.440000000000001, 4.559999999999999, -2.4400000000000013, 0.5599999999999987, 11.559999999999999, 3.5599999999999987, 4.559999999999999, -10.440000000000001, -0.4400000000000013, 3.5599999999999987, 2.5599999999999987, -0.4400000000000013, 1.5599999999999987, 4.559999999999999, 7.559999999999999, -1.4400000000000013, -6.440000000000001, 0.5599999999999987, 4.559999999999999, -0.4400000000000013, -4.440000000000001, -1.4400000000000013, 4.559999999999999, 5.559999999999999, -3.4400000000000013, 2.5599999999999987, -4.440000000000001, 4.559999999999999, 2.5599999999999987, -0.4400000000000013, -5.440000000000001, 4.559999999999999, 5.559999999999999, 2.5599999999999987, 1.5599999999999987, 2.5599999999999987, 2.5599999999999987, 2.5599999999999987, 4.559999999999999, 2.5599999999999987, 1.5599999999999987, -6.440000000000001, 1.5599999999999987, 9.559999999999999, 3.5599999999999987, -1.4400000000000013, 8.559999999999999, 7.559999999999999, 2.5599999999999987, 0.5599999999999987, 9.559999999999999, -1.4400000000000013, -3.4400000000000013, -2.4400000000000013, -1.4400000000000013, 8.559999999999999, -0.4400000000000013, -4.440000000000001, 1.5599999999999987, 2.5599999999999987, -5.440000000000001, 0.5599999999999987, 0.5599999999999987, -1.4400000000000013, 0.5599999999999987, -2.4400000000000013, -4.440000000000001, 0.5599999999999987, 0.5599999999999987, 9.559999999999999, -3.4400000000000013, 7.559999999999999, 2.5599999999999987, 2.5599999999999987, 2.5599999999999987, -2.4400000000000013, -1.4400000000000013, 4.559999999999999, 2.5599999999999987, -5.440000000000001, -6.440000000000001, -1.4400000000000013, -1.4400000000000013, 1.5599999999999987, -0.4400000000000013, -17.44]] caption="Water Vapor Number Density"
  out "CH3 (HSRL combined) smooth":dbl[](array[numeric])=[57.592, 36.69199999999999, 44.391999999999996, 56.19199999999999, 79.892, 118.992, 181.692, 262.49199999999996, 333.992, 415.092, 477.892, 513.992, 540.5919999999999, 551.3919999999998, 557.492, 548.7919999999999, 523.792, 494.692, 481.49199999999996, 431.692, 357.992, 337.492, 322.89200000000005, 297.39200000000005, 284.39200000000005, 276.39200000000005, 269.492, 275.79200000000003, 275.592, 255.29199999999997, 250.892, 250.692, 247.79199999999997, 244.99199999999996, 233.89199999999997, 232.89199999999997, 223.99199999999996, 214.69199999999995, 211.59199999999998, 203.29199999999997, 200.09199999999998, 187.59199999999998, 168.192, 169.09199999999998, 172.29199999999997, 153.59199999999998, 141.49200000000002, 145.49200000000002, 142.592, 131.49200000000002, 122.59200000000001, 120.39200000000001, 121.69200000000001, 125.092, 115.092, 95.592, 92.092, 91.892, 84.99199999999999, 82.49199999999999, 77.49199999999999, 74.99199999999999, 72.99199999999999, 67.59199999999998, 63.69199999999999, 60.592, 57.592, 52.49199999999999, 51.99199999999999, 52.092, 49.992, 46.891999999999996, 40.391999999999996, 36.19199999999999, 39.092, 36.99199999999999, 30.591999999999995, 28.691999999999997, 28.291999999999998, 26.891999999999996, 26.491999999999997, 23.092, 22.891999999999996, 27.191999999999997, 24.891999999999996, 24.291999999999994, 26.092, 22.991999999999997, 20.092, 20.491999999999997, 17.592, 14.792, 16.692, 18.192, 16.991999999999997, 14.392, 14.791999999999998, 14.291999999999998, 14.091999999999997, 12.591999999999999, 15.091999999999999, 16.391999999999996, 11.791999999999998, 9.591999999999999, 11.392, 11.591999999999999, 8.691999999999998, 10.791999999999998, 8.892, 4.791999999999999, 7.091999999999999, 8.591999999999999, 9.291999999999998, 8.691999999999998, 6.391999999999999, 10.991999999999999, 14.691999999999998, 11.991999999999997, 12.291999999999998, 8.392, 7.8919999999999995, 8.892, 5.991999999999999, 3.0919999999999987, 2.9919999999999987, 5.591999999999999, 4.3919999999999995, 3.691999999999999, 4.791999999999998, 7.791999999999999, 6.3919999999999995, 7.091999999999999, 9.591999999999999, 6.291999999999999, 5.391999999999999, 10.191999999999998, 7.391999999999999, 0.9919999999999987, 1.3919999999999988, 3.791999999999999, 7.091999999999999, 7.591999999999999, 5.3919999999999995, 3.391999999999999, 5.791999999999998, 6.891999999999999, 2.5919999999999987, 1.8919999999999988, 4.591999999999999, 5.391999999999999, 4.791999999999998, 4.391999999999999, 1.8919999999999986, 5.091999999999999, 6.091999999999999, 2.5919999999999987, 1.0919999999999987, 3.0919999999999987, 4.791999999999999, 2.791999999999999, 0.6919999999999988, 1.0919999999999987, 0.3919999999999988, -0.2080000000000013, 4.491999999999999, 5.191999999999998, 3.491999999999999, 5.091999999999999, 2.691999999999999, -0.7080000000000012, 2.0919999999999987, 3.791999999999999, 2.191999999999999, 1.1919999999999988, 0.2919999999999987, 4.491999999999999, 6.191999999999998, 2.3919999999999986, 4.391999999999999, 4.591999999999999, 2.0919999999999987, 1.9919999999999987, 4.291999999999999, 2.891999999999999, 4.191999999999998, 5.891999999999999, 1.6919999999999988, 0.19199999999999875, 0.7919999999999988, 0.19199999999999873, 1.5919999999999985, -0.3080000000000016, -0.7080000000000015, 5.191999999999998, 3.891999999999999, -0.2080000000000013, 1.1919999999999988, 0.49199999999999866, -0.5080000000000013, 2.691999999999999, 3.191999999999999, -0.1080000000000012, -2.508000000000001, -0.7080000000000012, 2.4919999999999987, 4.291999999999998, 2.9919999999999987, 3.191999999999999, 4.191999999999998, 2.5919999999999987, -0.5080000000000013, -0.9080000000000014, 0.8919999999999988, 1.4919999999999987, 3.0919999999999987, 4.491999999999999, 1.9919999999999989, -1.2080000000000013, -0.3080000000000012, 1.3919999999999988, 0.9919999999999988, 0.4919999999999987, 3.4919999999999987, 4.091999999999999, 2.8919999999999986, 2.0919999999999987, -0.6080000000000012, -0.7080000000000012, -1.2080000000000013, 0.09199999999999875, 2.0919999999999987, 1.0919999999999987, -0.3080000000000013, -1.2080000000000013, -0.6080000000000013, 1.1919999999999988, 2.791999999999999, 1.8919999999999986, 2.4919999999999987, 2.4919999999999987, 1.1919999999999988, -0.6080000000000012, 0.2919999999999987, 3.9919999999999987, 2.691999999999999, 1.0919999999999987, 1.791999999999999, 4.991999999999999, 6.191999999999998, -0.00800000000000134, -3.0080000000000013, -0.1080000000000012, 1.5919999999999987, 4.491999999999999, 1.591999999999999, 0.3919999999999988, 3.9919999999999987, 1.4919999999999987, -0.20800000000000124, 1.2919999999999987, 3.691999999999999, 4.391999999999999, 2.5919999999999987, 0.7919999999999988, 2.7919999999999985, 2.9919999999999987, 1.1919999999999988, -0.9080000000000013, -1.9080000000000013, -0.008000000000001256, 0.29199999999999876, -0.9080000000000013, -1.7080000000000013, -0.3080000000000013, 1.1919999999999988, 0.49199999999999877, -0.3080000000000012, 0.39199999999999874, 0.4919999999999987, -1.1080000000000012, -2.708000000000001, -1.6080000000000012, 0.7919999999999987, 2.4919999999999987, -0.5080000000000011, -1.5080000000000011, 0.19199999999999878, -0.5080000000000012, 0.8919999999999987, 2.4919999999999987, 3.8919999999999986, 1.6919999999999988, -2.0080000000000013, -1.2080000000000013, 0.7919999999999988, -0.008000000000001228, -1.9080000000000013, -1.8080000000000012, -1.1080000000000014, 0.09199999999999875, 0.5919999999999987, 1.2919999999999987, 3.691999999999999, 2.5919999999999987, -0.9080000000000011, -0.20800000000000118, 1.6919999999999988, 2.9919999999999987, 1.7919999999999987, -0.10800000000000126, 2.0919999999999987, 1.0919999999999987, -2.1080000000000014, -1.2080000000000013, 0.8919999999999988, 0.8919999999999988, 1.2919999999999987, -0.008000000000001117, 0.4919999999999989, 3.491999999999999, -0.10800000000000098, -2.008000000000001, 1.4919999999999987, -0.00800000000000134, -0.6080000000000013, 0.2919999999999987, 0.2919999999999987, 1.5919999999999987, 0.8919999999999988, -3.808000000000001, -4.808000000000001, -1.1080000000000012, 1.9919999999999987, 2.4919999999999987, -0.008000000000001256, 1.2919999999999987, 3.0919999999999987, 2.291999999999999, -0.1080000000000012, 2.2919999999999985, 3.0919999999999987, 0.29199999999999876, 0.49199999999999877, 1.3919999999999986, -0.10800000000000143, -0.2080000000000013, 1.8919999999999988, 2.691999999999999, 3.9919999999999987, 3.0919999999999987, 2.3919999999999986, 1.1919999999999988, 2.5919999999999987, 2.5919999999999987, 0.5919999999999987, -0.2080000000000013, 0.09199999999999875, 0.7919999999999988, 1.291999999999999, 3.491999999999999, 0.9919999999999989, 2.491999999999999, 5.791999999999999, 3.691999999999999, 2.3919999999999986, 1.791999999999999, 1.9919999999999987, 3.791999999999999, 3.491999999999999, 1.4919999999999987, -0.20800000000000124, -2.5080000000000013, -1.2080000000000013, 0.09199999999999875, 1.5919999999999985, 2.6919999999999984, -1.3080000000000012, -3.708000000000001, -1.1080000000000014, 2.291999999999999, 1.5919999999999987, -1.0080000000000013, -1.1080000000000012, -1.1080000000000012, 0.49199999999999866, 4.091999999999999, 4.991999999999999, 2.891999999999999, 1.9919999999999987, 1.4919999999999987, -1.3080000000000014, -1.0080000000000013, 0.09199999999999875, 0.19199999999999873, 0.9919999999999988, 2.6919999999999984, 2.9919999999999987, 0.5919999999999987, 3.191999999999999, 2.991999999999999, -0.9080000000000013, -0.6080000000000012, 2.4919999999999987, 4.091999999999999, 2.0919999999999987, 1.9919999999999987, 2.9919999999999987, 2.3919999999999986, 0.5919999999999987, 0.2919999999999987, 0.2919999999999987, -0.7080000000000013, 1.0919999999999987, 1.4919999999999987, -1.0080000000000013, 0.6919999999999987, 1.0919999999999987, 1.8919999999999988, -0.6080000000000014, -3.9080000000000013, 0.09199999999999875, 1.6919999999999988, -0.9080000000000013, -1.5080000000000013, 0.5919999999999987, -0.1080000000000012, -2.1080000000000014, -4.208000000000001, 0.09199999999999875, 6.191999999999998, 4.191999999999998, 2.3919999999999986, -0.6080000000000012, -2.5080000000000013, -1.1080000000000012, -0.008000000000001228, -0.5080000000000012, -3.308000000000001, -1.3080000000000012, 0.09199999999999875, -2.808000000000001, -3.008000000000001, -1.9080000000000013, -3.9080000000000013, -1.8080000000000014, 1.3919999999999988, 0.5919999999999987, -0.008000000000001228, -2.4080000000000013, -3.6080000000000014, -2.208000000000001, -0.008000000000001228, 1.8919999999999986, 3.9919999999999987, 2.9919999999999987, 0.29199999999999876, 1.7919999999999987, 2.191999999999999, 1.4919999999999987, 1.4919999999999987, 2.891999999999999, 3.0919999999999987, 1.791999999999999, 1.4919999999999987, 0.6919999999999987, -0.5080000000000012, -0.9080000000000013, 0.09199999999999875, -1.0080000000000013, 0.5919999999999987, 4.291999999999999, 1.591999999999999, -1.208000000000001, 1.3919999999999986, 2.791999999999999, 0.2919999999999988, -2.308000000000001, -1.9080000000000013, -1.0080000000000013, -0.10800000000000126, -0.9080000000000013, -0.008000000000001117, 3.9919999999999987, 2.8919999999999986, 1.8919999999999988, -1.2080000000000013, -3.3080000000000016, 0.09199999999999875, -1.1080000000000012, -0.5080000000000013, 2.6919999999999984, 2.9919999999999987, 2.0919999999999987, -0.8080000000000012, -1.708000000000001, 1.7919999999999985, 1.8919999999999986, -0.7080000000000013, 0.19199999999999873, -0.1080000000000012, 1.2919999999999985, 3.3919999999999986, 1.8919999999999988, 3.0919999999999987, 2.791999999999999, 1.8919999999999988, 3.291999999999999, 0.6919999999999986, -0.9080000000000013, -0.20800000000000124, -0.6080000000000012, -1.4080000000000013, -3.808000000000001, -2.308000000000001, -0.008000000000001284, 0.7919999999999987, 4.191999999999998, 3.391999999999999, -1.9080000000000013, -0.00800000000000134, 0.8919999999999988, -0.30800000000000116, 3.1919999999999984, 4.891999999999999, 1.6919999999999988, -3.008000000000001, -1.5080000000000013, 1.4919999999999987, 2.791999999999999, 1.4919999999999987, -2.0080000000000013, -1.2080000000000013, -0.7080000000000013, -2.8080000000000016, -1.8080000000000012, 0.7919999999999988, -0.008000000000001117, 1.1919999999999988, 1.6919999999999988, -2.0080000000000013, -2.1080000000000014, -0.8080000000000013, 3.891999999999999, 2.0919999999999987, -0.5080000000000011, 1.6919999999999988, -0.6080000000000012, -3.208000000000001, -1.3080000000000014, -0.3080000000000014, -1.0080000000000013, 0.39199999999999874, 0.7919999999999988, 0.8919999999999988, 2.0919999999999987, 1.3919999999999988, 0.49199999999999866, -0.6080000000000012]
  out "CH3 Bin Readings":dbl[](array[numeric])=[113.0, 57.0, 60.0, 66.0, 82.0, 105.0, 157.0, 226.0, 333.0, 409.0, 482.0, 521.0, 519.0, 563.0, 593.0, 562.0, 522.0, 522.0, 501.0, 450.0, 399.0, 363.0, 346.0, 329.0, 297.0, 311.0, 291.0, 286.0, 274.0, 302.0, 289.0, 302.0, 303.0, 261.0, 275.0, 240.0, 287.0, 229.0, 192.0, 238.0, 237.0, 212.0, 212.0, 188.0, 197.0, 188.0, 170.0, 181.0, 172.0, 162.0, 137.0, 133.0, 145.0, 146.0, 145.0, 124.0, 122.0, 143.0, 102.0, 108.0, 103.0, 84.0, 94.0, 96.0, 112.0, 89.0, 79.0, 69.0, 68.0, 74.0, 93.0, 61.0, 58.0, 42.0, 66.0, 59.0, 43.0, 49.0, 50.0, 55.0, 44.0, 39.0, 44.0, 39.0, 41.0, 44.0, 47.0, 52.0, 32.0, 49.0, 34.0, 34.0, 36.0, 31.0, 39.0, 37.0, 25.0, 33.0, 34.0, 33.0, 33.0, 48.0, 36.0, 34.0, 22.0, 30.0, 26.0, 23.0, 31.0, 28.0, 32.0, 25.0, 31.0, 20.0, 25.0, 29.0, 27.0, 26.0, 28.0, 25.0, 27.0, 26.0, 19.0, 21.0, 16.0, 36.0, 20.0, 20.0, 19.0, 25.0, 29.0, 31.0, 22.0, 24.0, 19.0, 31.0, 23.0, 25.0, 19.0, 21.0, 21.0, 18.0, 24.0, 32.0, 12.0, 22.0, 17.0, 15.0, 16.0, 20.0, 28.0, 32.0, 28.0, 27.0, 22.0, 15.0, 25.0, 12.0, 17.0, 21.0, 15.0, 14.0, 27.0, 17.0, 25.0, 20.0, 18.0, 19.0, 26.0, 15.0, 14.0, 15.0, 19.0, 17.0, 15.0, 14.0, 27.0, 13.0, 27.0, 23.0, 15.0, 24.0, 18.0, 19.0, 10.0, 26.0, 17.0, 22.0, 20.0, 20.0, 20.0, 10.0, 17.0, 18.0, 20.0, 13.0, 15.0, 11.0, 16.0, 19.0, 22.0, 16.0, 21.0, 16.0, 13.0, 20.0, 27.0, 25.0, 25.0, 19.0, 13.0, 12.0, 9.0, 20.0, 21.0, 8.0, 21.0, 19.0, 19.0, 24.0, 24.0, 16.0, 19.0, 20.0, 25.0, 16.0, 15.0, 21.0, 14.0, 16.0, 25.0, 18.0, 21.0, 12.0, 24.0, 14.0, 18.0, 18.0, 17.0, 28.0, 19.0, 17.0, 15.0, 16.0, 20.0, 25.0, 30.0, 20.0, 14.0, 26.0, 16.0, 20.0, 15.0, 15.0, 24.0, 12.0, 14.0, 28.0, 19.0, 15.0, 18.0, 19.0, 23.0, 19.0, 21.0, 19.0, 15.0, 19.0, 14.0, 17.0, 13.0, 18.0, 21.0, 14.0, 21.0, 13.0, 12.0, 17.0, 17.0, 22.0, 17.0, 16.0, 26.0, 16.0, 19.0, 16.0, 17.0, 23.0, 14.0, 25.0, 20.0, 27.0, 14.0, 16.0, 16.0, 16.0, 20.0, 13.0, 15.0, 12.0, 21.0, 13.0, 12.0, 21.0, 21.0, 12.0, 22.0, 19.0, 21.0, 17.0, 12.0, 29.0, 20.0, 19.0, 9.0, 24.0, 15.0, 14.0, 22.0, 21.0, 24.0, 15.0, 23.0, 14.0, 28.0, 16.0, 15.0, 16.0, 12.0, 21.0, 13.0, 15.0, 24.0, 26.0, 13.0, 19.0, 24.0, 21.0, 20.0, 23.0, 22.0, 23.0, 20.0, 19.0, 23.0, 14.0, 10.0, 21.0, 20.0, 18.0, 19.0, 19.0, 11.0, 17.0, 17.0, 17.0, 19.0, 20.0, 16.0, 27.0, 20.0, 14.0, 27.0, 19.0, 20.0, 20.0, 20.0, 16.0, 14.0, 17.0, 24.0, 10.0, 17.0, 21.0, 18.0, 20.0, 25.0, 14.0, 21.0, 26.0, 21.0, 21.0, 17.0, 16.0, 21.0, 16.0, 21.0, 19.0, 16.0, 20.0, 13.0, 18.0, 24.0, 17.0, 15.0, 23.0, 14.0, 22.0, 20.0, 26.0, 16.0, 15.0, 15.0, 34.0, 13.0, 20.0, 16.0, 26.0, 18.0, 8.0, 13.0, 22.0, 17.0, 24.0, 15.0, 19.0, 16.0, 11.0, 14.0, 24.0, 13.0, 16.0, 21.0, 20.0, 17.0, 17.0, 16.0, 15.0, 17.0, 24.0, 18.0, 12.0, 22.0, 12.0, 17.0, 18.0, 18.0, 17.0, 18.0, 23.0, 10.0, 12.0, 16.0, 21.0, 10.0, 22.0, 14.0, 24.0, 22.0, 14.0, 12.0, 20.0, 16.0, 13.0, 21.0, 21.0, 14.0, 24.0, 14.0, 17.0, 22.0, 21.0, 14.0, 20.0, 19.0, 14.0, 11.0, 12.0, 21.0, 15.0, 19.0, 24.0, 10.0, 16.0, 10.0, 22.0, 15.0, 18.0, 29.0, 21.0, 22.0, 7.0, 17.0, 21.0, 20.0, 17.0, 19.0, 22.0, 25.0, 16.0, 11.0, 18.0, 22.0, 17.0, 13.0, 16.0, 22.0, 23.0, 14.0, 20.0, 13.0, 22.0, 20.0, 17.0, 12.0, 22.0, 23.0, 20.0, 19.0, 20.0, 20.0, 20.0, 22.0, 20.0, 19.0, 11.0, 19.0, 27.0, 21.0, 16.0, 26.0, 25.0, 20.0, 18.0, 27.0, 16.0, 14.0, 15.0, 16.0, 26.0, 17.0, 13.0, 19.0, 20.0, 12.0, 18.0, 18.0, 16.0, 18.0, 15.0, 13.0, 18.0, 18.0, 27.0, 14.0, 25.0, 20.0, 20.0, 20.0, 15.0, 16.0, 22.0, 20.0, 12.0, 11.0, 16.0, 16.0, 19.0, 17.0, 0.0]
  out "CH2 (molecular) smoothed":dbl[](array[numeric])=[5.228, 6.728, 10.728, 11.628, 14.328000000000003, 25.628, 54.228, 76.128, 94.628, 121.228, 129.028, 138.728, 151.928, 164.32800000000003, 160.62800000000001, 144.128, 145.52800000000002, 136.828, 133.228, 143.428, 131.028, 126.62799999999999, 129.328, 117.128, 113.428, 118.728, 112.228, 103.228, 106.328, 105.128, 106.128, 106.02799999999999, 101.02799999999999, 97.328, 89.728, 87.62799999999999, 91.228, 87.728, 80.828, 78.72800000000001, 79.02799999999999, 76.728, 71.52799999999999, 71.72800000000001, 68.428, 61.02799999999999, 53.528, 49.528, 50.128, 47.828, 40.428, 39.628, 46.228, 42.628, 35.528000000000006, 36.028000000000006, 36.928000000000004, 30.628000000000004, 29.728, 34.028000000000006, 35.328, 33.228, 29.128, 23.728, 25.528000000000006, 26.928000000000004, 21.228, 21.228, 22.928000000000004, 19.128000000000004, 17.428000000000004, 20.028000000000002, 23.328000000000003, 21.728, 18.628000000000004, 16.728, 10.728, 8.228, 13.328000000000001, 13.128000000000002, 9.428, 12.728000000000002, 14.528, 13.628, 15.128, 13.228000000000002, 8.328, 12.928, 18.128000000000004, 16.428, 14.328, 12.228000000000002, 4.828, 2.128, 8.328, 6.928000000000001, 2.728, 3.028, 2.3280000000000003, 2.5280000000000005, 4.728, 9.428, 6.428, 0.5280000000000001, 1.3280000000000003, 2.728, 3.128, 4.428, 6.328, 4.928, 4.0280000000000005, 4.128, 2.8280000000000003, 4.428, 5.328, 2.128, 1.4280000000000002, 0.2280000000000002, 0.8280000000000001, 4.828, 7.128, 1.7280000000000002, -2.9719999999999995, 1.728, 1.728, 3.928, 6.0280000000000005, 3.528, 1.528, 0.3280000000000002, 0.42800000000000016, 2.228, 3.128, 1.2280000000000002, 0.528, -1.5719999999999998, -2.372, -0.6719999999999999, 1.6280000000000001, 4.728, 3.428, 1.728, 1.728, 1.228, 3.128, -1.8719999999999997, -3.0719999999999996, -1.3719999999999999, 1.928, 4.828, 0.9280000000000002, 2.928, 4.128, 1.328, 1.6280000000000001, 3.428, 2.528, 2.528, 2.8280000000000003, 5.428000000000001, 6.428000000000001, 3.928, -0.6720000000000002, -4.172000000000001, -1.572, 1.228, 2.8280000000000003, 1.828, 0.8280000000000001, 4.228, 4.628, 2.228, 4.328, 1.9280000000000002, -1.7719999999999998, 1.728, 1.128, 2.8280000000000003, 4.728, 2.228, 1.7280000000000002, 0.1280000000000001, -0.7719999999999999, -0.8719999999999999, 2.828, 3.328, 0.02800000000000008, -0.9719999999999999, 0.6280000000000001, 3.2279999999999998, -0.07200000000000006, -1.672, -0.17199999999999988, -0.9719999999999999, -0.0719999999999999, 1.828, -0.8719999999999999, -0.5719999999999998, 3.028, 0.528, -0.4719999999999999, -0.0719999999999999, 0.1280000000000001, 5.228000000000001, 7.228, 1.328, -2.1719999999999997, -3.072, -0.8719999999999999, 2.428, -0.17199999999999993, -2.972, -2.072, 1.028, 4.328, 5.128, 0.32799999999999985, -0.772, 0.8280000000000001, 0.32800000000000007, 5.428, 7.128, 2.928, 1.028, -0.2719999999999999, 0.1280000000000001, 0.6280000000000001, -2.1719999999999997, -0.5719999999999998, 1.4280000000000002, 1.7280000000000002, 4.0280000000000005, 1.428, -2.072, -1.3719999999999999, 1.428, 1.1280000000000001, -0.07199999999999984, 2.028, 0.528, 0.528, -0.472, -2.472, 1.6280000000000001, 3.928, 2.228, -2.672, -1.372, -0.5719999999999998, -2.372, 3.728, 2.3280000000000003, -0.9719999999999999, 2.528, 0.9280000000000002, 0.2280000000000002, 1.4280000000000002, 2.128, 1.9280000000000002, -2.672, -1.8719999999999999, 1.928, 1.828, -0.7719999999999998, -4.272, -0.07200000000000006, 5.628, 1.7280000000000002, 1.8279999999999998, 3.828, 0.5280000000000001, -0.7719999999999999, 0.928, 2.7279999999999998, 1.028, -2.772, -0.47199999999999975, -1.0719999999999998, -4.4719999999999995, -2.6719999999999997, -1.0719999999999998, -0.8719999999999999, 0.8280000000000001, 3.2279999999999998, 2.628, 1.2280000000000002, -2.372, -2.372, 0.3280000000000001, -2.6719999999999997, -0.2719999999999998, 2.3280000000000003, -0.3719999999999999, -0.9719999999999999, -1.2719999999999998, -0.7719999999999999, 0.5280000000000001, 4.928, 3.928, -0.9719999999999999, -3.1719999999999997, -3.272, -2.372, -3.5719999999999996, -1.2719999999999998, 2.128, 1.9280000000000002, -1.372, -0.972, 1.9280000000000002, 1.1280000000000001, -0.8719999999999999, -2.072, -0.8719999999999999, 1.028, 0.42800000000000016, -0.9719999999999999, 2.028, 3.428, -0.07199999999999984, -3.9719999999999995, -4.572, -0.272, 2.028, 2.928, 3.7279999999999998, 1.9280000000000002, 4.128, 0.9279999999999999, -1.472, -2.772, -4.872, -1.8719999999999999, -1.7719999999999998, -0.17199999999999993, 0.7280000000000001, -0.47199999999999986, 0.5280000000000001, 4.328, 5.428000000000001, 3.8280000000000003, 0.1280000000000001, -2.872, -1.7719999999999998, 1.6280000000000001, 3.728, -1.1719999999999997, -5.172, -3.072, -2.2720000000000002, -4.272, -2.1719999999999997, 2.628, 2.228, -0.572, -2.072, -2.6719999999999997, -3.372, -5.272, -3.0719999999999996, 1.5280000000000002, 1.7280000000000002, 0.5280000000000001, 3.028, 3.7279999999999998, -0.7719999999999998, -3.4719999999999995, 1.6280000000000001, 3.828, 1.7280000000000002, 1.6280000000000001, 0.22800000000000012, 2.028, 3.628, 4.0280000000000005, 3.428, 0.2280000000000001, 0.8280000000000001, 3.528, 7.327999999999999, 4.628, -1.572, -2.6719999999999997, -0.7719999999999998, -1.3719999999999999, -2.572, 2.028, 4.228, 4.228, 1.3280000000000003, -0.6719999999999999, -1.7719999999999998, 0.2280000000000002, 3.228, 0.9280000000000002, -2.2720000000000002, -3.972, 2.228, 3.8280000000000003, 3.228, 3.028, 0.9280000000000002, 3.428, 1.7280000000000002, -2.072, -2.072, 3.228, 2.128, 0.6280000000000001, 1.4280000000000002, -0.8719999999999999, 1.528, -1.172, -5.372, -0.07200000000000006, 3.428, 0.9280000000000002, -0.4719999999999999, 0.32800000000000007, 0.6280000000000001, 1.028, 1.6280000000000001, -1.3719999999999999, -1.0719999999999998, 0.3280000000000002, -1.972, 0.1280000000000001, 4.328, 2.128, -0.6719999999999998, 2.728, 0.5280000000000005, -1.7719999999999998, 0.9280000000000002, 1.028, -0.3719999999999999, 0.2280000000000002, 1.9280000000000002, 0.7280000000000001, -1.072, -4.172000000000001, -0.3719999999999999, 2.128, 0.7280000000000002, 2.8280000000000003, -0.7719999999999998, 0.4280000000000004, 2.3280000000000003, -0.9719999999999999, -1.0719999999999998, -4.372, -2.072, 2.728, -1.4719999999999998, -1.4719999999999998, -0.7719999999999998, -0.7719999999999998, 1.9280000000000002, 5.428, 3.028, -2.6719999999999997, -2.572, -1.7719999999999998, -1.572, -3.972, -0.7719999999999998, 5.128, 4.728, 2.228, 1.2280000000000002, 1.528, -0.3719999999999999, -1.972, 1.028, 0.2280000000000002, -3.272, 1.328, 3.128, -0.2719999999999999, 1.1280000000000001, -0.3719999999999999, -0.2719999999999998, 2.428, 3.2279999999999998, 3.8280000000000003, 1.5280000000000002, 3.128, 2.928, -0.47199999999999986, 0.7280000000000002, 2.0280000000000005, -3.4720000000000004, -7.472, -1.572, 2.428, 2.0280000000000005, -2.372, -2.972, 3.728, 3.628, 0.22800000000000015, -2.1719999999999997, 0.8280000000000003, 3.3280000000000003, -0.6719999999999999, -0.572, 2.8280000000000003, 3.3280000000000003, 2.228, 4.5280000000000005, 3.628, 0.7280000000000001, -1.172, -0.3719999999999999, -0.6719999999999999, -0.3719999999999999, 2.928, -1.4719999999999998, -0.9719999999999998, 3.628, 1.7280000000000002, 1.0280000000000002, 3.3280000000000003, 1.9280000000000002, -0.7719999999999998, -1.0719999999999998, -0.27199999999999985, 0.1280000000000001, -0.7719999999999998, -2.272, -0.17199999999999993, -0.6720000000000002, -4.4719999999999995, -4.672, -2.272, -0.0719999999999999, 0.1280000000000001, 0.7280000000000002, -1.1719999999999997, 1.5280000000000002, 3.4280000000000004, -0.4719999999999999, -1.2719999999999998, -3.472, -5.072, -4.772, -3.372, 1.9280000000000002, 1.3280000000000003, 1.7280000000000002, 6.228, 4.0280000000000005, -1.672, -0.07200000000000006, 3.528, -1.6719999999999997, -0.3719999999999999, 2.928]
  out "CH 2 Bin Readings":dbl[](array[numeric])=[41.0, 46.0, 34.0, 46.0, 41.0, 51.0, 78.0, 91.0, 123.0, 152.0, 145.0, 176.0, 186.0, 184.0, 212.0, 161.0, 183.0, 143.0, 154.0, 175.0, 160.0, 155.0, 166.0, 176.0, 146.0, 167.0, 159.0, 152.0, 139.0, 149.0, 139.0, 135.0, 112.0, 141.0, 109.0, 133.0, 122.0, 97.0, 115.0, 96.0, 110.0, 105.0, 101.0, 117.0, 119.0, 100.0, 81.0, 91.0, 83.0, 81.0, 78.0, 77.0, 88.0, 89.0, 78.0, 74.0, 75.0, 79.0, 60.0, 78.0, 63.0, 73.0, 76.0, 62.0, 60.0, 78.0, 50.0, 51.0, 52.0, 56.0, 56.0, 53.0, 48.0, 46.0, 64.0, 51.0, 41.0, 43.0, 44.0, 60.0, 46.0, 53.0, 57.0, 41.0, 46.0, 52.0, 41.0, 31.0, 43.0, 45.0, 46.0, 56.0, 45.0, 32.0, 32.0, 44.0, 30.0, 42.0, 43.0, 31.0, 39.0, 35.0, 36.0, 33.0, 29.0, 39.0, 39.0, 41.0, 42.0, 40.0, 50.0, 31.0, 35.0, 46.0, 37.0, 29.0, 37.0, 32.0, 39.0, 42.0, 37.0, 41.0, 23.0, 28.0, 34.0, 30.0, 50.0, 33.0, 37.0, 23.0, 35.0, 26.0, 37.0, 27.0, 42.0, 32.0, 39.0, 40.0, 34.0, 43.0, 31.0, 28.0, 28.0, 28.0, 37.0, 45.0, 37.0, 39.0, 32.0, 38.0, 29.0, 35.0, 29.0, 39.0, 31.0, 36.0, 33.0, 37.0, 27.0, 38.0, 39.0, 42.0, 46.0, 44.0, 31.0, 24.0, 33.0, 28.0, 35.0, 46.0, 33.0, 34.0, 29.0, 49.0, 49.0, 32.0, 40.0, 28.0, 45.0, 39.0, 40.0, 44.0, 36.0, 31.0, 31.0, 32.0, 42.0, 39.0, 34.0, 35.0, 32.0, 28.0, 38.0, 29.0, 38.0, 28.0, 35.0, 25.0, 42.0, 31.0, 27.0, 31.0, 33.0, 37.0, 42.0, 39.0, 39.0, 40.0, 36.0, 26.0, 31.0, 34.0, 29.0, 29.0, 34.0, 34.0, 40.0, 30.0, 43.0, 32.0, 32.0, 45.0, 23.0, 41.0, 34.0, 34.0, 36.0, 37.0, 32.0, 37.0, 34.0, 36.0, 41.0, 32.0, 28.0, 27.0, 52.0, 34.0, 32.0, 33.0, 31.0, 23.0, 33.0, 27.0, 32.0, 34.0, 33.0, 35.0, 28.0, 31.0, 32.0, 36.0, 34.0, 41.0, 37.0, 33.0, 38.0, 37.0, 43.0, 29.0, 27.0, 41.0, 37.0, 26.0, 35.0, 27.0, 31.0, 44.0, 24.0, 33.0, 46.0, 34.0, 33.0, 39.0, 47.0, 28.0, 37.0, 33.0, 35.0, 23.0, 29.0, 27.0, 33.0, 32.0, 33.0, 44.0, 39.0, 28.0, 33.0, 23.0, 23.0, 37.0, 33.0, 26.0, 37.0, 29.0, 32.0, 40.0, 28.0, 34.0, 43.0, 38.0, 30.0, 23.0, 34.0, 42.0, 36.0, 36.0, 35.0, 26.0, 44.0, 36.0, 36.0, 44.0, 44.0, 37.0, 40.0, 27.0, 36.0, 31.0, 29.0, 20.0, 23.0, 35.0, 32.0, 42.0, 32.0, 36.0, 42.0, 32.0, 36.0, 31.0, 37.0, 29.0, 36.0, 45.0, 33.0, 45.0, 31.0, 39.0, 28.0, 37.0, 23.0, 27.0, 38.0, 51.0, 39.0, 30.0, 43.0, 25.0, 39.0, 31.0, 30.0, 27.0, 32.0, 41.0, 41.0, 21.0, 24.0, 30.0, 42.0, 34.0, 32.0, 44.0, 25.0, 33.0, 28.0, 28.0, 31.0, 32.0, 42.0, 29.0, 36.0, 33.0, 36.0, 43.0, 44.0, 27.0, 40.0, 34.0, 26.0, 23.0, 28.0, 30.0, 29.0, 32.0, 29.0, 36.0, 37.0, 38.0, 40.0, 36.0, 35.0, 36.0, 35.0, 33.0, 35.0, 26.0, 43.0, 28.0, 29.0, 34.0, 40.0, 41.0, 33.0, 27.0, 39.0, 38.0, 32.0, 41.0, 32.0, 22.0, 34.0, 35.0, 34.0, 46.0, 33.0, 39.0, 33.0, 37.0, 34.0, 35.0, 42.0, 29.0, 45.0, 29.0, 34.0, 42.0, 28.0, 36.0, 24.0, 34.0, 30.0, 51.0, 39.0, 40.0, 33.0, 44.0, 36.0, 44.0, 30.0, 35.0, 40.0, 40.0, 34.0, 47.0, 24.0, 49.0, 37.0, 32.0, 36.0, 31.0, 33.0, 35.0, 35.0, 41.0, 32.0, 35.0, 45.0, 38.0, 23.0, 39.0, 26.0, 31.0, 20.0, 33.0, 38.0, 44.0, 24.0, 33.0, 40.0, 42.0, 29.0, 34.0, 35.0, 32.0, 32.0, 38.0, 36.0, 34.0, 42.0, 29.0, 37.0, 28.0, 43.0, 34.0, 40.0, 38.0, 32.0, 34.0, 34.0, 35.0, 35.0, 25.0, 34.0, 33.0, 40.0, 31.0, 34.0, 40.0, 33.0, 38.0, 37.0, 30.0, 28.0, 28.0, 39.0, 46.0, 40.0, 39.0, 37.0, 20.0, 38.0, 29.0, 36.0, 28.0, 35.0, 39.0, 35.0, 38.0, 33.0, 37.0, 44.0, 44.0, 32.0, 39.0, 31.0, 39.0, 31.0, 32.0, 34.0, 45.0, 29.0, 27.0, 27.0, 35.0, 29.0, 41.0, 33.0, 30.0, 38.0, 37.0, 27.0, 33.0, 33.0, 33.0, 24.0, 41.0, 35.0, 31.0, 37.0, 36.0, 39.0, 33.0, 31.0, 43.0, 27.0, 36.0, 36.0, 0.0]
  in  "stop":bool
  in  "Reset Average":bool=TRUE
  in  "Save Data?":bool=TRUE
  in  "Collect Data?":bool=TRUE
  in  "ILX Address":i32=6 min=0 step=1
  in  "Lambda On DBR Current":dbl=171.13999999999868
  in  "Lambda Off DBR Current":dbl=172.9499999999997
  in  "Tab Control":T2(tab)=enum."OD"
  out "Water Vapor Number Density":cluster{"Y":dbl[], "Y":dbl[]}[](graph)
  out "Absolute Humidity":cluster{"Y":dbl[], "Y":dbl[]}[](graph)
  out "NRB plot":cluster{"Y":dbl[], "Y":dbl[]}[](graph)
  in  "background length":i32=25
  out "Correction":cluster{"Y":dbl[], "Y":dbl[]}[](graph)
  in  "dead time":dbl=3.7e-08
  out "Optical Depth":cluster{"Y":dbl[], "Y":dbl[]}[](graph) caption="XY Graph"
  out "aerosol profile":cluster{"Y":dbl[], "Y":dbl[]}[](graph)
  out "CH1 RingBuffer long":dbl[][](array[numeric])
  in  "Weather":T3(tab)=enum."Relative Humidity"
  out "Temperature (C)":dbl(graph)=28.47237484737485
  out "Pressure (mb)":dbl(graph)=984.8763736263736
  out "Relative Humdity (%)":dbl(graph)=48.827838827838825
  out "Pulse Energy (Micro Joule)":T4(graph)={"Online Pulse Energy"=5.263724285714285, "Pulse Energy Offline"=5.265377142857142}
  out "?":cluster{"mean":dbl, "mean":dbl}(graph)={"mean"=4457.822891144558, "mean"=4883.444172208611}
  out "Index":i32=150
  out "CH1  Bin Readings":dbl[](array[numeric])=[31.0, 45.0, 42.0, 59.0, 76.0, 121.0, 138.0, 195.0, 275.0, 326.0, 397.0, 435.0, 441.0, 437.0, 507.0, 498.0, 506.0, 492.0, 482.0, 446.0, 428.0, 369.0, 314.0, 325.0, 302.0, 249.0, 244.0, 250.0, 243.0, 254.0, 233.0, 221.0, 215.0, 235.0, 233.0, 189.0, 224.0, 176.0, 192.0, 161.0, 175.0, 185.0, 183.0, 152.0, 148.0, 162.0, 153.0, 165.0, 153.0, 140.0, 117.0, 137.0, 100.0, 112.0, 112.0, 114.0, 111.0, 101.0, 103.0, 103.0, 94.0, 91.0, 95.0, 90.0, 74.0, 67.0, 87.0, 75.0, 72.0, 68.0, 66.0, 72.0, 55.0, 64.0, 53.0, 63.0, 42.0, 50.0, 45.0, 55.0, 53.0, 51.0, 51.0, 44.0, 41.0, 41.0, 48.0, 38.0, 28.0, 34.0, 42.0, 23.0, 37.0, 33.0, 37.0, 40.0, 28.0, 30.0, 38.0, 25.0, 29.0, 35.0, 24.0, 26.0, 25.0, 22.0, 22.0, 22.0, 28.0, 34.0, 26.0, 21.0, 27.0, 21.0, 22.0, 20.0, 24.0, 25.0, 23.0, 19.0, 20.0, 29.0, 18.0, 25.0, 12.0, 30.0, 27.0, 14.0, 17.0, 30.0, 18.0, 22.0, 24.0, 14.0, 21.0, 20.0, 25.0, 21.0, 24.0, 24.0, 33.0, 21.0, 23.0, 21.0, 19.0, 25.0, 14.0, 17.0, 7.0, 17.0, 13.0, 20.0, 10.0, 14.0, 13.0, 22.0, 17.0, 24.0, 16.0, 20.0, 27.0, 14.0, 20.0, 16.0, 23.0, 22.0, 20.0, 16.0, 14.0, 19.0, 20.0, 14.0, 17.0, 18.0, 21.0, 8.0, 16.0, 12.0, 17.0, 17.0, 16.0, 24.0, 14.0, 15.0, 14.0, 17.0, 10.0, 19.0, 23.0, 25.0, 18.0, 19.0, 19.0, 21.0, 20.0, 16.0, 16.0, 17.0, 14.0, 14.0, 18.0, 13.0, 16.0, 10.0, 12.0, 15.0, 14.0, 18.0, 12.0, 15.0, 15.0, 12.0, 17.0, 11.0, 16.0, 18.0, 16.0, 16.0, 17.0, 19.0, 14.0, 14.0, 11.0, 13.0, 12.0, 19.0, 22.0, 10.0, 13.0, 20.0, 13.0, 21.0, 20.0, 14.0, 12.0, 25.0, 7.0, 12.0, 23.0, 13.0, 18.0, 20.0, 20.0, 16.0, 10.0, 17.0, 11.0, 10.0, 12.0, 16.0, 17.0, 15.0, 15.0, 14.0, 20.0, 11.0, 11.0, 13.0, 14.0, 15.0, 12.0, 16.0, 22.0, 24.0, 14.0, 21.0, 15.0, 27.0, 22.0, 24.0, 11.0, 17.0, 15.0, 14.0, 16.0, 10.0, 12.0, 19.0, 16.0, 14.0, 16.0, 14.0, 13.0, 18.0, 10.0, 18.0, 22.0, 13.0, 11.0, 12.0, 17.0, 12.0, 14.0, 7.0, 13.0, 18.0, 13.0, 12.0, 11.0, 19.0, 11.0, 18.0, 20.0, 15.0, 11.0, 25.0, 24.0, 18.0, 15.0, 21.0, 19.0, 19.0, 12.0, 14.0, 21.0, 22.0, 21.0, 15.0, 14.0, 18.0, 20.0, 11.0, 14.0, 15.0, 13.0, 16.0, 19.0, 16.0, 14.0, 21.0, 14.0, 18.0, 14.0, 16.0, 20.0, 18.0, 16.0, 17.0, 14.0, 15.0, 7.0, 15.0, 14.0, 14.0, 17.0, 18.0, 12.0, 19.0, 14.0, 15.0, 15.0, 12.0, 17.0, 12.0, 22.0, 15.0, 16.0, 14.0, 14.0, 12.0, 15.0, 16.0, 18.0, 15.0, 13.0, 19.0, 13.0, 10.0, 13.0, 19.0, 13.0, 19.0, 13.0, 21.0, 15.0, 17.0, 17.0, 16.0, 11.0, 22.0, 13.0, 13.0, 14.0, 18.0, 11.0, 13.0, 15.0, 21.0, 18.0, 12.0, 14.0, 16.0, 13.0, 19.0, 14.0, 14.0, 18.0, 21.0, 19.0, 15.0, 22.0, 20.0, 7.0, 15.0, 19.0, 26.0, 22.0, 15.0, 16.0, 13.0, 19.0, 13.0, 16.0, 15.0, 13.0, 15.0, 17.0, 12.0, 20.0, 18.0, 10.0, 16.0, 13.0, 23.0, 18.0, 18.0, 14.0, 18.0, 20.0, 13.0, 15.0, 18.0, 13.0, 13.0, 17.0, 13.0, 11.0, 23.0, 18.0, 17.0, 13.0, 24.0, 16.0, 15.0, 16.0, 18.0, 15.0, 14.0, 13.0, 16.0, 23.0, 22.0, 17.0, 12.0, 16.0, 17.0, 13.0, 12.0, 13.0, 21.0, 19.0, 10.0, 15.0, 16.0, 12.0, 15.0, 17.0, 16.0, 12.0, 14.0, 19.0, 15.0, 13.0, 17.0, 16.0, 20.0, 16.0, 18.0, 14.0, 23.0, 16.0, 12.0, 11.0, 19.0, 14.0, 18.0, 14.0, 16.0, 13.0, 14.0, 17.0, 11.0, 16.0, 10.0, 27.0, 13.0, 14.0, 8.0, 16.0, 20.0, 17.0, 19.0, 12.0, 27.0, 16.0, 18.0, 9.0, 13.0, 15.0, 16.0, 10.0, 14.0, 12.0, 11.0, 15.0, 19.0, 15.0, 10.0, 16.0, 23.0, 16.0, 22.0, 11.0, 22.0, 17.0, 24.0, 20.0, 13.0, 18.0, 19.0, 13.0, 11.0, 16.0, 18.0, 17.0, 19.0, 18.0, 11.0, 16.0, 19.0, 13.0, 10.0, 20.0, 17.0, 19.0, 19.0, 14.0, 18.0, 15.0, 15.0, 14.0, 18.0, 14.0, 14.0, 12.0, 15.0, 26.0, 12.0, 13.0, 0.0]
  out "CH1 (WV off) smooth":dbl[](array[numeric])=[24.746357615894034, 31.96490066225165, 45.743046357615896, 66.58410596026489, 98.65695364238408, 145.52450331125826, 206.78940397351, 281.6139072847683, 356.4682119205298, 423.7397350993376, 481.62715231788053, 523.9913907284765, 552.5807947019864, 573.4682119205296, 588.0443708609268, 593.3357615894038, 588.974834437086, 566.9019867549666, 527.1536423841056, 480.36556291390696, 435.23973509933757, 390.3887417218543, 350.8092715231788, 321.4913907284768, 296.37218543046356, 281.58079470198675, 274.5476821192053, 267.20331125827823, 260.0973509933776, 254.99470198675505, 250.50132450331137, 242.85562913907296, 234.91523178807955, 229.3887417218544, 223.36887417218549, 217.08410596026494, 210.00132450331128, 202.77947019867554, 196.54768211920532, 188.89536423841062, 180.7198675496689, 175.27615894039738, 169.22317880794705, 162.51788079470202, 157.23311258278147, 152.1966887417219, 149.49139072847686, 142.70993377483444, 136.59735099337746, 133.5211920529801, 128.2331125827814, 122.9947019867549, 118.9218543046357, 113.46490066225162, 109.15033112582779, 106.21324503311257, 100.6072847682119, 95.05430463576155, 91.85231788079467, 90.28278145695361, 86.27947019867548, 81.74304635761587, 77.45827814569536, 72.5841059602649, 68.59403973509936, 64.65364238410598, 61.67350993377487, 59.44172185430465, 56.81920529801325, 53.041059602649014, 49.968211920529804, 47.56092715231789, 45.31258278145697, 43.20662251655631, 40.358940397351006, 37.74966887417219, 35.36887417218543, 34.29602649006622, 33.567549668874165, 32.12715231788079, 30.196688741721854, 28.266225165562915, 26.481456953642383, 25.958278145695356, 25.64039735099337, 23.908609271523176, 22.223178807947015, 22.670198675496685, 22.6205298013245, 21.03774834437086, 21.064238410596026, 19.984768211920528, 19.557615894039735, 19.26953642384106, 17.908609271523176, 17.504635761589405, 17.130463576158945, 16.68013245033113, 16.415231788079474, 15.74966887417219, 15.819205298013252, 15.574172185430466, 14.19668874172185, 13.209933774834433, 12.279470198675494, 12.547682119205295, 12.935099337748342, 12.570860927152316, 12.057615894039731, 11.594039735099336, 11.103973509933773, 10.511258278145695, 10.319205298013244, 10.11390728476821, 9.895364238410593, 10.385430463576157, 10.471523178807946, 8.948344370860925, 8.395364238410593, 8.819205298013244, 8.160264900662249, 7.786092715231785, 8.027814569536421, 8.127152317880793, 8.401986754966886, 8.183443708609268, 7.613907284768208, 7.425165562913904, 7.123841059602645, 6.488079470198673, 6.252980132450329, 7.011258278145693, 6.286092715231785, 5.501324503311256, 5.696688741721852, 5.4019867549668845, 5.2728476821192025, 5.269536423841057, 5.501324503311256, 5.464900662251653, 5.3125827814569515, 4.819205298013243, 4.6105960264900645, 4.92185430463576, 4.766225165562911, 4.560927152317879, 4.769536423841057, 4.309271523178805, 4.007947019867546, 4.094039735099335, 4.2165562913907255, 4.365562913907282, 3.815894039735097, 3.630463576158939, 4.004635761589402, 4.050993377483441, 3.090728476821191, 2.4913907284768206, 2.951655629139072, 3.074172185430463, 3.117218543046356, 2.958278145695363, 2.9417218543046353, 2.911920529801324, 2.514569536423841, 2.7662251655629135, 2.8589403973509926, 2.5841059602649, 2.574172185430463, 2.4450331125827818, 2.2993377483443718, 2.474834437086093, 2.9417218543046353, 2.216556291390728, 1.6072847682119211, 2.1403973509933776, 1.898675496688742, 2.014569536423841, 2.2430463576158948, 1.9814569536423854, 1.4847682119205303, 1.9350993377483445, 2.7827814569536424, 2.2, 1.7331125827814575, 1.6536423841059609, 1.3754966887417228, 1.4450331125827822, 2.213245033112583, 2.1635761589403977, 1.6801324503311266, 1.9814569536423852, 1.842384105960266, 1.9516556291390734, 2.087417218543046, 1.7000000000000002, 1.5211920529801333, 1.3821192052980136, 1.1536423841059604, 0.8225165562913909, 0.9947019867549672, 1.1238410596026491, 1.2629139072847684, 1.700000000000001, 1.3324503311258287, 1.0245033112582782, 1.4251655629139077, 1.8721854304635772, 1.660264900662253, 1.5046357615894048, 2.027814569536424, 2.3125827814569533, 1.4549668874172188, 0.40860927152317905, 0.2960264900662251, 0.7132450331125832, 1.481456953642385, 1.4913907284768215, 1.1139072847682123, 0.9947019867549677, 1.3158940397351007, 1.6337748344370873, 1.0476821192052985, 0.8887417218543046, 1.0013245033112583, 1.5112582781456965, 1.9086092715231802, 1.6337748344370868, 0.8324503311258282, 0.8655629139072849, 1.2231788079470203, 0.7728476821192054, 0.8423841059602654, 0.779470198675497, 0.5741721854304633, 0.4417218543046356, 0.9086092715231793, 0.8953642384105966, 0.18675496688741727, 0.03443708609271508, 0.2662251655629138, 0.5741721854304638, 0.5907284768211924, 0.6536423841059606, 0.9052980132450335, 0.5079470198675499, 0.6735099337748346, 1.0940397350993383, 0.6403973509933777, 0.6370860927152321, 0.8655629139072853, 0.8523178807947025, 0.42516556291390756, 0.10397350993377483, 0.41854304635761613, 0.5807947019867551, 0.8158940397350996, 0.842384105960265, 0.41854304635761597, 0.6470198675496691, 0.7, 0.6933774834437085, 0.7000000000000001, 0.898675496688742, 0.8589403973509936, 0.4417218543046356, 0.6304635761589406, 0.8854304635761594, 0.8423841059602653, 0.6370860927152321, 0.2529801324503312, 0.031125827814569292, 0.5907284768211922, 0.8754966887417224, 0.885430463576159, 0.8357615894039736, 0.3655629139072849, 0.31589403973509933, 0.44172185430463584, 0.74635761589404, 0.7066225165562918, 0.20662251655629144, 0.7397350993377485, 0.8920529801324506, 0.48145695364238433, 0.7993377483443713, 0.6768211920529805, 0.13708609271523184, -0.32980132450331134, -0.27682119205298017, 0.24304635761589408, 0.03443708609271531, -0.14768211920529806, -0.03841059602649021, -0.03841059602649026, 0.2033112582781456, 0.309271523178808, 1.1039735099337749, 1.0344370860927152, 0.26953642384105947, -0.19072847682119196, -0.6046357615894038, 0.054304635761589615, 0.7033112582781462, 0.9052980132450337, 0.4847682119205299, 0.12052980132450315, 0.4880794701986756, 0.6403973509933777, 0.15364238410596032, 0.09072847682119216, 0.19337748344370867, 0.35894039735099326, 0.1668874172185429, -0.10132450331125835, 0.3258278145695363, 0.6900662251655632, 0.6470198675496692, 0.02119205298013252, 0.17682119205298022, 0.14039735099337738, 0.2728476821192054, 0.5476821192052983, -0.1443708609271523, -0.08807947019867557, 0.12715231788079462, 0.6668874172185433, 0.5642384105960268, -0.4125827814569536, 0.074172185430464, 0.3291390728476824, 0.16026490066225174, 0.4980132450331128, 0.07748344370860946, -0.3066225165562914, -0.4125827814569537, -0.03178807947019857, 0.5874172185430468, -0.06158940397350926, -0.3033112582781454, -0.07152317880794702, 0.11059602649006614, 0.3788079470198675, -0.12450331125827822, -0.16092715231788085, 0.07417218543046343, 0.011258278145695211, -0.24701986754966893, 0.12384105960264913, 0.5675496688741724, 0.352317880794702, 0.5973509933774837, 0.8225165562913913, 0.054304635761589726, -0.17086092715231796, 0.23642384105960262, -0.13774834437086095, 0.12715231788079484, 0.696688741721855, 0.4152317880794706, 0.5311258278145695, 0.7198675496688742, 0.31258278145695356, -0.018543046357615903, -0.04503311258278162, 0.06754966887417196, -0.14768211920529817, -0.30000000000000016, 0.49801324503311284, 0.802649006622517, 0.2927152317880798, 0.047682119205298176, -0.12450331125827815, 0.30927152317880796, 0.3225165562913908, -0.0019867549668875877, -0.06821192052980149, -0.1807947019867551, -0.03178807947019889, 0.044370860927152166, 0.2596026490066226, 0.418543046357616, 0.11721854304635757, -0.04503311258278153, 0.24304635761589402, 0.48807947019867554, 0.24635761589403976, 0.21324503311258275, 0.537748344370861, 0.4350993377483445, 0.04768211920529788, 0.13046357615894036, 0.37880794701986775, 0.4582781456953645, 0.28940397350993396, 0.13708609271523184, -0.28013245033112555, -0.8264900662251651, -0.11125827814569494, 0.7066225165562917, 0.537748344370861, 0.38543046357615907, 0.18344370860927153, 0.21655629139072885, 0.26622516556291426, -0.025165562913907372, -0.02516556291390732, 0.3357615894039735, 0.7596026490066229, 0.22317880794702022, 0.21655629139072885, 0.739735099337749, 0.39867549668874175, -0.23708609271523184, -0.46225165562913906, 0.09072847682119187, 0.6834437086092718, 0.6768211920529806, 0.5178807947019869, 0.4317880794701987, 0.08741721854304627, -0.06158940397351008, 0.05761589403973517, 0.07086092715231793, 0.5311258278145695, 0.2364238410596029, -0.26357615894039715, 0.037748344370860776, -0.001986754966887456, 0.25960264900662294, 0.11390728476821227, -0.03509933774834445, 0.24304635761589377, -0.05496688741721874, 0.2066225165562914, 0.276158940397351, 0.027814569536423667, 0.08741721854304621, 0.4317880794701989, 0.4715231788079472, -0.452317880794702, -0.6807947019867546, 0.06423841059602706, 0.3589403973509936, 0.2562913907284767, -0.10794701986754984, 0.11059602649006617, 0.4913907284768213, -0.2105960264900659, -0.6907284768211917, -0.35960264900662237, 0.07417218543046347, 0.24304635761589388, 0.7860927152317884, 0.17019867549668932, -0.7271523178807944, -0.37947019867549653, -0.09470198675496692, 0.16357615894039734, 0.3490066225165564, 0.04768211920529808, 0.12052980132450308, -0.03509933774834445, -0.3231788079470197, 0.05099337748344368, 0.16026490066225155, -0.10132450331125842, -0.3827814569536425, -0.42251655629139084, -0.45562913907284763, 0.07086092715231812, 0.299337748344371, -0.22052980132450323, -0.5748344370860923, -0.4125827814569534, 0.05430463576158931, 0.252980132450331, 0.13046357615894022, 0.24304635761589377, 0.11390728476821171, 0.5543046357615896, 0.7430463576158942, 0.1006622516556289, 0.03443708609271501, 0.19006622516556276, 0.11721854304635754, -0.30993377483443707, -0.22384105960264888, 0.0741721854304636, 0.23311258278145708, 0.31920529801324526, 0.2596026490066224, 0.11059602649006606, 0.133774834437086, 0.01456953642384104, 0.28940397350993396, 0.20662251655629177, -0.20728476821192043, 0.18344370860927164, -0.04503311258278106, -0.21390728476821164, 0.46158940397351006, 0.5476821192052981, 0.09735099337748364, 0.027814569536423903, 0.514569536423841, 0.3688741721854304, 0.2496688741721855, 0.5576158940397353, 0.3291390728476823, 0.7066225165562917, 1.064238410596027, 0.5576158940397353, 0.3324503311258278, 0.5178807947019868, 0.1437086092715232, -0.17748344370860938, 0.2231788079470198, 0.4317880794701986, 0.570860927152318, 0.46158940397351, -0.36291390728476824, -0.43245033112582776, -0.05827814569536427, 0.07086092715231788, 0.395364238410596, 0.5576158940397352, 0.38543046357615907, 0.13377483443708593, 0.1834437086092714, -0.07483443708609264, 0.10066225165562945, 0.44834437086092727, 0.31258278145695356, 0.45827814569536435, 0.1801324503311258, -0.06821192052980155, 0.1039735099337749, -0.26357615894039704, -0.5947019867549669, -0.051655629139073095, 0.30596026490066214, 0.4847682119205298, 0.4947019867549669, -0.0019867549668875356, -0.22052980132450334, 0.05099337748344357, -0.25033112582781425, -0.29006622516556246, 0.25298013245033113, 0.16026490066225163, 0.05430463576158934, -0.06158940397351009, 0.30927152317880824, 0.517880794701987, 0.16357615894039723, -0.36291390728476813, -0.9589403973509931]
  out "CH0 (WV on) smoothed":dbl[](array[numeric])=[23.31854304635761, 29.414569536423848, 40.345033112582804, 57.85165562913907, 83.2754966887417, 117.87483443708612, 164.97748344370865, 216.80860927152315, 265.24238410596, 309.9211920529798, 343.5602649006619, 363.3317880794699, 374.4807947019865, 377.5139072847679, 375.3350993377481, 369.2225165562911, 356.6298013245031, 335.42781456953617, 306.4377483443705, 271.0900662251653, 236.04039735099332, 205.8748344370861, 179.4443708609272, 159.8682119205299, 146.41788079470206, 137.88145695364244, 133.61324503311266, 129.65629139072854, 125.73907284768218, 121.66953642384111, 117.42781456953644, 113.47086092715227, 108.43112582781453, 103.0933774834437, 100.01059602649008, 95.7158940397351, 91.25231788079469, 87.88807947019866, 82.63311258278142, 79.82847682119203, 76.93774834437083, 72.43774834437083, 69.2026490066225, 66.57682119205296, 63.08013245033112, 60.22913907284768, 58.003973509933786, 56.3152317880795, 54.215894039735126, 51.28543046357618, 49.14966887417221, 46.91456953642387, 46.42781456953645, 44.871523178807976, 41.98741721854308, 39.86158940397354, 38.65629139072851, 38.20927152317884, 37.21589403973513, 35.298675496688766, 32.55033112582783, 30.861589403973525, 29.6430463576159, 27.35496688741722, 25.659602649006622, 24.93774834437086, 22.626490066225166, 21.07682119205298, 20.41788079470198, 19.19271523178807, 18.020529801324496, 16.58675496688741, 15.702649006622508, 15.586754966887412, 14.977483443708607, 13.487417218543044, 12.676158940397347, 12.093377483443707, 11.609933774834435, 11.15960264900662, 10.34503311258278, 9.20596026490066, 8.87483443708609, 8.798675496688741, 7.77549668874172, 7.265562913907284, 7.957615894039736, 8.341721854304634, 7.997350993377481, 7.348344370860925, 6.590066225165562, 6.2523178807947, 6.090066225165561, 5.898013245033111, 6.457615894039735, 6.712582781456954, 6.258940397350992, 6.278807947019866, 6.18278145695364, 5.944370860927149, 5.841721854304634, 5.911258278145693, 5.513907284768209, 4.960927152317879, 4.169536423841059, 3.735761589403973, 4.3284768211920515, 4.785430463576158, 3.9741721854304632, 3.6264900662251645, 3.907947019867549, 2.9211920529801323, 2.9311258278145687, 3.6927152317880783, 3.1960264900662256, 2.9377483443708607, 3.209271523178807, 3.146357615894039, 2.6165562913907277, 2.742384105960265, 2.9874172185430456, 2.378145695364238, 1.8615894039735108, 2.0834437086092716, 2.5701986754966883, 2.4311258278145695, 1.9807947019867553, 2.053642384105961, 2.2523178807947017, 2.1860927152317884, 1.755629139072849, 1.4311258278145707, 1.4013245033112594, 1.5337748344370874, 1.9543046357615899, 2.047019867549669, 1.66953642384106, 1.7887417218543045, 2.2788079470198674, 1.762251655629139, 1.9741721854304632, 1.9410596026490068, 1.3384105960264912, 2.0304635761589407, 2.14635761589404, 1.298675496688742, 1.0635761589403976, 0.9609271523178811, 1.3880794701986763, 1.8450331125827826, 1.2192052980132457, 1.0139072847682125, 0.7754966887417221, 0.7026490066225168, 0.7390728476821196, 1.0403973509933782, 1.205960264900663, 0.8549668874172189, 1.1993377483443717, 0.997350993377484, 0.9543046357615901, 0.6860927152317887, 0.8814569536423843, 1.219205298013245, 0.4973509933774831, 0.5933774834437083, 1.003973509933775, 1.414569536423842, 0.8516556291390733, 0.7655629139072848, 0.9973509933774833, 0.4046357615894038, 0.6430463576158941, 1.0569536423841066, 1.1198675496688744, 0.5271523178807943, 0.22582781456953638, 1.139735099337749, 0.944370860927153, 0.14304635761589404, 0.3251655629139073, 0.30529801324503325, 0.219205298013245, 0.4509933774834438, 0.3715231788079472, 0.3450331125827815, 0.9112582781456962, 1.020529801324504, 0.8251655629139072, 1.3251655629139072, 0.6099337748344371, -0.5589403973509934, -0.24105960264900683, -0.1251655629139074, 0.14966887417218536, 0.6993377483443706, 0.6099337748344369, 0.2788079470198674, 0.04370860927152306, 0.6529801324503315, 1.3947019867549675, 0.7390728476821197, -0.062251655629138924, 0.2357615894039736, 0.6662251655629134, 0.7490066225165559, 0.6132450331125827, 0.3317880794701987, 0.17284768211920534, 0.29536423841059595, 0.14635761589403978, -0.04900662251655616, 0.6596026490066227, 0.81523178807947, 0.391390728476821, 0.9311258278145702, 1.1960264900662256, 0.7589403973509932, -0.1317880794701986, -0.3900662251655629, 0.31192052980132445, 0.3052980132450332, 0.32516556291390725, 0.10993377483443695, -0.05231788079470212, 0.6629139072847687, 0.4079470198675502, 0.1993377483443707, 0.40463576158940373, 0.19602649006622497, 0.5072847682119204, 0.8052980132450329, 0.6298013245033113, 0.7390728476821197, 0.5569536423841065, 0.12980132450331125, 0.19602649006622513, 0.4642384105960265, 0.7357615894039738, 0.6860927152317886, 0.7225165562913913, 0.29867549668874205, -0.19801324503311243, 0.5668874172185437, 1.0768211920529804, 0.5933774834437084, 0.5105960264900663, 0.5735099337748344, 0.6562913907284772, 0.7192052980132457, -0.08211920529801325, -0.10860927152317884, 0.6430463576158938, 0.6728476821192048, 0.15629139072847656, -0.1384105960264901, 0.4079470198675496, 0.6728476821192051, 0.5172185430463575, 0.3086092715231789, -0.15165562913907266, -0.15827814569536422, 0.42450331125827806, 0.8251655629139073, 0.7655629139072849, 0.41456953642384126, 0.18278145695364256, 0.2953642384105961, 0.3019867549668874, 0.14635761589403967, -0.23112582781456975, -0.0854304635761591, 0.5172185430463575, 0.5304635761589402, 0.1066225165562914, 0.4046357615894039, 0.8483443708609271, 0.6562913907284769, 0.4377483443708611, 0.09006622516556306, 0.4476821192052981, 0.8748344370860927, 0.1430463576158939, -0.40993377483443705, -0.029139072847681996, 0.05695364238410601, -0.3569536423841059, 0.1695364238410602, 0.43443708609271564, -0.4364238410596028, -0.5059602649006623, 0.03708609271523182, 0.11986754966887414, 0.3152317880794701, 0.23907284768211914, 0.043708609271523285, -0.09205298013245033, 0.305298013245033, 0.7986754966887417, 0.4410596026490065, -0.19470198675496708, -0.23774834437086104, 0.4046357615894042, 0.20264900662251684, 0.44105960264900734, 0.792052980132451, 0.1761589403973508, -0.23443708609271524, -0.34701986754966874, 0.20927152317880784, 0.5006622516556292, 0.32185430463576165, 0.15629139072847678, -0.012582781456953726, 0.22913907284768203, -0.015894039735099397, -0.3271523178807948, -0.01258278145695349, 0.03377483443708629, -0.26092715231788094, -0.49271523178807963, -0.6516556291390729, -0.20794701986754965, 0.6066225165562922, 0.401324503311259, -0.6483443708609267, -0.7509933774834434, -0.36357615894039746, -0.23443708609271524, 0.07019867549668873, -0.12847682119205306, 0.013907284768211792, 0.5304635761589402, 0.02384105960264865, 0.05033112582781424, 0.7688741721854304, 0.2986754966887418, -0.5821192052980133, -0.2708609271523179, 0.43443708609271536, 0.11324503311258294, -0.2245033112582781, 0.020529801324503365, -0.2410596026490066, -0.31059602649006623, 0.1430463576158939, 0.6397350993377482, 0.4576158940397351, -0.05894039735099339, 0.15960264900662263, 0.15298013245033112, -0.4463576158940398, -0.949668874172185, -0.3999999999999996, -0.01920529801324497, -0.1715231788079469, -0.1781456953642383, -0.2112582781456954, 0.040397350993377365, -0.01920529801324508, -0.10198675496688739, -0.03576158940397327, 0.05695364238410616, -0.2973509933774831, -0.5953642384105957, -0.33046357615894045, 0.3119205298013245, 0.7556291390728476, 0.3450331125827813, 0.09006622516556279, -0.09205298013245052, 0.05364238410596023, 0.5735099337748351, 0.30198675496688804, -0.1880794701986755, -0.35364238410596044, -0.15496688741721873, -0.04569536423841054, 0.3615894039735099, 0.8317880794701986, 0.13973509933774847, -0.5490066225165564, -0.16490066225165587, -0.27086092715231735, -0.1748344370860922, 0.5933774834437084, 0.18609271523178803, -0.025827814569536395, 0.0569536423841059, 0.18940397350993365, 0.9973509933774839, 0.8715231788079476, 0.2589403973509935, 0.15960264900662247, 0.030463576158940266, -0.04569536423841061, 0.07682119205298012, 0.25894039735099333, 0.35827814569536426, 0.5139072847682119, 0.14966887417218552, -0.16490066225165548, 0.003973509933774877, -0.3536423841059604, -0.5688741721854305, -0.5721854304635763, -0.17152317880794718, 0.381456953642384, 0.18940397350993368, 0.09006622516556285, -0.2377483443708609, -0.333774834437086, 0.04701986754966901, 0.13973509933774841, 0.30529801324503303, 0.6463576158940396, 0.5370860927152318, -0.1417218543046358, 0.02715231788079464, 0.18940397350993388, 0.07682119205298017, 0.050331125827814543, 0.06688741721854308, 0.1165562913907285, -0.23112582781456942, -0.12516556291390726, 0.2456953642384105, 0.020529801324503494, -0.2907284768211918, 0.28211920529801315, 0.34503311258278146, 0.2390728476821197, 0.6629139072847685, 0.818543046357616, 0.6364238410596026, 0.25894039735099345, 0.2490066225165564, -0.06887417218543049, -0.44304635761589395, -0.5556291390728478, -0.10529801324503335, 0.17947019867549663, 0.22251655629139078, -0.19801324503311268, -0.28410596026490087, 0.5602649006622515, -0.05894039735099338, -0.5490066225165563, -0.6715231788079465, -0.47615894039735046, -0.21456953642384116, -0.701324503311258, -0.698013245033112, -0.3039735099337748, 0.1132450331125827, 0.20596026490066224, 0.07682119205298014, -0.14172185430463596, -0.0655629139072849, -0.05894039735099328, -0.19139072847682115, 0.19933774834437076, 0.6529801324503309, 0.21920529801324487, -0.17814569536423858, 0.007284768211920485, -0.31059602649006607, -0.32715231788079463, -0.11523178807947038, -0.2543046357615895, 0.027152317880794585, 0.17947019867549652, 0.143046357615894, 0.2192052980132449, 0.38145695364238397, 0.7688741721854305, 0.5933774834437087, -0.06887417218543054, 0.1993377483443709, 0.5403973509933775, 0.22913907284768215, 0.003973509933774794, -0.0059602649006621905, 0.39801324503311275, 0.20927152317880793, -0.042384105960264915, 0.176158940397351, 0.30529801324503314, -0.0622516556291392, -0.0920529801324506, 0.02384105960264883, 0.11324503311258285, 0.4576158940397351, 0.02715231788079453, -0.015894039735099424, 0.007284768211920645, -0.14503311258278112, 0.017218543046357674, -0.1516556291390729, -0.2509933774834436, -0.09205298013245042, -0.13841059602649028, -0.08211920529801324, -0.1119205298013244, -0.1748344370860927, 0.31523178807947017, 0.457615894039735, 0.10662251655629117, -0.3238410596026491, -0.19139072847682115, 0.11324503311258272, 0.07682119205298017, -0.2145695364238409, -0.5754966887417218, -0.2841059602649007, 0.1298013245033112, 0.4675496688741721, 0.457615894039735, 0.18609271523178808, -0.32052980132450337, -0.3569536423841061, -0.27748344370860933, -0.10198675496688742, 0.3052980132450332, -0.062251655629139035, 0.053642384105960186, 0.13973509933774828, 0.44437086092715244, 0.38476821192052996, -0.09205298013245027, -0.22119205298013245, 0.2026490066225168, 0.29867549668874205, -0.07880794701986754, 0.18609271523178803, 0.16622516556291383, 0.28543046357615887, 0.5271523178807946, -0.03245033112582796, -0.6350993377483446, -0.43311258278145714, 0.10331125827814565, 0.12317880794701987, -0.09867549668874176, 0.5105960264900666, 0.41125827814569565, 0.3052980132450328, 0.23576158940397332, -0.5589403973509935, -0.9066225165562909, -0.4066225165562909, -0.07549668874172194, 0.09668874172185424, 0.49735099337748345, 0.1264900662251656, 0.0569536423841059, 0.010596026490066274, -0.32384105960264886]
  out "CH 0 Bin Readings":dbl[](array[numeric])=[35.0, 39.0, 34.0, 41.0, 59.0, 77.0, 113.0, 130.0, 203.0, 227.0, 262.0, 250.0, 226.0, 281.0, 293.0, 253.0, 270.0, 261.0, 239.0, 208.0, 201.0, 171.0, 140.0, 135.0, 130.0, 143.0, 125.0, 122.0, 127.0, 104.0, 120.0, 96.0, 102.0, 110.0, 94.0, 78.0, 94.0, 64.0, 83.0, 70.0, 77.0, 75.0, 62.0, 56.0, 71.0, 62.0, 71.0, 60.0, 76.0, 53.0, 40.0, 63.0, 39.0, 44.0, 45.0, 45.0, 52.0, 61.0, 43.0, 46.0, 46.0, 31.0, 33.0, 29.0, 34.0, 31.0, 33.0, 39.0, 28.0, 37.0, 26.0, 22.0, 35.0, 36.0, 30.0, 27.0, 24.0, 26.0, 31.0, 24.0, 29.0, 25.0, 39.0, 26.0, 18.0, 20.0, 31.0, 25.0, 32.0, 15.0, 18.0, 19.0, 20.0, 24.0, 16.0, 15.0, 18.0, 15.0, 22.0, 22.0, 11.0, 27.0, 18.0, 15.0, 22.0, 17.0, 19.0, 18.0, 21.0, 16.0, 20.0, 12.0, 13.0, 21.0, 11.0, 16.0, 23.0, 19.0, 17.0, 28.0, 14.0, 12.0, 9.0, 17.0, 19.0, 14.0, 18.0, 14.0, 16.0, 15.0, 15.0, 21.0, 15.0, 11.0, 16.0, 14.0, 12.0, 13.0, 18.0, 22.0, 22.0, 15.0, 9.0, 19.0, 12.0, 11.0, 17.0, 15.0, 14.0, 18.0, 15.0, 12.0, 16.0, 20.0, 15.0, 13.0, 15.0, 18.0, 13.0, 14.0, 12.0, 14.0, 15.0, 19.0, 15.0, 12.0, 14.0, 24.0, 17.0, 11.0, 12.0, 19.0, 15.0, 15.0, 15.0, 14.0, 12.0, 15.0, 18.0, 12.0, 13.0, 16.0, 16.0, 21.0, 17.0, 9.0, 24.0, 16.0, 13.0, 9.0, 12.0, 19.0, 10.0, 14.0, 17.0, 23.0, 13.0, 15.0, 13.0, 19.0, 17.0, 20.0, 19.0, 8.0, 19.0, 14.0, 16.0, 11.0, 25.0, 20.0, 17.0, 12.0, 13.0, 18.0, 22.0, 6.0, 14.0, 20.0, 12.0, 15.0, 12.0, 13.0, 11.0, 17.0, 10.0, 13.0, 15.0, 17.0, 17.0, 13.0, 22.0, 16.0, 4.0, 23.0, 13.0, 12.0, 12.0, 8.0, 13.0, 21.0, 25.0, 17.0, 17.0, 21.0, 11.0, 16.0, 9.0, 12.0, 13.0, 13.0, 12.0, 12.0, 16.0, 16.0, 14.0, 19.0, 14.0, 22.0, 13.0, 10.0, 14.0, 15.0, 13.0, 21.0, 15.0, 11.0, 16.0, 19.0, 15.0, 14.0, 20.0, 15.0, 23.0, 13.0, 17.0, 12.0, 8.0, 23.0, 13.0, 16.0, 15.0, 11.0, 13.0, 8.0, 23.0, 19.0, 14.0, 17.0, 17.0, 9.0, 13.0, 15.0, 14.0, 13.0, 19.0, 11.0, 12.0, 14.0, 18.0, 15.0, 11.0, 16.0, 24.0, 12.0, 23.0, 13.0, 12.0, 17.0, 20.0, 14.0, 13.0, 13.0, 16.0, 15.0, 21.0, 12.0, 13.0, 11.0, 20.0, 19.0, 12.0, 15.0, 13.0, 12.0, 17.0, 15.0, 18.0, 12.0, 18.0, 13.0, 26.0, 17.0, 16.0, 12.0, 16.0, 16.0, 16.0, 18.0, 10.0, 18.0, 18.0, 14.0, 6.0, 15.0, 11.0, 13.0, 21.0, 12.0, 9.0, 23.0, 19.0, 13.0, 7.0, 17.0, 19.0, 13.0, 15.0, 11.0, 17.0, 19.0, 11.0, 20.0, 11.0, 20.0, 18.0, 16.0, 20.0, 20.0, 20.0, 20.0, 18.0, 7.0, 13.0, 12.0, 15.0, 15.0, 16.0, 7.0, 15.0, 9.0, 17.0, 16.0, 13.0, 14.0, 10.0, 20.0, 15.0, 17.0, 11.0, 22.0, 15.0, 14.0, 13.0, 11.0, 7.0, 15.0, 13.0, 16.0, 11.0, 18.0, 17.0, 14.0, 15.0, 11.0, 10.0, 17.0, 11.0, 15.0, 17.0, 16.0, 16.0, 18.0, 21.0, 13.0, 18.0, 15.0, 12.0, 21.0, 16.0, 16.0, 14.0, 17.0, 14.0, 13.0, 13.0, 18.0, 9.0, 15.0, 16.0, 8.0, 18.0, 12.0, 9.0, 9.0, 16.0, 17.0, 16.0, 17.0, 11.0, 7.0, 15.0, 22.0, 11.0, 19.0, 11.0, 15.0, 16.0, 13.0, 11.0, 18.0, 18.0, 18.0, 23.0, 16.0, 12.0, 17.0, 10.0, 12.0, 21.0, 10.0, 12.0, 11.0, 12.0, 18.0, 9.0, 21.0, 19.0, 15.0, 13.0, 10.0, 11.0, 12.0, 14.0, 23.0, 13.0, 12.0, 12.0, 17.0, 13.0, 17.0, 20.0, 22.0, 12.0, 18.0, 12.0, 18.0, 19.0, 7.0, 23.0, 14.0, 18.0, 13.0, 15.0, 26.0, 14.0, 15.0, 21.0, 13.0, 17.0, 14.0, 13.0, 14.0, 14.0, 18.0, 23.0, 25.0, 15.0, 15.0, 21.0, 10.0, 21.0, 12.0, 14.0, 12.0, 22.0, 17.0, 10.0, 14.0, 13.0, 12.0, 10.0, 20.0, 14.0, 19.0, 14.0, 10.0, 18.0, 19.0, 23.0, 18.0, 15.0, 12.0, 16.0, 14.0, 13.0, 11.0, 16.0, 13.0, 9.0, 19.0, 13.0, 21.0, 18.0, 17.0, 12.0, 8.0, 20.0, 13.0, 11.0, 8.0, 16.0, 13.0, 15.0, 16.0, 15.0, 6.0, 19.0, 14.0, 23.0, 0.0]
  out "Range Corrected Altitude Array":dbl[](array[numeric])=[1406.25, 5625.0, 12656.25, 22500.0, 35156.25, 50625.0, 68906.25, 90000.0, 113906.25, 140625.0, 170156.25, 202500.0, 237656.25, 275625.0, 316406.25, 360000.0, 406406.25, 455625.0, 507656.25, 562500.0, 620156.25, 680625.0, 743906.25, 810000.0, 878906.25, 950625.0, 1025156.25, 1102500.0, 1182656.25, 1265625.0, 1351406.25, 1440000.0, 1531406.25, 1625625.0, 1722656.25, 1822500.0, 1925156.25, 2030625.0, 2138906.25, 2250000.0, 2363906.25, 2480625.0, 2600156.25, 2722500.0, 2847656.25, 2975625.0, 3106406.25, 3240000.0, 3376406.25, 3515625.0, 3657656.25, 3802500.0, 3950156.25, 4100625.0, 4253906.25, 4410000.0, 4568906.25, 4730625.0, 4895156.25, 5062500.0, 5232656.25, 5405625.0, 5581406.25, 5760000.0, 5941406.25, 6125625.0, 6312656.25, 6502500.0, 6695156.25, 6890625.0, 7088906.25, 7290000.0, 7493906.25, 7700625.0, 7910156.25, 8122500.0, 8337656.25, 8555625.0, 8776406.25, 9000000.0, 9226406.25, 9455625.0, 9687656.25, 9922500.0, 10160156.25, 10400625.0, 10643906.25, 10890000.0, 11138906.25, 11390625.0, 11645156.25, 11902500.0, 12162656.25, 12425625.0, 12691406.25, 12960000.0, 13231406.25, 13505625.0, 13782656.25, 14062500.0, 14345156.25, 14630625.0, 14918906.25, 15210000.0, 15503906.25, 15800625.0, 16100156.25, 16402500.0, 16707656.25, 17015625.0, 17326406.25, 17640000.0, 17956406.25, 18275625.0, 18597656.25, 18922500.0, 19250156.25, 19580625.0, 19913906.25, 20250000.0, 20588906.25, 20930625.0, 21275156.25, 21622500.0, 21972656.25, 22325625.0, 22681406.25, 23040000.0, 23401406.25, 23765625.0, 24132656.25, 24502500.0, 24875156.25, 25250625.0, 25628906.25, 26010000.0, 26393906.25, 26780625.0, 27170156.25, 27562500.0, 27957656.25, 28355625.0, 28756406.25, 29160000.0, 29566406.25, 29975625.0, 30387656.25, 30802500.0, 31220156.25, 31640625.0, 32063906.25, 32490000.0, 32918906.25, 33350625.0, 33785156.25, 34222500.0, 34662656.25, 35105625.0, 35551406.25, 36000000.0, 36451406.25, 36905625.0, 37362656.25, 37822500.0, 38285156.25, 38750625.0, 39218906.25, 39690000.0, 40163906.25, 40640625.0, 41120156.25, 41602500.0, 42087656.25, 42575625.0, 43066406.25, 43560000.0, 44056406.25, 44555625.0, 45057656.25, 45562500.0, 46070156.25, 46580625.0, 47093906.25, 47610000.0, 48128906.25, 48650625.0, 49175156.25, 49702500.0, 50232656.25, 50765625.0, 51301406.25, 51840000.0, 52381406.25, 52925625.0, 53472656.25, 54022500.0, 54575156.25, 55130625.0, 55688906.25, 56250000.0, 56813906.25, 57380625.0, 57950156.25, 58522500.0, 59097656.25, 59675625.0, 60256406.25, 60840000.0, 61426406.25, 62015625.0, 62607656.25, 63202500.0, 63800156.25, 64400625.0, 65003906.25, 65610000.0, 66218906.25, 66830625.0, 67445156.25, 68062500.0, 68682656.25, 69305625.0, 69931406.25, 70560000.0, 71191406.25, 71825625.0, 72462656.25, 73102500.0, 73745156.25, 74390625.0, 75038906.25, 75690000.0, 76343906.25, 77000625.0, 77660156.25, 78322500.0, 78987656.25, 79655625.0, 80326406.25, 81000000.0, 81676406.25, 82355625.0, 83037656.25, 83722500.0, 84410156.25, 85100625.0, 85793906.25, 86490000.0, 87188906.25, 87890625.0, 88595156.25, 89302500.0, 90012656.25, 90725625.0, 91441406.25, 92160000.0, 92881406.25, 93605625.0, 94332656.25, 95062500.0, 95795156.25, 96530625.0, 97268906.25, 98010000.0, 98753906.25, 99500625.0, 100250156.25, 101002500.0, 101757656.25, 102515625.0, 103276406.25, 104040000.0, 104806406.25, 105575625.0, 106347656.25, 107122500.0, 107900156.25, 108680625.0, 109463906.25, 110250000.0, 111038906.25, 111830625.0, 112625156.25, 113422500.0, 114222656.25, 115025625.0, 115831406.25, 116640000.0, 117451406.25, 118265625.0, 119082656.25, 119902500.0, 120725156.25, 121550625.0, 122378906.25, 123210000.0, 124043906.25, 124880625.0, 125720156.25, 126562500.0, 127407656.25, 128255625.0, 129106406.25, 129960000.0, 130816406.25, 131675625.0, 132537656.25, 133402500.0, 134270156.25, 135140625.0, 136013906.25, 136890000.0, 137768906.25, 138650625.0, 139535156.25, 140422500.0, 141312656.25, 142205625.0, 143101406.25, 144000000.0, 144901406.25, 145805625.0, 146712656.25, 147622500.0, 148535156.25, 149450625.0, 150368906.25, 151290000.0, 152213906.25, 153140625.0, 154070156.25, 155002500.0, 155937656.25, 156875625.0, 157816406.25, 158760000.0, 159706406.25, 160655625.0, 161607656.25, 162562500.0, 163520156.25, 164480625.0, 165443906.25, 166410000.0, 167378906.25, 168350625.0, 169325156.25, 170302500.0, 171282656.25, 172265625.0, 173251406.25, 174240000.0, 175231406.25, 176225625.0, 177222656.25, 178222500.0, 179225156.25, 180230625.0, 181238906.25, 182250000.0, 183263906.25, 184280625.0, 185300156.25, 186322500.0, 187347656.25, 188375625.0, 189406406.25, 190440000.0, 191476406.25, 192515625.0, 193557656.25, 194602500.0, 195650156.25, 196700625.0, 197753906.25, 198810000.0, 199868906.25, 200930625.0, 201995156.25, 203062500.0, 204132656.25, 205205625.0, 206281406.25, 207360000.0, 208441406.25, 209525625.0, 210612656.25, 211702500.0, 212795156.25, 213890625.0, 214988906.25, 216090000.0, 217193906.25, 218300625.0, 219410156.25, 220522500.0, 221637656.25, 222755625.0, 223876406.25, 225000000.0, 226126406.25, 227255625.0, 228387656.25, 229522500.0, 230660156.25, 231800625.0, 232943906.25, 234090000.0, 235238906.25, 236390625.0, 237545156.25, 238702500.0, 239862656.25, 241025625.0, 242191406.25, 243360000.0, 244531406.25, 245705625.0, 246882656.25, 248062500.0, 249245156.25, 250430625.0, 251618906.25, 252810000.0, 254003906.25, 255200625.0, 256400156.25, 257602500.0, 258807656.25, 260015625.0, 261226406.25, 262440000.0, 263656406.25, 264875625.0, 266097656.25, 267322500.0, 268550156.25, 269780625.0, 271013906.25, 272250000.0, 273488906.25, 274730625.0, 275975156.25, 277222500.0, 278472656.25, 279725625.0, 280981406.25, 282240000.0, 283501406.25, 284765625.0, 286032656.25, 287302500.0, 288575156.25, 289850625.0, 291128906.25, 292410000.0, 293693906.25, 294980625.0, 296270156.25, 297562500.0, 298857656.25, 300155625.0, 301456406.25, 302760000.0, 304066406.25, 305375625.0, 306687656.25, 308002500.0, 309320156.25, 310640625.0, 311963906.25, 313290000.0, 314618906.25, 315950625.0, 317285156.25, 318622500.0, 319962656.25, 321305625.0, 322651406.25, 324000000.0, 325351406.25, 326705625.0, 328062656.25, 329422500.0, 330785156.25, 332150625.0, 333518906.25, 334890000.0, 336263906.25, 337640625.0, 339020156.25, 340402500.0, 341787656.25, 343175625.0, 344566406.25, 345960000.0, 347356406.25, 348755625.0, 350157656.25, 351562500.0, 352970156.25, 354380625.0, 355793906.25, 357210000.0, 358628906.25, 360050625.0, 361475156.25, 362902500.0, 364332656.25, 365765625.0, 367201406.25, 368640000.0, 370081406.25, 371525625.0, 372972656.25, 374422500.0, 375875156.25, 377330625.0, 378788906.25, 380250000.0, 381713906.25, 383180625.0, 384650156.25, 386122500.0, 387597656.25, 389075625.0, 390556406.25, 392040000.0, 393526406.25, 395015625.0, 396507656.25, 398002500.0, 399500156.25, 401000625.0, 402503906.25, 404010000.0, 405518906.25, 407030625.0, 408545156.25, 410062500.0, 411582656.25, 413105625.0, 414631406.25, 416160000.0, 417691406.25, 419225625.0, 420762656.25, 422302500.0, 423845156.25, 425390625.0, 426938906.25, 428490000.0, 430043906.25, 431600625.0, 433160156.25, 434722500.0, 436287656.25, 437855625.0, 439426406.25, 441000000.0]
  out "Altitude Array (km)":dbl[](array[numeric])=[0.0375, 0.075, 0.11249999999999999, 0.15, 0.1875, 0.225, 0.26249999999999996, 0.3, 0.33749999999999997, 0.37499999999999994, 0.4125, 0.44999999999999996, 0.48749999999999993, 0.525, 0.5625, 0.6, 0.6375, 0.6749999999999999, 0.7124999999999999, 0.75, 0.7875, 0.825, 0.8624999999999999, 0.8999999999999999, 0.9374999999999999, 0.975, 1.0125, 1.05, 1.0875000000000001, 1.125, 1.1625, 1.2, 1.2375, 1.2750000000000001, 1.3125, 1.35, 1.3875, 1.425, 1.4625000000000001, 1.5, 1.5375, 1.575, 1.6125, 1.6500000000000001, 1.6875, 1.725, 1.7625, 1.8, 1.8375, 1.875, 1.9125, 1.95, 1.9875, 2.025, 2.0625, 2.1, 2.1375, 2.175, 2.2125, 2.25, 2.2875, 2.325, 2.3625, 2.4, 2.4375, 2.475, 2.5125, 2.55, 2.5875, 2.625, 2.6625, 2.7, 2.7375, 2.775, 2.8125, 2.85, 2.8875, 2.925, 2.9625, 3.0, 3.0375, 3.075, 3.1125, 3.15, 3.1875, 3.225, 3.2625, 3.3, 3.3375, 3.375, 3.4125, 3.45, 3.4875, 3.525, 3.5625, 3.6, 3.6374999999999997, 3.675, 3.7125, 3.75, 3.7875, 3.8249999999999997, 3.8625, 3.9, 3.9375, 3.975, 4.012499999999999, 4.05, 4.0874999999999995, 4.124999999999999, 4.1625, 4.199999999999999, 4.2375, 4.2749999999999995, 4.312499999999999, 4.35, 4.387499999999999, 4.425, 4.4624999999999995, 4.499999999999999, 4.5375, 4.574999999999999, 4.6125, 4.6499999999999995, 4.687499999999999, 4.725, 4.762499999999999, 4.8, 4.8374999999999995, 4.874999999999999, 4.9125, 4.949999999999999, 4.9875, 5.0249999999999995, 5.062499999999999, 5.1, 5.137499999999999, 5.175, 5.2124999999999995, 5.249999999999999, 5.2875, 5.324999999999999, 5.3625, 5.3999999999999995, 5.437499999999999, 5.475, 5.512499999999999, 5.55, 5.5874999999999995, 5.624999999999999, 5.6625, 5.699999999999999, 5.7375, 5.7749999999999995, 5.812499999999999, 5.85, 5.887499999999999, 5.925, 5.9624999999999995, 5.999999999999999, 6.0375, 6.074999999999999, 6.1125, 6.1499999999999995, 6.187499999999999, 6.225, 6.262499999999999, 6.3, 6.3374999999999995, 6.374999999999999, 6.4125, 6.449999999999999, 6.4875, 6.5249999999999995, 6.562499999999999, 6.6, 6.637499999999999, 6.675, 6.7124999999999995, 6.749999999999999, 6.7875, 6.824999999999999, 6.8625, 6.8999999999999995, 6.937499999999999, 6.975, 7.012499999999999, 7.05, 7.0874999999999995, 7.124999999999999, 7.1625, 7.199999999999999, 7.237499999999999, 7.2749999999999995, 7.312499999999999, 7.35, 7.387499999999999, 7.424999999999999, 7.4624999999999995, 7.499999999999999, 7.5375, 7.574999999999999, 7.612499999999999, 7.6499999999999995, 7.687499999999999, 7.725, 7.762499999999999, 7.799999999999999, 7.8374999999999995, 7.874999999999999, 7.9125, 7.949999999999999, 7.987499999999999, 8.025, 8.0625, 8.1, 8.1375, 8.174999999999999, 8.212499999999999, 8.25, 8.2875, 8.325, 8.362499999999999, 8.399999999999999, 8.4375, 8.475, 8.5125, 8.549999999999999, 8.587499999999999, 8.625, 8.6625, 8.7, 8.737499999999999, 8.774999999999999, 8.8125, 8.85, 8.8875, 8.924999999999999, 8.962499999999999, 9.0, 9.0375, 9.075, 9.112499999999999, 9.149999999999999, 9.1875, 9.225, 9.2625, 9.299999999999999, 9.337499999999999, 9.375, 9.4125, 9.45, 9.487499999999999, 9.524999999999999, 9.5625, 9.6, 9.6375, 9.674999999999999, 9.712499999999999, 9.75, 9.7875, 9.825, 9.862499999999999, 9.899999999999999, 9.9375, 9.975, 10.0125, 10.049999999999999, 10.087499999999999, 10.125, 10.1625, 10.2, 10.237499999999999, 10.274999999999999, 10.3125, 10.35, 10.3875, 10.424999999999999, 10.462499999999999, 10.5, 10.5375, 10.575, 10.612499999999999, 10.649999999999999, 10.6875, 10.725, 10.7625, 10.799999999999999, 10.837499999999999, 10.875, 10.9125, 10.95, 10.987499999999999, 11.024999999999999, 11.0625, 11.1, 11.1375, 11.174999999999999, 11.212499999999999, 11.25, 11.2875, 11.325, 11.362499999999999, 11.399999999999999, 11.4375, 11.475, 11.5125, 11.549999999999999, 11.587499999999999, 11.625, 11.6625, 11.7, 11.737499999999999, 11.774999999999999, 11.8125, 11.85, 11.8875, 11.924999999999999, 11.962499999999999, 12.0, 12.0375, 12.075, 12.112499999999999, 12.149999999999999, 12.1875, 12.225, 12.2625, 12.299999999999999, 12.337499999999999, 12.375, 12.4125, 12.45, 12.487499999999999, 12.524999999999999, 12.5625, 12.6, 12.6375, 12.674999999999999, 12.712499999999999, 12.75, 12.7875, 12.825, 12.862499999999999, 12.899999999999999, 12.9375, 12.975, 13.0125, 13.049999999999999, 13.087499999999999, 13.125, 13.1625, 13.2, 13.237499999999999, 13.274999999999999, 13.3125, 13.35, 13.3875, 13.424999999999999, 13.462499999999999, 13.5, 13.5375, 13.575, 13.612499999999999, 13.649999999999999, 13.6875, 13.725, 13.7625, 13.799999999999999, 13.837499999999999, 13.875, 13.9125, 13.95, 13.987499999999999, 14.024999999999999, 14.0625, 14.1, 14.1375, 14.174999999999999, 14.212499999999999, 14.25, 14.2875, 14.325, 14.362499999999999, 14.399999999999999, 14.437499999999998, 14.475, 14.5125, 14.549999999999999, 14.587499999999999, 14.624999999999998, 14.6625, 14.7, 14.737499999999999, 14.774999999999999, 14.812499999999998, 14.85, 14.8875, 14.924999999999999, 14.962499999999999, 14.999999999999998, 15.0375, 15.075, 15.112499999999999, 15.149999999999999, 15.187499999999998, 15.225, 15.2625, 15.299999999999999, 15.337499999999999, 15.374999999999998, 15.4125, 15.45, 15.487499999999999, 15.524999999999999, 15.562499999999998, 15.6, 15.6375, 15.674999999999999, 15.712499999999999, 15.749999999999998, 15.7875, 15.825, 15.862499999999999, 15.899999999999999, 15.937499999999998, 15.975, 16.0125, 16.05, 16.087500000000002, 16.125, 16.1625, 16.2, 16.2375, 16.275000000000002, 16.3125, 16.35, 16.3875, 16.425, 16.462500000000002, 16.5, 16.5375, 16.575, 16.6125, 16.650000000000002, 16.6875, 16.725, 16.7625, 16.8, 16.837500000000002, 16.875, 16.9125, 16.95, 16.9875, 17.025000000000002, 17.0625, 17.1, 17.1375, 17.175, 17.212500000000002, 17.25, 17.2875, 17.325, 17.3625, 17.400000000000002, 17.4375, 17.475, 17.5125, 17.55, 17.587500000000002, 17.625, 17.6625, 17.7, 17.7375, 17.775000000000002, 17.8125, 17.85, 17.8875, 17.925, 17.962500000000002, 18.0, 18.0375, 18.075, 18.1125, 18.150000000000002, 18.1875, 18.225, 18.2625, 18.3, 18.337500000000002, 18.375, 18.4125, 18.45, 18.4875, 18.525000000000002, 18.5625, 18.6, 18.6375, 18.675, 18.712500000000002, 18.75, 18.7875, 18.825, 18.8625, 18.900000000000002, 18.9375, 18.975, 19.0125, 19.05, 19.087500000000002, 19.125, 19.1625, 19.2, 19.2375, 19.275000000000002, 19.3125, 19.35, 19.3875, 19.425, 19.462500000000002, 19.5, 19.5375, 19.575, 19.6125, 19.650000000000002, 19.6875, 19.725, 19.7625, 19.8, 19.837500000000002, 19.875, 19.9125, 19.95, 19.9875, 20.025000000000002, 20.0625, 20.1, 20.1375, 20.175, 20.212500000000002, 20.25, 20.2875, 20.325, 20.3625, 20.400000000000002, 20.4375, 20.475, 20.5125, 20.55, 20.587500000000002, 20.625, 20.6625, 20.7, 20.7375, 20.775000000000002, 20.8125, 20.85, 20.8875, 20.925, 20.962500000000002, 21.0]
  out "Offline Pulse Energy":dbl=5.256561428571429
  out "Online Pulse Energy":dbl=5.263724285714285
  in  "Instrument Control":T5(tab)
  in  "Device In":refnum<visa-resource-name>="GPIB0::10::INSTR"
  in  "Settings":T6={"Module"=enum."WV Etalon TEC", "WV Online TEC"=23.071000000001693, "WV Online LD"=0.175, "WV Offline TEC"=29.506450000000473, "WV Offline LD"=0.17, "WV Etalon TEC"=26.6, "HSRL Etalon TEC"=22.51, "HSRL TEC"=18.639500000001075, "HSRL LD"=0.16} {"HSRL LD" min=0.0 max=0.18 step=0.001 format="%.3p"; "HSRL TEC" min=14.0 max=28.0 step=0.1 format="%.3g"; "WV Offline LD" min=0.0 max=0.18 step=0.001 format="%.3p"; "WV Online LD" min=0.0 max=0.18 step=0.001 format="%.3p"; "HSRL Etalon TEC" format="%.2g"; "WV Etalon TEC" format="%.2g"; "WV Offline TEC" min=16.0 max=30.0 step=0.1 format="%.3g"; "WV Online TEC" min=14.0 max=28.0 step=0.1 format="%.3g"}
  out "Readings":T7={"Pro8000"=TRUE, "WV OnLine TEC"=23.0788212, "WV Online TEC"=TRUE, "WV Online LD"=0.175066411, "WV Online LD"=TRUE, "WV Offline TEC"=29.5190372, "WV Offline TEC"=TRUE, "WV Offline LD"=0.170347661, "WV Offline LD"=TRUE, "WV EtalonTEC"=26.9652939, "WV Etalon TEC"=TRUE, "HSRL Etalon TEC"=22.8755722, "HSRL Etalon TEC"=TRUE, "HSRL TEC"=18.6511478, "HSRL TEC "=TRUE, "HSRL LD"=0.160250008, "HSRL LD"=TRUE} {"HSRL LD" format="%.3p"; "HSRL TEC" format="%.3g"; "WV Offline LD" format="%.3p"; "WV Online LD" format="%.3p"; "HSRL Etalon TEC" format="%.3g"; "WV EtalonTEC" format="%.3g"; "WV Offline TEC" format="%.3g"; "WV OnLine TEC" format="%.3g"}
  in  "Pulse B Polarity":enum32{"Low", "High"}(ring)=enum."High"
  in  "Pulse A Delay(ns)":u32=1040 min=80 max=327600
  in  "Pulse B Delay(ns)":u32=170000 min=80 max=327600 step=1
  in  "Accumulation Delay(ns)":u32=10 min=10 max=1270 step=1
  in  "Sync Pulse Polarity":enum32{"Low", "High"}(ring)=enum."High"
  in  "Pulse A Polarity":enum32{"Low", "High"}(ring)=enum."High"
  in  "Number of Bins":u32=560 min=2 max=4095 step=1
  in  "Number of Accumulates":u32=14285 min=1 max=32767 step=1
  in  "Time Resolution Per Bin(ns)":u32=250 min=5 max=1063 step=1
  out "AMCS_Profile":i32=12
  in  "WV Online Set (nm)":dbl=828.193 format="%.5f"
  out "WV Online Read (nm)":dbl=828.1930134212099 format="%.5f"
  out "WV Offline Read (nm)":dbl=828.29267102208 format="%.5f"
  in  "WV Offline Set (nm)":dbl=828.29265 format="%.5f"
  in  "Bristol In":i32=5
  out "Bristol Out":i32
  out "Online_Diff":dbl=1.3421209928310418e-05 format="%#_3e"
  out "Oflline_Diff":dbl=2.1022079977228714e-05 format="%#_3e"
  out "WV Online Locked":bool=TRUE
  out "WV Oflline Locked":bool=TRUE
  in  "calculate absorption cross sections":bool
  in  "Online_Tol":dbl=5e-05 format="%#_15g"
  in  "Cancel online":bool
  in  "Offline_Tol":dbl=5e-05 format="%#_15g"
  in  "Cancel Offline":bool
  in  "temp step size":dbl=0.0005 format="%#_6p"
  in  "HSRL_Tol":dbl=7.5e-05 format="%#_15g"
  out "HSRL_Diff":dbl=6.707882562295708e-05 format="%#_3e"
  in  "Cancel HSRL":bool
  out "HSRL Locked":bool=TRUE
  out "HSRL Read (nm)":dbl=780.2461870788256 format="%.5f"
  in  "HSRL Set (nm)":dbl=780.24612 format="%#.5f"
  in  "Smoothing Range":dbl=75.0
  in  "Total DIAL Integration Time (Minutes)":i32=3
  in  "Data Reads (number of loops)":i32=1
  in  "Total Aerosol Integration Time (Minutes)":dbl=0.08
  in  "Scalar Wait Time":u32
  out "Smoothed Bins":dbl=2.0
  out "gate size":dbl=37.5
  in  "Receiver Scale Factor":dbl=0.75
  in  "NewportIn":string
  in  "logging":bool
  out "Newport Device Key":string="1918-R 15120"
  in  "SampleSize":i32=2
  out "NewportRef":refnum<k24>
  in  "Switch Comm Port":refnum<visa-resource-name>="COM3"
  out "FF_On_Ref":refnum<file>
  out "FF_On_Ptr":i64=5787936 format="%.2p"
  out "FF_Off_Ref":refnum<file>
  out "FF_Off_Ptr":i64=5787936 format="%.2p"
  out "NF_On_Ref":refnum<file>
  out "NF_On_Ptr":i64=5787936 format="%.2p"
  out "NF_Off_Ref":refnum<file>
  out "NF_Off_Ptr":i64=5787936 format="%.2p"
  out "DataOpen":bool=TRUE
  out "File Path_Far Field (out)":string="C:\\Users\\H2ODial\\Desktop\\SharedTeleWVData\\171010FF\\22"
  out "File Path_Near Field (out)":string="C:\\Users\\H2ODial\\Desktop\\SharedTeleWVData\\171010NF\\22"
  in  "Data File DIR (in)":string="C:\\Users\\H2ODial\\Desktop\\SharedTeleWVData\\"
  out "TRHP":T8
  in  "WS visa":refnum<visa-resource-name>="COM12"
  in  "WS_On/Off":bool
  in  "bins":u32=560 min=2 max=4095 step=1
  out "y offset":u32=10
  in  "ns scale":u32=250
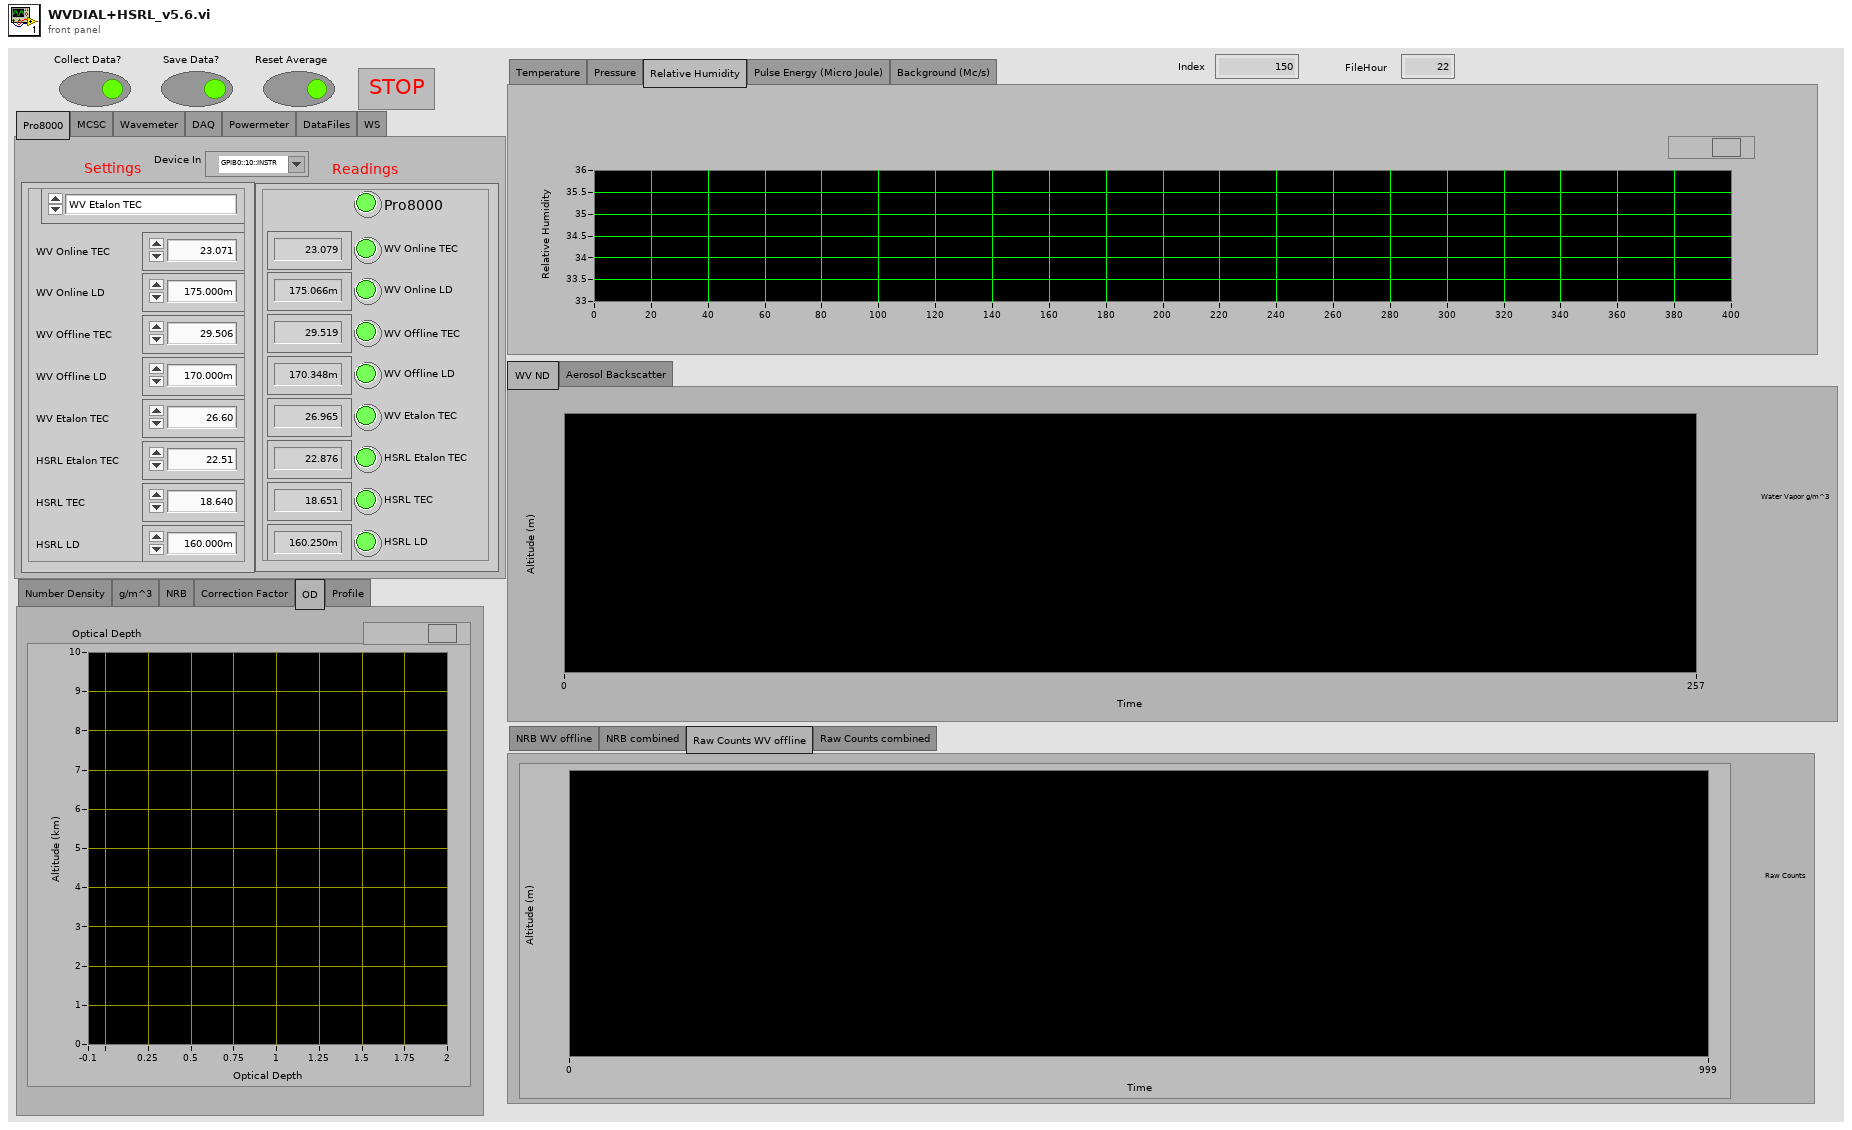
[diagram p1: front panel]
types:
  T1 = enum32{"NRB WV offline", "NRB combined", "Raw Counts WV offline", "Raw Counts combined"}
  T2 = enum32{"Number Density", "g/m^3", "NRB", "Correction Factor", "OD", "Profile"}
  T3 = enum32{"Temperature", "Pressure", "Relative Humidity", "Pulse Energy (Micro Joule)", "Background (Mc/s)"}
  T4 = cluster{"Online Pulse Energy":dbl, "Pulse Energy Offline":dbl}
  T5 = enum32{"Pro8000", "MCSC", "Wavemeter", "DAQ", "Powermeter", "DataFiles", "WS"}
  T6 = cluster{"Module":enum16{"WV Online TEC", "WV Online LD", "WV Offline TEC", "WV Offline LD", "WV Etalon TEC", "HSRL Etalon TEC", "HSRL TEC", "HSRL LD"}, "WV Online TEC":dbl, "WV Online LD":dbl, "WV Offline TEC":dbl, "WV Offline LD":dbl, "WV Etalon TEC":dbl, "HSRL Etalon TEC":dbl, "HSRL TEC":dbl, "HSRL LD":dbl}
  T7 = cluster{"Pro8000":bool, "WV OnLine TEC":dbl, "WV Online TEC":bool, "WV Online LD":dbl, "WV Online LD":bool, "WV Offline TEC":dbl, "WV Offline TEC":bool, "WV Offline LD":dbl, "WV Offline LD":bool, "WV EtalonTEC":dbl, "WV Etalon TEC":bool, "HSRL Etalon TEC":dbl, "HSRL Etalon TEC":bool, "HSRL TEC":dbl, "HSRL TEC ":bool, "HSRL LD":dbl, "HSRL LD":bool}
  T8 = cluster{"Temp C":dbl, "RelH %":dbl, "Press hPa":dbl, "AbH g/m^3":dbl}
  T9 = enum16{"Open_TL", "Close_TL", "Verify_ID", "TEC_Sensor", "SET", "READ", "ON", "OFF", "Set_Limits", "Read_Limits", "Enable_Status", "Read_Status"}
  T10 = enum16{"Initialize ILX", "Set ON T", "Set Off T", "Set ON I", "Set Off I", "Set On Lim", "Set Off Lim", "Read ILX", "TEC ON/OFF", "LASER ON/OFF", "Status?", "ILX OFF"}
  T11 = enum16{"open", "replace", "create", "open or create", "replace or create", "replace or create with confirmation"}
  T12 = enum16{"WV Online TEC", "WV Online LD", "WV Offline TEC", "WV Offline LD", "WV Etalon TEC", "HSRL Etalon TEC", "HSRL TEC", "HSRL LD"}
  T13 = cluster{"Temp":dbl, "RelH":dbl, "Press":dbl, "AbH":dbl}
  T14 = typedef "LVDateTimeRec.ctl" = cluster{"fractional second":dbl, "second":i32, "minute":i32, "hour":i32, "day of month":i32, "month":i32, "year":i32, "day of week":i32, "day of year":i32, "DST":i32}
  T15 = cluster{"Online Pulse Energy":dbl, "Offline Pulse Energy":dbl}
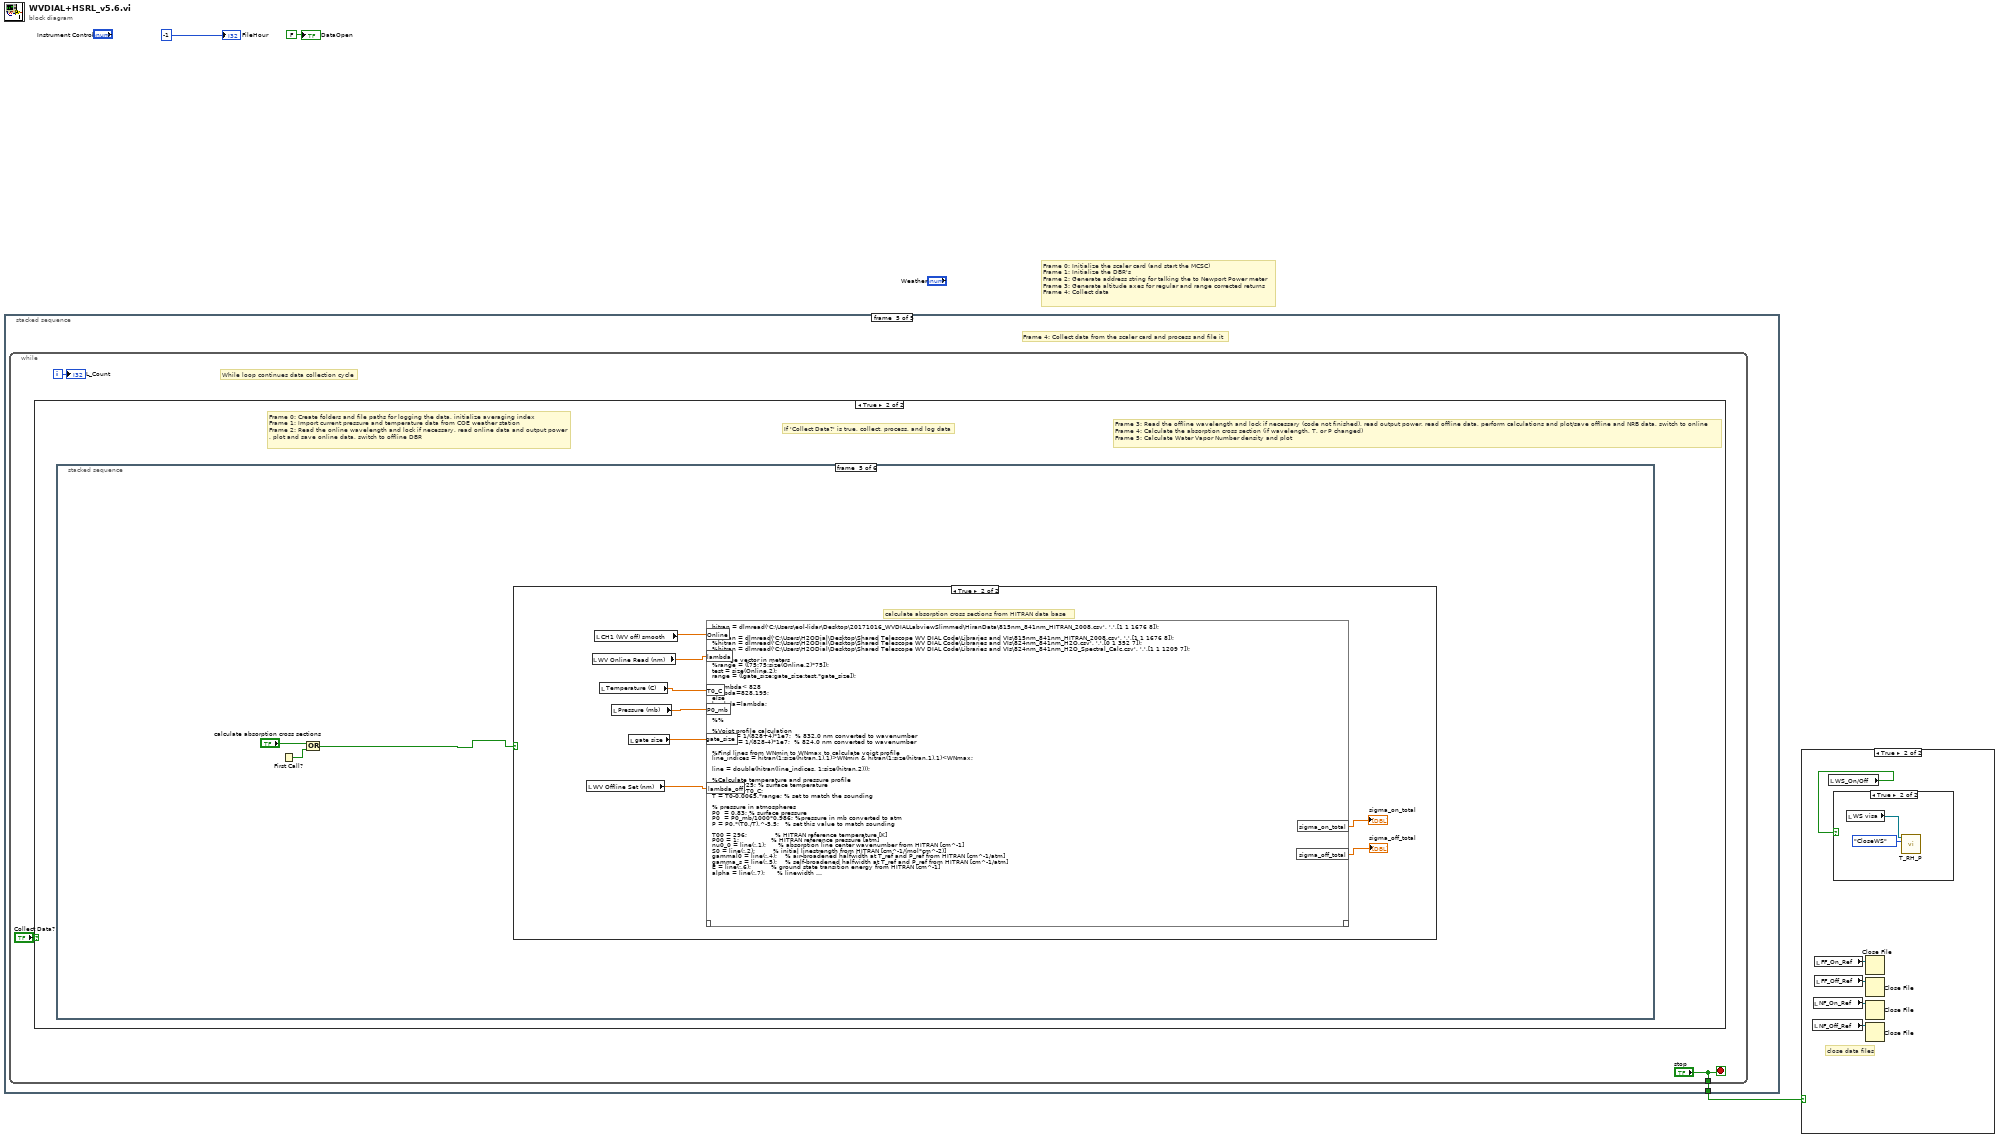
[diagram p0: block diagram]
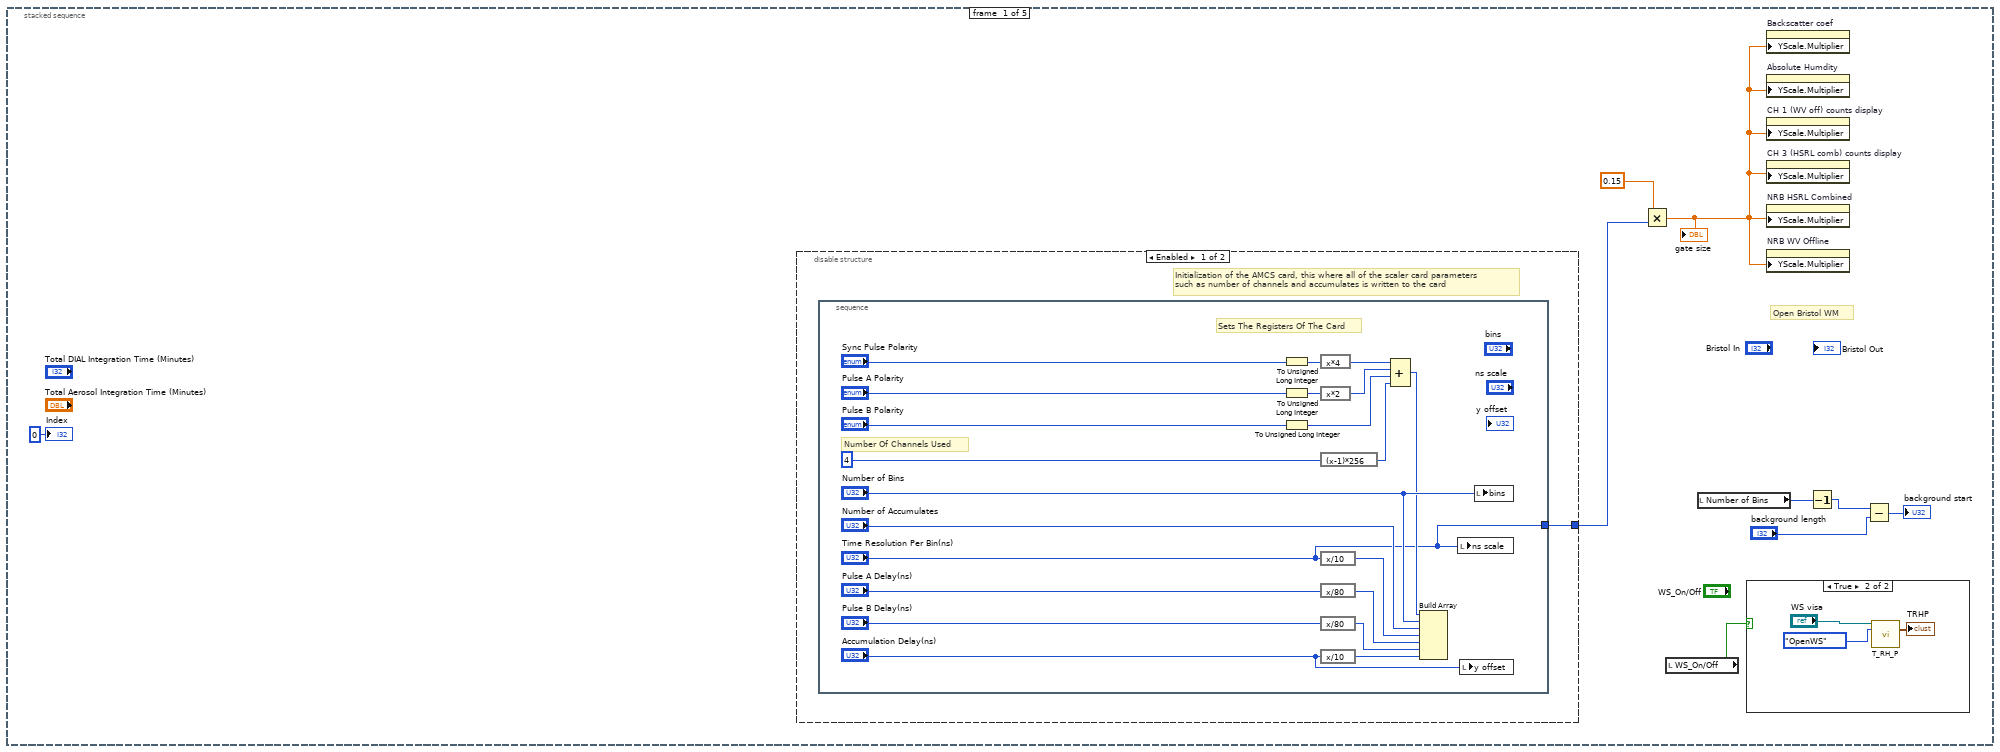
[diagram p4: hidden frame]
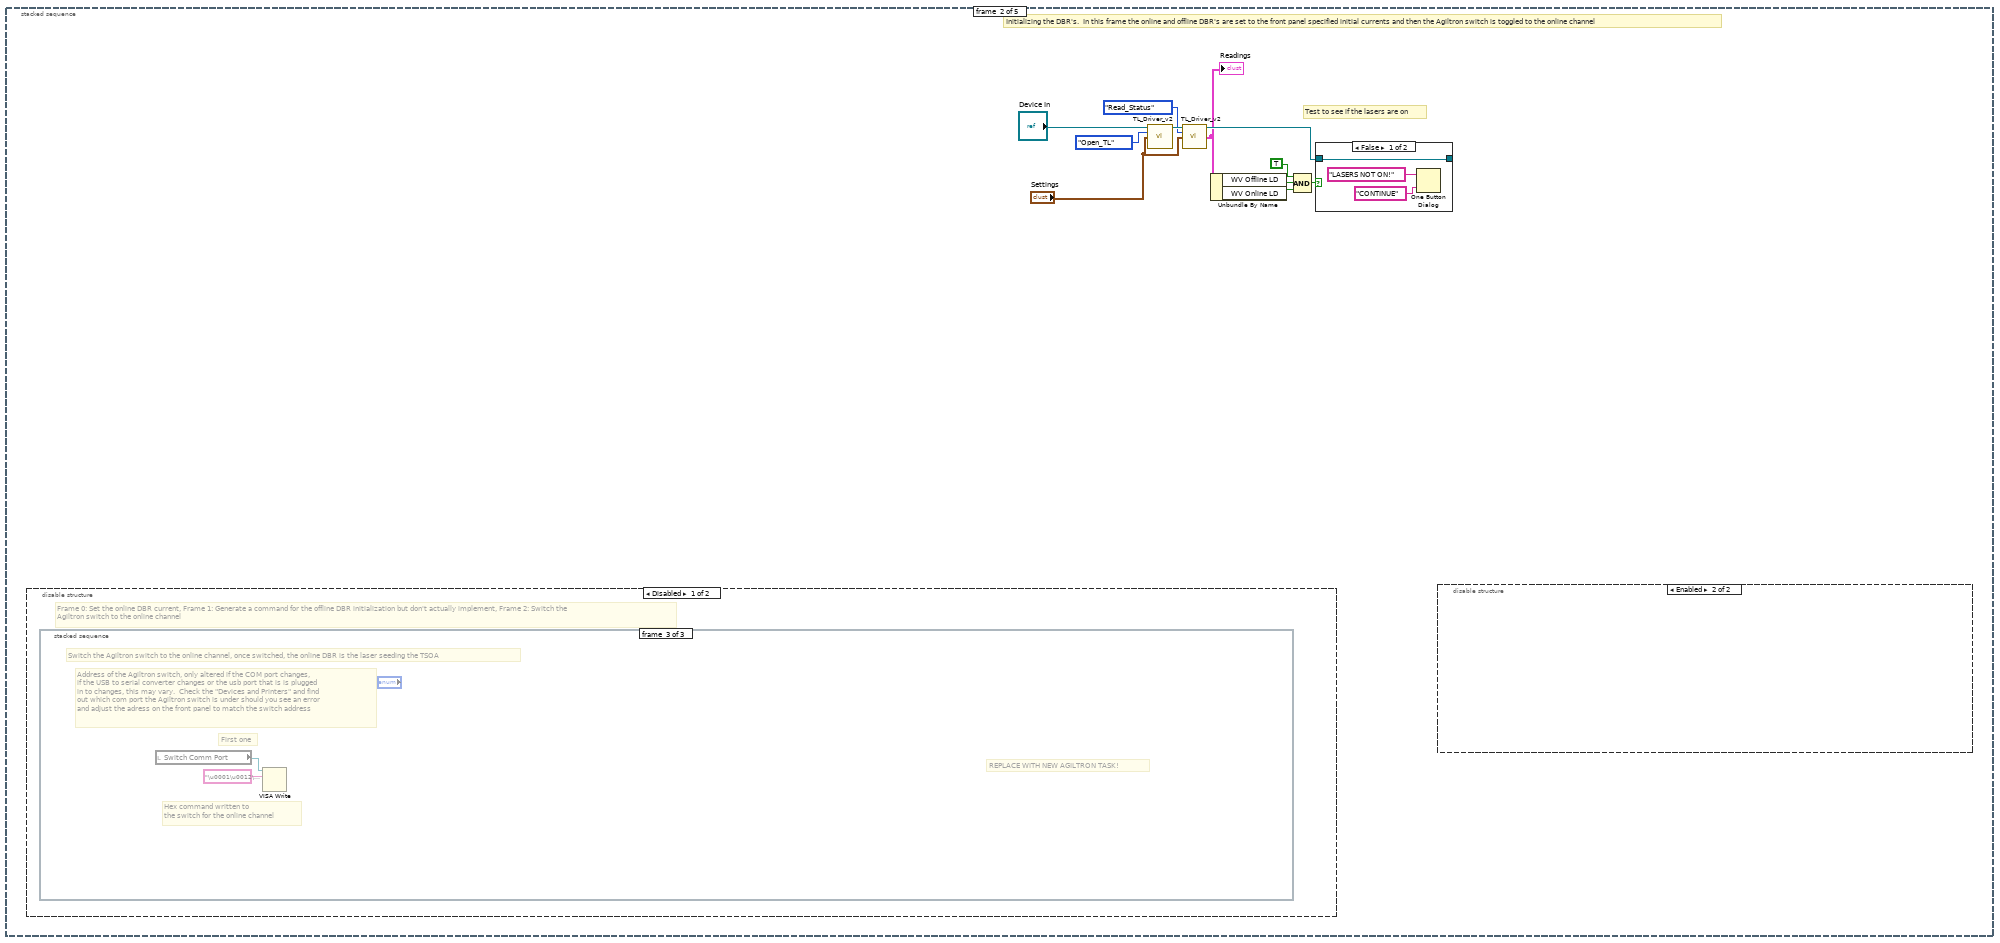
[diagram p7: hidden frame]
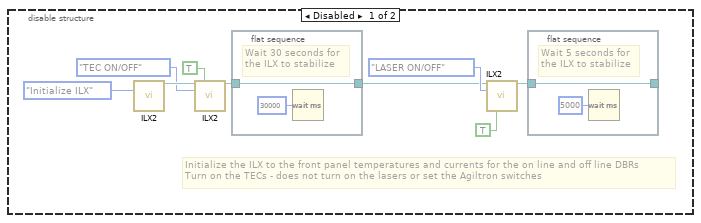
[diagram p9: hidden frame]
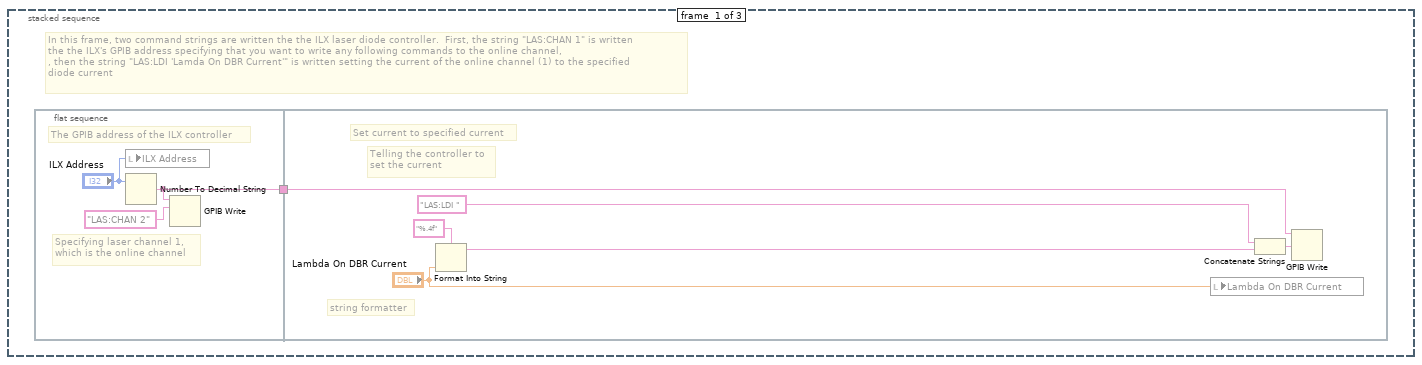
[diagram p10: hidden frame]
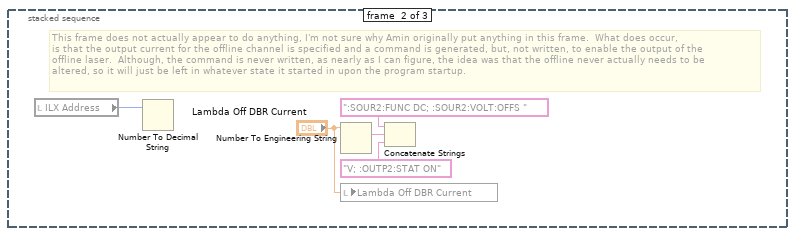
[diagram p11: hidden frame]
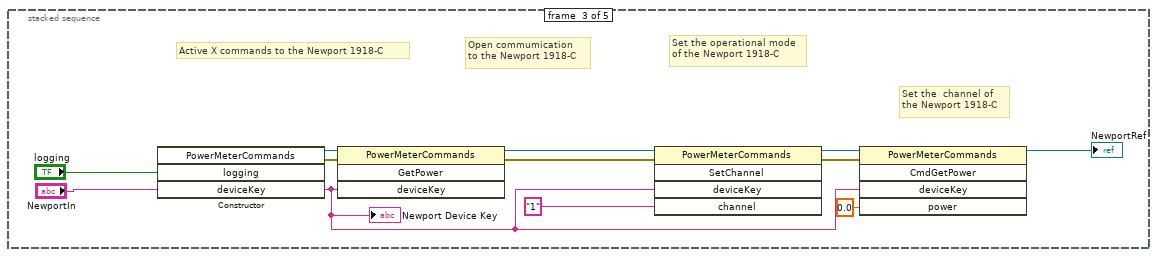
[diagram p13: hidden frame]
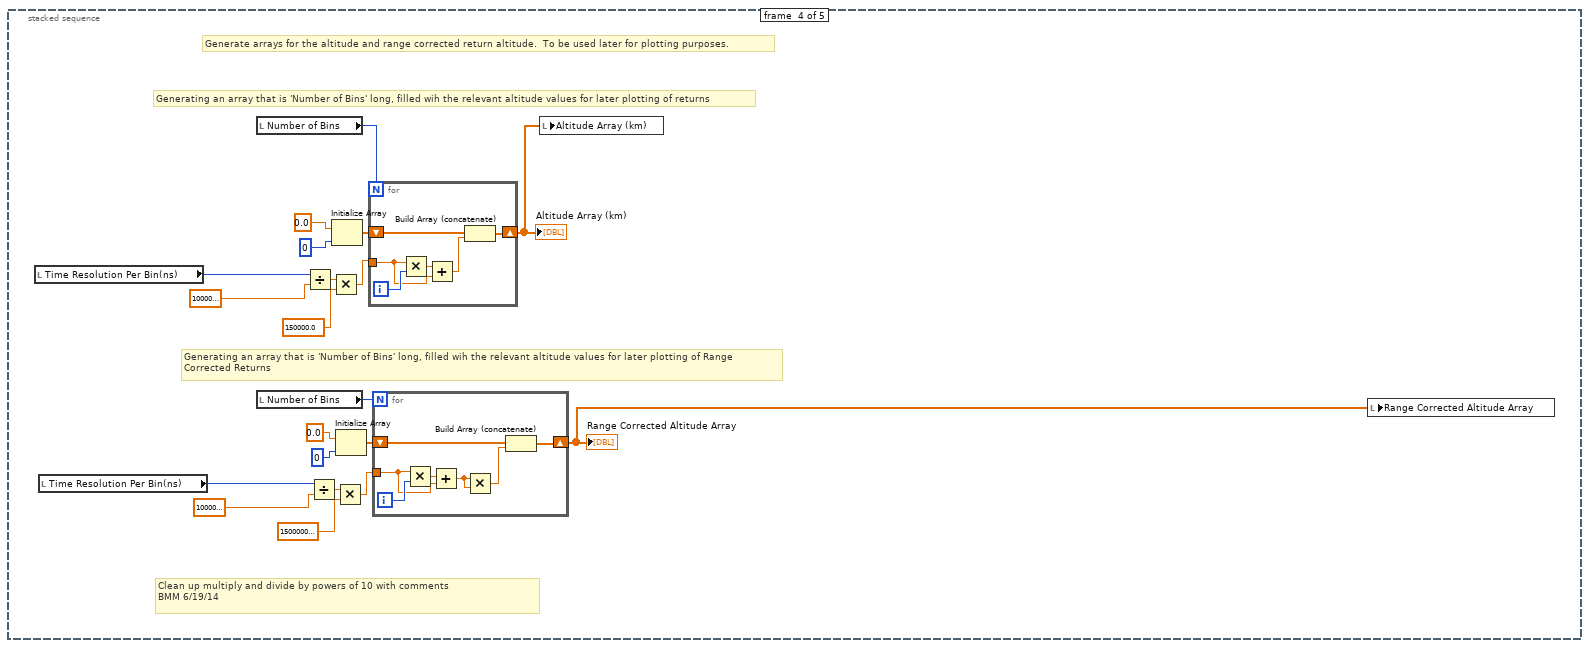
[diagram p14: hidden frame]
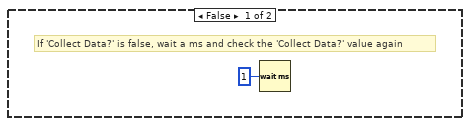
[diagram p15: hidden frame]
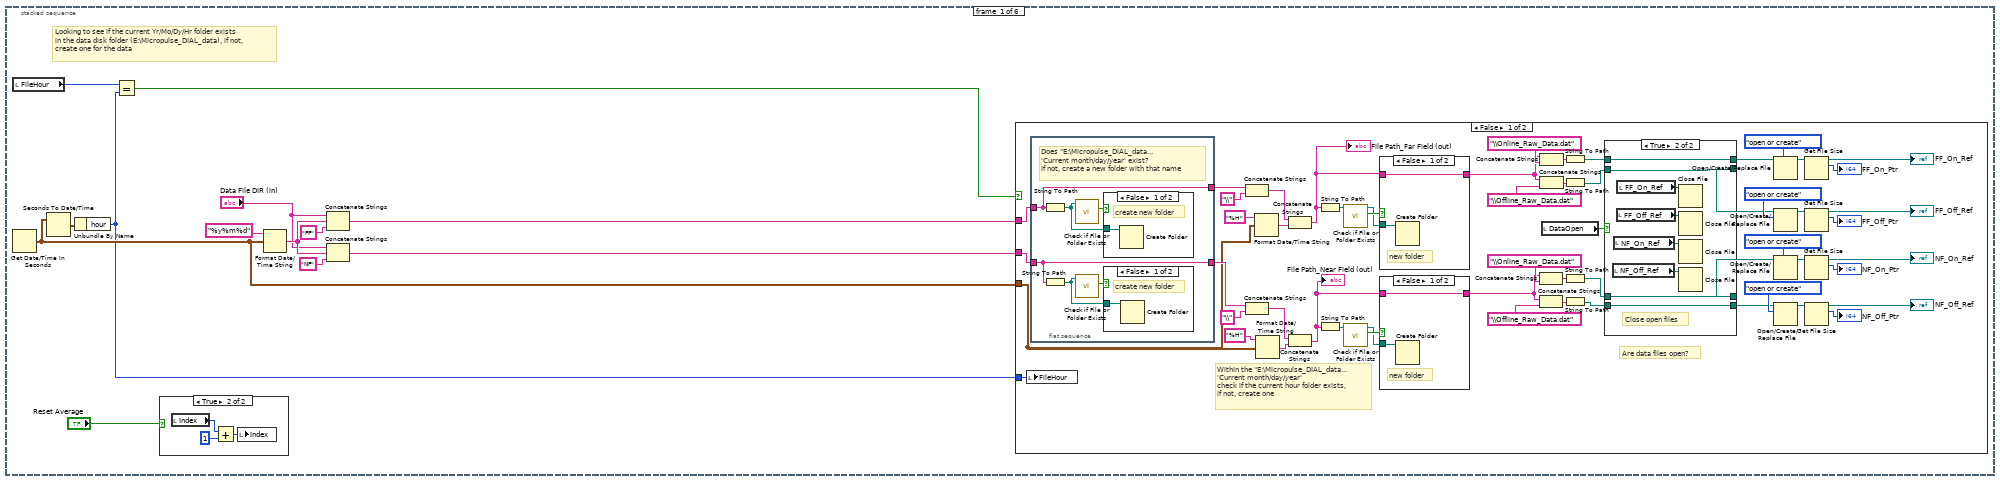
[diagram p16: hidden frame]
diagram:
  # "Frame 0: Initialize the scaler card (and start the MCSC)\nFrame 1: Initialize the DBR's\nFrame 2: Generate address string for talking the to Newport Power meter\nFrame 3: Generate altitude axes for regular and range corrected returns\nFrame 4: Collect data"
  n1 = stacked-sequence {
    tunnel: [_ _ _ _ w128] -> w3
    frame #0 {
      # "Open Bristol WM"
      n2 = disable-structure shown="Enabled" {
        disable-tunnel: [w16 _] -> w5
        frame Enabled {
          # "Initialization of the AMCS card, this where all of the scaler card parameters\nsuch as number of channels and accumulates is written to the card"
          n3 = stacked-sequence {
            tunnel: ["Time Resolution Per Bin(ns)"] -> w16
            frame #0 {
              # "Sets The Registers Of The Card"
              # "Number Of Channels Used"
              n4 = To Unsigned Long Integer(number="Sync Pulse Polarity") -> (unsigned 32bit integer=w18:u32)
              n5 = To Unsigned Long Integer(number="Pulse A Polarity") -> (unsigned 32bit integer=w22:u32)
              n6 = To Unsigned Long Integer(number="Pulse B Polarity") -> (unsigned 32bit integer=w20:u32)
              n7 = expression code="x*4"(w18) -> (w27:u32)
              n8 = expression code="x*2"(w22) -> (w26:u32)
              n9 = expression code="(x-1)*256"(u32 4 ("Number of Channels Used")) -> (w25:u32)
              n10 = expression code="x/10"("Time Resolution Per Bin(ns)") -> (w28:u32)
              n11 = expression code="x/80"("Pulse A Delay(ns)") -> (w35:u32)
              n12 = expression code="x/80"("Pulse B Delay(ns)") -> (w37:u32)
              n13 = expression code="x/10"("Accumulation Delay(ns)") -> (w36:u32)
              n14 = Compound Arithmetic op=ADD(w27, w26, w20, w25) -> (w24:u32)
              n15 = Build Array(w24, "Number of Bins", "Number of Accumulates", w28, w35, w37, w36) -> ()  [unwired: 1 out]
              n16 = local write "ns scale"("Time Resolution Per Bin(ns)") -> ()
              n17 = local write "y offset"("Accumulation Delay(ns)") -> ()
              n18 = local write "bins"("Number of Bins") -> ()
            }
          }
        }
        frame Disabled {
        }
      }
      n19 = Multiply(x=0.15, y=w5) -> (x*y=w4:dbl)
      "gate size" <- w4
      n20 = local read "WS_On/Off"() -> (w7:bool)
      n21 = local read "Number of Bins"() -> (w11:u32)
      n22 = case shown="True" w7 {
        frame False {
        }
        frame True {
          n23 = call "T_RH_P.vi"("VISA in"="WS visa", "WS_Commands"=enum16{"OpenWS", "ReadTRHP", "CloseWS"}."OpenWS") -> ("TRHP"=→"TRHP":T13)  [unwired: 11 in, 2 out]
        }
      }
      n24 = property on="Backscatter coef" class="IntChart (strict)"("YScale.Multiplier"=w4) -> ()  [unwired: 2 in, 2 out]
      n25 = property on="Absolute Humdity" class="IntChart (strict)"("YScale.Multiplier"=w4) -> ()  [unwired: 2 in, 2 out]
      n26 = property on="CH 1 (WV off) counts display" class="IntChart (strict)"("YScale.Multiplier"=w4) -> ()  [unwired: 2 in, 2 out]
      n27 = property on="CH 3 (HSRL comb) counts display" class="IntChart (strict)"("YScale.Multiplier"=w4) -> ()  [unwired: 2 in, 2 out]
      n28 = property on="NRB HSRL Combined" class="IntChart (strict)"("YScale.Multiplier"=w4) -> ()  [unwired: 2 in, 2 out]
      n29 = property on="NRB WV Offline" class="IntChart (strict)"("YScale.Multiplier"=w4) -> ()  [unwired: 2 in, 2 out]
      n30 = Decrement(x=w11) -> (x-1=w10:u32)
      n31 = Subtract(x=w10, y="background length") -> (x-y=→"background start":u32)
      "Index" <- 0 ("Index")
    }
    frame #1 {
      # "Test to see if the lasers are on"
      # "Initializing the DBR's.  In this frame the online and offline DBR's are set to the front panel specified initial currents and then the Agiltron switch is toggled to the online channel"
      n32 = disable-structure shown="Disabled" {
        frame Disabled {
          # "Frame 0: Set the online DBR current, Frame 1: Generate a command for the offline DBR initialization but don't actually implement, Frame 2: Switch the \nAgiltron switch to the online channel"
          n33 = stacked-sequence {
            frame #0 {
              # "In this frame, two command strings are written the the ILX laser diode controller.  First, the string \"LAS:CHAN 1\" is written\nthe the ILX's GPIB address specifying that you want to write any following commands to the online channel,\n, then the string \"LAS:LDI 'Lamda On DBR Current'\" is written setting the current of the online channel (1) to the specified \ndiode current"
              n34 = flat-sequence {
                tunnel: [w68] -> w66
                tunnel: w66 -> [w70]
                frame #0 {
                  # "The GPIB address of the ILX controller"
                  # "Specifying laser channel 1,\nwhich is the online channel"
                  n35 = local write "ILX Address"("ILX Address") -> ()
                  n36 = Number To Decimal String(number="ILX Address") -> (decimal integer string=w68:string)  [unwired: 1 in]
                  n37 = GPIB Write(0:w68, 1:"LAS:CHAN 2") -> ()  [unwired: 3 in, 2 out]
                }
                frame #1 {
                  # "Telling the controller to\nset the current"
                  # "string formatter"
                  # "Set current to specified current"
                  n38 = Format Into String(format string="%.4f" ("Format String"), "Lambda On DBR Current") -> (resulting string=w73:string)  [unwired: 2 in, 1 out]
                  n39 = local write "Lambda On DBR Current"("Lambda On DBR Current") -> ()
                  n40 = Concatenate Strings("LAS:LDI ", w73) -> (w74:string)
                  n41 = GPIB Write(0:w70, 1:w74) -> ()  [unwired: 3 in, 2 out]
                }
              }
            }
            frame #1 {
              # "This frame does not actually appear to do anything, I'm not sure why Amin originally put anything in this frame.  What does occur, \nis that the output current for the offline channel is specified and a command is generated, but, not written, to enable the output of the\noffline laser.  Although, the command is never written, as nearly as I can figure, the idea was that the offline never actually needs to be \naltered, so it will just be left in whatever state it started in upon the program startup."
              n42 = local read "ILX Address"() -> (w76:i32)
              n43 = Number To Decimal String(number=w76) -> ()  [unwired: 1 in, 1 out]
              n44 = Number To Engineering String(4:"Lambda Off DBR Current") -> (0:w80:string)  [unwired: 3 in]
              n45 = local write "Lambda Off DBR Current"("Lambda Off DBR Current") -> ()
              n46 = Concatenate Strings(":SOUR2:FUNC DC; :SOUR2:VOLT:OFFS ", w80, "V; :OUTP2:STAT ON") -> ()  [unwired: 1 out]
            }
            frame #2 {
              # "REPLACE WITH NEW AGILTRON TASK!"
              # "First one"
              # "Address of the Agiltron switch, only altered if the COM port changes,\nif the USB to serial converter changes or the usb port that is is plugged\nin to changes, this may vary.  Check the \"Devices and Printers\" and find \nout which com port the Agiltron switch is under should you see an error \nand adjust the adress on the front panel to match the switch address"
              # "Hex command written to \nthe switch for the online channel"
              # "Switch the Agiltron switch to the online channel, once switched, the online DBR is the laser seeding the TSOA"
              n47 = local read "Switch Comm Port"() -> (w81:refnum<visa-resource-name>)
              n48 = VISA Write(VISA resource name=w81, write buffer="\u0001\u0012\u0000\u0002") -> ()  [unwired: 1 in, 3 out]
            }
          }
        }
        frame Enabled {
        }
      }
      n49 = call "TL_Driver_v2.vi"("Device In"="Device In", "Commands"=T9."Open_TL", "Settings"="Settings") -> ("Device Out"=w46:refnum<visa-resource-name>)  [unwired: 9 in, 3 out]
      n50 = call "TL_Driver_v2.vi"("Device In"=w46, "Commands"=T9."Read_Status", "Settings"="Settings") -> ("Device Out"=w44:refnum<visa-resource-name>, "Readings"=w38:T7)  [unwired: 9 in, 2 out]
      "Readings" <- w38
      n51 = Unbundle By Name(w38) -> ("WV Offline LD"=w41:bool, "WV Online LD"=w42:bool)
      n52 = Compound Arithmetic op=AND(TRUE, w41, w42) -> (w40:bool)
      n53 = case shown="False" w40 {
        tunnel: w44 -> [w49 w52]
        tunnel: [w49 w52] -> _
        frame False {
          n54 = One Button Dialog(message="LASERS NOT ON!", button name ("OK")="CONTINUE") -> ()  [unwired: 1 out]
        }
        frame True {
        }
      }
      n55 = disable-structure shown="Enabled" {
        frame Disabled {
          # "Initialize the ILX to the front panel temperatures and currents for the on line and off line DBRs\nTurn on the TECs - does not turn on the lasers or set the Agiltron switches"
          n56 = call "ILX2.vi"("ILX Command"=T10."Initialize ILX") -> ("Device Out"=w60:refnum<visa-resource-name>)  [unwired: 10 in, 4 out]
          n57 = call "ILX2.vi"("Device In"=w60, "TEC Control"=TRUE, "ILX Command"=T10."TEC ON/OFF") -> ("Device Out"=w57:refnum<visa-resource-name>)  [unwired: 8 in, 4 out]
          n58 = flat-sequence {
            tunnel: w57 -> [w64]
            tunnel: [w64] -> w54
            frame #0 {
              # "Wait 30 seconds for\nthe ILX to stabilize"
              n59 = Wait (ms)(milliseconds to wait=u32 30000) -> ()  [unwired: 1 out]
            }
          }
          n60 = call "ILX2.vi"("Device In"=w54, "ILX Command"=T10."LASER ON/OFF", "Laser Control"=TRUE ("TEC Control")) -> ("Device Out"=w53:refnum<visa-resource-name>)  [unwired: 8 in, 4 out]
          n61 = flat-sequence {
            tunnel: w53 -> [w62]
            tunnel: [w62] -> _
            frame #0 {
              # "Wait 5 seconds for\nthe ILX to stabilize"
              n62 = Wait (ms)(milliseconds to wait=u32 5000) -> ()  [unwired: 1 out]
            }
          }
        }
        frame Enabled {
        }
      }
    }
    frame #2 {
      # "Active X commands to the Newport 1918-C"
      # "Set the  channel of\nthe Newport 1918-C"
      # "Set the operational mode\nof the Newport 1918-C"
      # "Open commumication\nto the Newport 1918-C"
      n63 = constructor class="PowerMeterCommands"("logging"="logging", "deviceKey"="NewportIn") -> (reference out=w94:refnum<k24>, error out=w91:errorcluster, "deviceKey"=w86:string)  [unwired: 3 in, 2 out]
      "Newport Device Key" <- w86
      n64 = invoke class="PowerMeterCommands" method="GetPower"(reference=w94, error in=w91, "deviceKey"=w86) -> (reference out=w93:refnum<k24>, error out=w90:errorcluster)  [unwired: 1 in, 2 out]
      n65 = invoke class="PowerMeterCommands" method="SetChannel"(reference=w93, error in=w90, "deviceKey"=w86, "channel"="1") -> (reference out=w87:refnum<k24>, error out=w89:errorcluster)  [unwired: 1 in, 3 out]
      n66 = invoke class="PowerMeterCommands" method="CmdGetPower"(reference=w87, error in=w89, "deviceKey"=w86, "power"=sgl 0.0) -> (reference out=→"NewportRef":refnum<k24>)  [unwired: 1 in, 4 out]
    }
    frame #3 {
      # "Clean up multiply and divide by powers of 10 with comments\nBMM 6/19/14"
      # "Generating an array that is 'Number of Bins' long, filled wih the relevant altitude values for later plotting of Range \nCorrected Returns"
      # "Generating an array that is 'Number of Bins' long, filled wih the relevant altitude values for later plotting of returns"
      # "Generate arrays for the altitude and range corrected return altitude.  To be used later for plotting purposes."
      n67 = local read "Time Resolution Per Bin(ns)"() -> (w107:u32)
      n68 = local read "Time Resolution Per Bin(ns)"() -> (w97:u32)
      n69 = local read "Number of Bins"() -> (w110:u32)
      n70 = local read "Number of Bins"() -> (w100:u32)
      n71 = Divide(x=w107, y=1000000000.0) -> (x/y=w105:dbl)
      n72 = Divide(x=w97, y=1000000000.0) -> (x/y=w95:dbl)
      n73 = Multiply(x=w105, y=150000.0) -> (x*y=w108:dbl)
      n74 = Initialize Array(0.0, 0) -> (w113:dbl[])
      n75 = Multiply(x=w95, y=150000000.0) -> (x*y=w98:dbl)
      n76 = Initialize Array(0.0, 0) -> (w103:dbl[])
      n77 = for {
        N: w110 -> [_]
        shift-right: [w126] -> w111
        shift-left: w113 -> [w127]
        tunnel: w108 -> [w123]
        i -> [w125]
        n78 = Multiply(x=w123, y=w125) -> (x*y=w124:dbl)
        n79 = Add(x=w124, y=w123) -> (x+y=w122:dbl)
        n80 = Build Array (concatenate)(w127, w122) -> (w126:dbl[])
      }
      "Altitude Array (km)" <- w111
      n81 = for {
        N: w100 -> [_]
        shift-right: [w120] -> w101
        shift-left: w103 -> [w121]
        tunnel: w98 -> [w116]
        i -> [w119]
        n82 = Multiply(x=w116, y=w119) -> (x*y=w117:dbl)
        n83 = Add(x=w117, y=w116) -> (x+y=w115:dbl)
        n84 = Multiply(x=w115, y=w115) -> (x*y=w118:dbl)
        n85 = Build Array (concatenate)(w121, w118) -> (w120:dbl[])
      }
      "Range Corrected Altitude Array" <- w101
      n86 = local write "Altitude Array (km)"(w111) -> ()
      n87 = local write "Range Corrected Altitude Array"(w101) -> ()
    }
    frame #4 {
      # "Frame 4: Collect data from the scaler card and process and file it"
      n88 = while {
        tunnel: ["stop"] -> w128
        i -> [w129]
        stop <- "stop" stop-if-true
        # "While loop continues data collection cycle"
        n89 = case shown="True" "Collect Data?" {
          frame False {
            # "If 'Collect Data?' is false, wait a ms and check the 'Collect Data?' value again"
            n90 = Wait (ms)(milliseconds to wait=u32 1) -> ()  [unwired: 1 out]
          }
          frame True {
            # "Frame 3: Read the offline wavelength and lock if necessary (code not finished), read output power, read offline data, perform calculations and plot/save offline and NRB data, switch to online\nFrame 4: Calculate the absorption cross section (if wavelength, T, or P changed)\nFrame 5: Calculate Water Vapor Number density and plot"
            # "Frame 0: Create folders and file paths for logging the data, initialize averaging index\nFrame 1: Import current pressure and temperature data from COE weather station\nFrame 2: Read the online wavelength and lock if necessary, read online data and output power\n, plot and save online data, switch to offline DBR"
            # "If 'Collect Data?' is true, collect, process, and log data"
            n91 = stacked-sequence {
              frame #0 {
                # "Looking to see if the current Yr/Mo/Dy/Hr folder exists\nin the data disk folder (E:\\Micropulse_DIAL_data), if not,\ncreate one for the data"
                n92 = local read "FileHour"() -> (w142:i32)
                n93 = Get Date/Time In Seconds() -> (seconds since 1Jan1904=w134:timestamp)
                n94 = Seconds To Date/Time(time stamp (now)=w134) -> (date time rec=w144:T14)  [unwired: 1 in]
                n95 = Unbundle By Name(w144) -> ("hour"=w133:i32)
                n96 = Equal?(x=w142, y=w133) -> (x = y?=w143:bool)
                n97 = case shown="True" "Reset Average" {
                  frame False {
                    n98 = local write "Index"(0 ("Index")) -> ()
                  }
                  frame True {
                    n99 = local read "Index"() -> (w232:i32)
                    n100 = Add(x=w232, y=1) -> (x+y=w231:i32)
                    n101 = local write "Index"(w231) -> ()
                  }
                }
                n102 = Format Date/Time String(time format string (%c)="%y%m%d", seconds (now)=w134) -> (date/time string=w138:string)  [unwired: 1 in]
                n103 = Concatenate Strings("Data File DIR (in)", w138, "FF" ("string")) -> (w140:string)
                n104 = Concatenate Strings("Data File DIR (in)", w138, "NF" ("string")) -> (w135:string)
                n105 = case shown="False" w143 {
                  tunnel: w140 -> [w202 _]
                  tunnel: w135 -> [w201 _]
                  tunnel: w134 -> [w188 _]
                  tunnel: w133 -> [w164 _]
                  frame False {
                    # "Are data files open?"
                    # "Within the \"E:\\Micropulse_DIAL_data...\n'Current month/day/year' \ncheck if the current hour folder exists,\nif not, create one"
                    n106 = local write "FileHour"(w164) -> ()
                    n107 = flat-sequence {
                      tunnel: [w222] -> w189
                      tunnel: w202 -> [w221]
                      tunnel: w201 -> [w222]
                      tunnel: [w221] -> w190
                      frame #0 {
                        # "Does \"E:\\Micropulse_DIAL_data...\n'Current month/day/year' exist?\nIf not, create a new folder with that name"
                        n108 = String To Path(string=w221) -> (path=w226:path)
                        n109 = String To Path(string=w222) -> (path=w224:path)
                        n110 = call <vilib>:"Check if File or Folder Exists.vi"("path"=w226) -> ("file or folder exists?"=w225:bool)  [unwired: 8 in, 2 out]
                        n111 = call <vilib>:"Check if File or Folder Exists.vi"("path"=w224) -> ("file or folder exists?"=w223:bool)  [unwired: 8 in, 2 out]
                        n112 = case shown="False" w225 {
                          tunnel: w226 -> [w228 _]
                          frame False {
                            # "create new folder"
                            n113 = Create Folder(path (use dialog)=w228) -> ()  [unwired: 2 in, 3 out]
                          }
                          frame True {
                            # "Folder exists\ndo nothing"
                          }
                        }
                        n114 = case shown="False" w223 {
                          tunnel: w224 -> [w227 _]
                          frame False {
                            # "create new folder"
                            n115 = Create Folder(path (use dialog)=w227) -> ()  [unwired: 2 in, 3 out]
                          }
                          frame True {
                            # "Folder exists\ndo nothing"
                          }
                        }
                      }
                    }
                    n116 = Concatenate Strings(w190, "\\" ("string")) -> (w197:string)
                    n117 = Concatenate Strings(w189, "\\" ("string")) -> (w192:string)
                    n118 = Format Date/Time String(time format string (%c)="%H", seconds (now)=w188) -> (date/time string=w200:string)  [unwired: 1 in]
                    n119 = Format Date/Time String(time format string (%c)="%H", seconds (now)=w188) -> (date/time string=w195:string)  [unwired: 1 in]
                    n120 = Concatenate Strings(w197, w200) -> (w160:string)
                    "File Path_Far Field (out)" <- w160
                    n121 = Concatenate Strings(w192, w195) -> (w161:string)
                    "File Path_Near Field (out)" <- w161
                    n122 = String To Path(string=w160) -> (path=w198:path)
                    n123 = String To Path(string=w161) -> (path=w193:path)
                    n124 = call <vilib>:"Check if File or Folder Exists.vi"("path"=w198) -> ("file or folder exists?"=w187:bool, "dup path"=w185:path)  [unwired: 8 in, 1 out]
                    n125 = call <vilib>:"Check if File or Folder Exists.vi"("path"=w193) -> ("file or folder exists?"=w186:bool, "dup path"=w184:path)  [unwired: 8 in, 1 out]
                    n126 = case shown="False" w187 {
                      tunnel: w185 -> [w219 _]
                      tunnel: w160 -> [w218 w220]
                      tunnel: [w218 w220] -> w158
                      frame False {
                        # "new folder"
                        n127 = Create Folder(path (use dialog)=w219) -> ()  [unwired: 2 in, 3 out]
                      }
                      frame True {
                        # "Folder exists\ndo nothing"
                      }
                    }
                    n128 = case shown="False" w186 {
                      tunnel: w184 -> [w216 _]
                      tunnel: w161 -> [w215 w217]
                      tunnel: [w215 w217] -> w159
                      frame False {
                        # "new folder"
                        n129 = Create Folder(path (use dialog)=w216) -> ()  [unwired: 2 in, 3 out]
                      }
                      frame True {
                        # "Folder exists\ndo nothing"
                      }
                    }
                    n130 = Concatenate Strings(w159, "\\Online_Raw_Data.dat" ("string")) -> (w178:string)
                    n131 = Concatenate Strings(w159, "\\Offline_Raw_Data.dat" ("string")) -> (w177:string)
                    n132 = Concatenate Strings(w158, "\\Online_Raw_Data.dat" ("string")) -> (w183:string)
                    n133 = Concatenate Strings(w158, "\\Offline_Raw_Data.dat" ("string")) -> (w182:string)
                    n134 = local read "DataOpen"() -> (w175:bool)
                    n135 = String To Path(string=w183) -> (path=w174:path)
                    n136 = String To Path(string=w182) -> (path=w173:path)
                    n137 = String To Path(string=w178) -> (path=w172:path)
                    n138 = String To Path(string=w177) -> (path=w171:path)
                    n139 = case shown="True" w175 {
                      tunnel: w174 -> [w206 w210]
                      tunnel: [w206 w210] -> w168
                      tunnel: w173 -> [w205 w209]
                      tunnel: [w205 w209] -> w167
                      tunnel: w172 -> [w204 w208]
                      tunnel: [w204 w208] -> w166
                      tunnel: [w203 w207] -> w165
                      tunnel: w171 -> [w203 w207]
                      frame False {
                        # "No files open\ndo nothing"
                      }
                      frame True {
                        # "Close open files"
                        n140 = local read "NF_Off_Ref"() -> (w212:refnum<file>)
                        n141 = local read "NF_On_Ref"() -> (w211:refnum<file>)
                        n142 = local read "FF_Off_Ref"() -> (w214:refnum<file>)
                        n143 = local read "FF_On_Ref"() -> (w213:refnum<file>)
                        n144 = Close File(refnum=w213) -> ()  [unwired: 1 in, 2 out]
                        n145 = Close File(refnum=w214) -> ()  [unwired: 1 in, 2 out]
                        n146 = Close File(refnum=w211) -> ()  [unwired: 1 in, 2 out]
                        n147 = Close File(refnum=w212) -> ()  [unwired: 1 in, 2 out]
                      }
                    }
                    n148 = Open/Create/Replace File(file path (use dialog)=w168, operation (0:open)=T11."open or create") -> (refnum out=w154:refnum<file>)  [unwired: 4 in, 2 out]
                    n149 = Open/Create/Replace File(file path (use dialog)=w167, operation (0:open)=T11."open or create") -> (refnum out=w155:refnum<file>)  [unwired: 4 in, 2 out]
                    n150 = Open/Create/Replace File(file path (use dialog)=w166, operation (0:open)=T11."open or create") -> (refnum out=w156:refnum<file>)  [unwired: 4 in, 2 out]
                    n151 = Open/Create/Replace File(file path (use dialog)=w165, operation (0:open)=T11."open or create") -> (refnum out=w157:refnum<file>)  [unwired: 4 in, 2 out]
                    n152 = Get File Size(file=w154) -> (refnum out=→"FF_On_Ref":refnum<file>, size (in bytes)=→"FF_On_Ptr":i64)  [unwired: 1 in, 1 out]
                    n153 = Get File Size(file=w155) -> (refnum out=→"FF_Off_Ref":refnum<file>, size (in bytes)=→"FF_Off_Ptr":i64)  [unwired: 1 in, 1 out]
                    n154 = Get File Size(file=w156) -> (refnum out=→"NF_On_Ref":refnum<file>, size (in bytes)=→"NF_On_Ptr":i64)  [unwired: 1 in, 1 out]
                    n155 = Get File Size(file=w157) -> (refnum out=→"NF_Off_Ref":refnum<file>, size (in bytes)=→"NF_Off_Ptr":i64)  [unwired: 1 in, 1 out]
                  }
                  frame True {
                    # "Don't need to do anything!"
                  }
                }
              }
              frame #1 {
                # "Writing and plotting retrieved\nweather parameters"
                # "Matlab script goes online and retrieves most recent press, temp, and relative humidity data \nfrom the weather station on the roof of Cobleigh"
                # "Importing the current weather conditions from the COE weather station"
                n156 = disable-structure shown="Disabled" {
                  frame Disabled {
                    n157 = script code="%try\n%s=urlread('http://www.coe.montana.edu/ee/weather/mostCurrentCSV.php');\n%amin=textscan(s,'%s %s %s %s %s %s %s %s %s %s %s %s %s');\n%data=amin{1}{2};\n%[test remain]=strtok(data,',');\n%remain=str2num(remain);\n%press=remain(3)./1000;\n%temp=remain(5);\n%RH=remain(7);\n%catch\npress=.850;\ntemp=20;\nRH=40;\n%end"() -> ()  [unwired: 1 in, 4 out]
                  }
                  frame Enabled {
                  }
                }
                n158 = local read "WS_On/Off"() -> (w233:bool)
                n159 = case shown="True" w233 {
                  frame False {
                  }
                  frame True {
                    n160 = local read "WS visa"() -> (w238:refnum<visa-resource-name>)
                    n161 = call "T_RH_P.vi"("VISA in"=w238, "WS_Commands"=enum16{"OpenWS", "ReadTRHP", "CloseWS"}."ReadTRHP") -> ("TRHP"=w234:T13)  [unwired: 11 in, 2 out]
                    n162 = local write "TRHP"(w234) -> ()
                    n163 = Unbundle By Name(w234) -> ("Temp"=→"Temperature (C)":dbl, "RelH"=→"Relative Humdity (%)":dbl, "Press"=→"Pressure (mb)":dbl)
                  }
                }
              }
              frame #2 {
                # "Frame 3: Read, process, and plot online data\nFrame 4:\nFrame 5: Write the data to the folders from Frame 0 of outter sequence"
                # "Frame 0: Read the online wavelength and adjust to locking tolerance if out of range, Switch to offline DBR\nFrame 1: Read the output power from the Newport meter, calculate and plot the output pulse energy\nFrame 2: Wait 'Scalar Wait Time' for buffer to clear other wavelength data"
                # "Online"
                n164 = stacked-sequence {
                  frame #0 {
                    # "Read the online wavelength and continue adjusting the online DBR if outside the wavelength tolerance\nuntil it is within tolerance"
                    n165 = while {
                      i -> [w241]
                      stop <- w240 stop-if-true
                      # "Frame 2: Decrement DBR current if above tolerance\nFrame 3: Increment DBR current if below tolerance"
                      # "Frame 0: Read the current wavelength from the wavemeter\nFrame 1: Calculate the difference between desired and actual wavelength"
                      # "Continue reading and adjusting online DBR current until within locking tolerance"
                      n166 = stacked-sequence {
                        tunnel: w241 -> [w243 _ _ _ _]
                        tunnel: [_ _ w259 _ _] -> w240
                        frame #0 {
                          n167 = Equal To 0?(x=w243) -> (x = 0?=w242:bool)
                          n168 = case shown="True" w242 {
                            frame False {
                            }
                            frame True {
                              # "Set the wavemeter switch to WV Online"
                              n169 = flat-sequence {
                                frame #0 {
                                n170 = Build Array(FALSE ("Boolean")) -> (w246:bool[])
                                n171 = call-poly <vilib>:"DAQmx Write.vi"("task/channels in"=refnum<k21> "BristolWM", "data"=w246) -> ()  [unwired: 11 in, 3 out]
                                }
                                frame #1 {
                                n172 = Build Array(FALSE ("Boolean")) -> (w249:bool[])
                                n173 = call-poly <vilib>:"DAQmx Write.vi"("task/channels in"=refnum<k21> "HSRL_WV_switch", "data"=w249) -> ()  [unwired: 11 in, 3 out]
                                }
                              }
                            }
                          }
                        }
                        frame #1 {
                          # "Reading the wavelength from the wavemeter"
                          n174 = flat-sequence {
                            tunnel: [w252] -> w251
                            tunnel: w251 -> [w255]
                            tunnel: [w254] -> w250
                            tunnel: w250 -> [w258]
                            frame #0 {
                              n175 = local read "Bristol In"() -> (w253:i32)
                              n176 = dll-call lib="C:/Users/eol-lidar/Desktop/20171016_WVDIALLabviewSlimmed/DLLs/CLDevIface.dll" fn="CLOpenUSBSerialDevice"("commPort"=w253) -> ("return type"=w252:i32)  [unwired: 4 in, 2 out]
                            }
                            frame #1 {
                              n177 = dll-call lib="C:/Users/eol-lidar/Desktop/20171016_WVDIALLabviewSlimmed/DLLs/CLDevIface.dll" fn="CLGetLambdaReading"("devHandle"=w255) -> ("return type"=→"WV Online Read (nm)":dbl, "devHandle"=w254:i32)  [unwired: 3 in, 2 out]
                            }
                            frame #2 {
                              n178 = dll-call lib="C:/Users/eol-lidar/Desktop/20171016_WVDIALLabviewSlimmed/DLLs/CLDevIface.dll" fn="CLCloseDevice"("commPort"=w258) -> ("return type"=w257:i32)  [unwired: 4 in, 2 out]
                              n179 = local write "Bristol Out"(w257) -> ()
                            }
                          }
                        }
                        frame #2 {
                          # "If WL difference is within tolerance, stop looping, and illuminate 'Wavelength Lock Online' indicator"
                          # "Calculating the difference between the actual and desired online wavelength"
                          n180 = local read "WV Online Read (nm)"() -> (w262:dbl)
                          n181 = local read "Online_Tol"() -> (w267:dbl)
                          n182 = Multiply(x=-1.0, y=w267) -> (x*y=w268:dbl)
                          n183 = Subtract(x=w262, y="WV Online Set (nm)") -> (x-y=w263:dbl)
                          "Online_Diff" <- w263
                          n184 = Greater?(x=w263, y=w268) -> (0:w264:bool)
                          n185 = Less?(x=w263, y=w267) -> (x < y?=w265:bool)
                          n186 = And(x=w264, y=w265) -> (x .and. y?=w261:bool)
                          "WV Online Locked" <- w261
                          n187 = Or(x=w261, y="Cancel online") -> (x .or. y?=w259:bool)
                        }
                        frame #3 {
                          # "If the wavelength difference is greater that 0.0002 nm, decrement the \nDBR current by 0.01 mA"
                          n188 = local read "Online_Diff"() -> (w272:dbl)
                          n189 = Greater Or Equal?(x=w272, y="Online_Tol") -> (x >= y?=w271:bool)
                          n190 = case shown="True" w271 {
                            frame False {
                              # "Wavelength difference is not greater than 0.0002 nm, do nothing"
                            }
                            frame True {
                              # "Generating a command string\nto decrement the current"
                              # "WL difference is greater than 0.0002 nm,\ndecrement the DBR current by 0.01 mA"
                              n191 = local read "Settings"() -> (w279:T6)
                              n192 = local read "temp step size"() -> (w274:dbl)
                              n193 = Unbundle By Name(w279) -> ("WV Online TEC"=w278:dbl)
                              n194 = local read "Device In"() -> (w275:refnum<visa-resource-name>)
                              n195 = Subtract(x=w278, y=w274) -> (x-y=w277:dbl)
                              n196 = Bundle By Name(cluster=w279, "WV Online TEC"=w277, "Module"=T12."WV Online TEC") -> (w281:T6)
                              n197 = call "TL_Driver_v2.vi"("Device In"=w275, "Commands"=T9."SET", "Settings"=w281) -> ("Readings"=w280:T7)  [unwired: 9 in, 3 out]
                              n198 = local write "Settings"(w281) -> ()
                              n199 = local write "Readings"(w280) -> ()
                            }
                          }
                        }
                        frame #4 {
                          # "If WL difference is < 0.0002 nm, increment the DBR current"
                          n200 = local read "Online_Tol"() -> (w283:dbl)
                          n201 = local read "Online_Diff"() -> (w286:dbl)
                          n202 = Multiply(x=-1.0, y=w283) -> (x*y=w282:dbl)
                          n203 = Less Or Equal?(x=w286, y=w282) -> (x <= y?=w285:bool)
                          n204 = case shown="True" w285 {
                            frame False {
                              # "WL difference is no <= to -0.0002 nm, do nothing"
                            }
                            frame True {
                              # "WL difference is < -0.0002,\nincrement the DBR current by 0.01 mA"
                              # "Generating a command string\nto decrement the current"
                              n205 = local read "Settings"() -> (w295:T6)
                              n206 = local read "temp step size"() -> (w288:dbl)
                              n207 = Unbundle By Name(w295) -> ("WV Online TEC"=w292:dbl)
                              n208 = local read "Device In"() -> (w289:refnum<visa-resource-name>)
                              n209 = Add(x=w292, y=w288) -> (x+y=w291:dbl)
                              n210 = Bundle By Name(cluster=w295, "WV Online TEC"=w291, "Module"=T12."WV Online TEC") -> (w294:T6)
                              n211 = call "TL_Driver_v2.vi"("Device In"=w289, "Commands"=T9."SET", "Settings"=w294) -> ("Readings"=w293:T7)  [unwired: 9 in, 3 out]
                              n212 = local write "Settings"(w294) -> ()
                              n213 = local write "Readings"(w293) -> ()
                            }
                          }
                        }
                      }
                    }
                  }
                  frame #1 {
                    # "Converting to pulse energy, assumes 5 percent pickoff"
                    # "Reading the Newport Power meter"
                    # "Reading the output power of the laser transmitter from the Newport power meter, once read, convert to corresponding pulse energy and plot"
                    n214 = local read "Newport Device Key"() -> (w300:string)
                    n215 = local read "NewportRef"() -> (w296:refnum<k24>)
                    n216 = disable-structure shown="Enabled" {
                      frame Enabled {
                        # "Plotting the online and offling pulse energies"
                        n217 = local read "Online Pulse Energy"() -> (w311:dbl)
                        n218 = local read "Offline Pulse Energy"() -> (w310:dbl)
                        n219 = Bundle("Online Pulse Energy"=w311, "Offline Pulse Energy"=w310) -> (→"Pulse Energy (Micro Joule)":T15)  [unwired: 1 in]
                      }
                      frame Disabled {
                      }
                    }
                    n220 = Number To Decimal String(number="SampleSize") -> (decimal integer string=w298:string)  [unwired: 1 in]
                    n221 = invoke class="PowerMeterCommands" method="PerformDAQ"(reference=w296, "deviceKey"=w300, "interval"="1", "sampleSize"=w298) -> ("PerformDAQ"=w301:dbl[])  [unwired: 2 in, 5 out]
                    n222 = call-poly <vilib>:"Mean.vi"("X"=w301) -> ("mean"=w299:dbl)  [unwired: 1 out]
                    n223 = Multiply(x=w299, y=1000.0) -> (x*y=w307:dbl)
                    n224 = Divide(x=w307, y=0.05) -> (x/y=w305:dbl)
                    n225 = Divide(x=w305, y=7.0) -> (x/y=→"Online Pulse Energy":dbl)
                  }
                  frame #2 {
                    # "Wait 'Scalar Wait Time' for the next available batch of scalar card data"
                    n226 = local read "AMCS_Profile"() -> (w312:i32)
                    n227 = disable-structure shown="Disabled" {
                      frame Disabled {
                        # "Waiting 'Scalar Wait Time'"
                        n228 = Wait (ms)(milliseconds to wait="Scalar Wait Time") -> ()  [unwired: 1 out]
                      }
                      frame Enabled {
                      }
                    }
                    n229 = while {
                      tunnel: [w319] -> w313
                      tunnel: [w315] -> _
                      tunnel: w312 -> [w315]
                      stop <- w317 stop-if-true
                      n230 = global read "AMCS_Data.vi" "AMCS_Profile"() -> (w319:i32)
                      n231 = Wait (ms)(milliseconds to wait=u32 10) -> ()  [unwired: 1 out]
                      n232 = Equal?(x=w319, y=w315) -> (x = y?=w318:bool)
                      n233 = case shown="False" w318 {
                        tunnel: [TRUE FALSE] -> w317
                        frame False {
                        }
                        frame True {
                        }
                      }
                    }
                    "AMCS_Profile" <- w313
                  }
                  frame #3 {
                    # "convert time per range bin to meters\nand calculate smoothed bins using\nsmoothing range"
                    # "Plotting online cross section and smoothed online data"
                    # "Calculate the bin by bin mean of the data"
                    # "Collect 'Integration Period (Seconds)' number\nof scalar data"
                    # "Reading, processing, and plotting the online data"
                    n234 = local read "Data Reads (number of loops)"() -> (w323:i32)
                    n235 = local read "bins"() -> (w322:u32)
                    n236 = for {
                      N: w323 -> [_]
                      tunnel: [w377] -> w363 mode=indexing
                      tunnel: [w372] -> w328 mode=indexing
                      tunnel: w322 -> [w371]
                      # "Scalar Data is retrieved from Global \nVariable that scaler.vi is writing to,"
                      n237 = global read "AMCS_Data.vi" "AMCS_Data"() -> (w380:u16[][])
                      n238 = disable-structure shown="Disabled" {
                        frame Disabled {
                          n239 = global read "Scalar_Data_3.vi" "Scalar Data 3"() -> ()  [unwired: 1 out]
                          n240 = global read "Scalar_Data.vi" "Scalar Data"() -> ()  [unwired: 1 out]
                        }
                        frame Enabled {
                        }
                      }
                      n241 = Index Array(array=w380, index (row) #1=0 ("index (row)"), index (row) #2=2 ("index (row)")) -> (element #1=w376:u16[], element #2=w374:u16[])  [unwired: 2 in]
                      n242 = Array Subset(array=w376, index=0, length=w371) -> (w377:u16[])
                      n243 = Array Subset(array=w374, index=0, length=w371) -> (w372:u16[])
                    }
                    n244 = Transpose 2D Array(2D array=w363) -> (transposed array=w367:u16[][])
                    n245 = Transpose 2D Array(2D array=w328) -> (transposed array=w350:u16[][])
                    n246 = for {
                      tunnel: w350 -> [w370] mode=indexing
                      tunnel: [w369] -> w351 mode=indexing
                      n247 = call-poly <vilib>:"Mean.vi"("X"=w370) -> ("mean"=w369:dbl)  [unwired: 1 out]
                    }
                    n248 = for {
                      tunnel: w367 -> [w382] mode=indexing
                      tunnel: [w381] -> w368 mode=indexing
                      n249 = call-poly <vilib>:"Mean.vi"("X"=w382) -> ("mean"=w381:dbl)  [unwired: 1 out]
                    }
                    n250 = Array Subset(array=w368, index=1 ("dimension size"), length=w322) -> (w355:dbl[])
                    n251 = Array Subset(array=w351, index=1 ("dimension size"), length=w322) -> (w348:dbl[])
                    n252 = local read "background length"() -> (w335:i32)
                    n253 = local read "background start"() -> (w336:u32)
                    n254 = Array Size(array=w355) -> (size(s)=w352:i32)
                    n255 = Array Size(array=w348) -> (size(s)=w345:i32)
                    n256 = Initialize Array(1.0 ("element"), w352) -> (w354:dbl[])
                    n257 = Initialize Array(1.0 ("element"), w345) -> (w347:dbl[])
                    n258 = Multiply(x=w355, y=w354) -> (x*y=w356:dbl[])
                    "CH 0 Bin Readings" <- w356
                    n259 = Multiply(x=w348, y=w347) -> (x*y=w339:dbl[])
                    "CH 2 Bin Readings" <- w339
                    n260 = local read "Total DIAL Integration Time (Minutes)"() -> (w359:i32)
                    n261 = local read "Total Aerosol Integration Time (Minutes)"() -> (w325:dbl)
                    n262 = local read "Time Resolution Per Bin(ns)"() -> (w331:u32)
                    n263 = Array Subset(array=w356, index=w336, length=w335) -> (w365:dbl[])
                    n264 = Array Subset(array=w339, index=w336, length=w335) -> (w341:dbl[])
                    n265 = Divide(x=w325, y=w323) -> (x/y=w326:dbl)
                    n266 = call-poly <vilib>:"Mean.vi"("X"=w365) -> ("mean"=w364:dbl)  [unwired: 1 out]
                    n267 = Multiply(x=w326, y=60.0) -> (x*y=w324:dbl)
                    n268 = call-poly <vilib>:"Mean.vi"("X"=w341) -> ("mean"=w342:dbl)  [unwired: 1 out]
                    n269 = Divide(x=w359, y=w323) -> (x/y=w357:dbl)
                    n270 = local read "Index"() -> (w340:i32)
                    n271 = Subtract(x=w356, y=w364) -> (x-y=w361:dbl[])
                    n272 = Subtract(x=w339, y=w342) -> (x-y=w343:dbl[])
                    n273 = Multiply(x=w357, y=60.0) -> (x*y=w337:dbl)
                    n274 = To Double Precision Float(number=w331) -> (double precision float=w332:dbl)
                    n275 = Multiply(x=w332, y=0.15) -> (x*y=w334:dbl)
                    n276 = call "Ring Buffer CH2 rev2.vi"("Index"=w340, "Profiles to Average"=w324, "Input Array"=w343) -> ("AvgArray"=w344:dbl[])  [unwired: 7 in, 1 out]
                    n277 = call "Ring Buffer CH0 rev2.vi"("Index"=w340, "Profiles to Average"=w337, "Input Array"=w361) -> ("AvgArray"=w360:dbl[])  [unwired: 7 in, 1 out]
                    n278 = Divide(x="Smoothing Range", y=w334) -> (x/y=w329:dbl)
                    "Smoothed Bins" <- w329
                    n279 = call "Smooth Arrray.vi"("smooth size"=w329, "Raw Array"=w360) -> ("Smoothed Array"=→"CH0 (WV on) smoothed":dbl[])  [unwired: 9 in]
                    n280 = call "Smooth Arrray.vi"("smooth size"=w329, "Raw Array"=w344) -> ("Smoothed Array"=→"CH2 (molecular) smoothed":dbl[])  [unwired: 9 in]
                    n281 = disable-structure shown="Disabled" {
                      frame Disabled {
                        n282 = script code="format long;\ncounts=sum(Online);\nif counts >=0.5e6\ntime=time;\nelse\ntime=time\nend"() -> ()  [unwired: 3 in, 2 out]
                      }
                      frame Enabled {
                      }
                    }
                  }
                  frame #4 {
                    # "Toggling the Agiltron switch to the offline DBR seed laser"
                    n283 = disable-structure shown="Disabled" {
                      frame Disabled {
                        n284 = flat-sequence {
                          frame #0 {
                            # "Second one"
                            # "Command the switch to switch to position 2\ncorresponding to the offline DBR"
                            # "Hex string command \ncorrespond to offline"
                            n285 = VISA Write(VISA resource name="Switch Comm Port", write buffer="\u0001\u0012\u0000\u0001") -> ()  [unwired: 1 in, 3 out]
                          }
                        }
                      }
                      frame Enabled {
                      }
                    }
                  }
                  frame #5 {
                    # "Save the recently collected online data if 'Save Data?' is true"
                    n286 = case shown="True" "Save Data?" {
                      frame False {
                        # "'Save Data?' is false, do nothing"
                      }
                      frame True {
                        # "'Save Data?' is true, save onfline data to the Data Disk"
                        # "Write only one copy of data at this time"
                        # "Retrieve Julian Date"
                        n287 = local read "Readings"() -> (w388:T7)
                        n288 = local read "Time Resolution Per Bin(ns)"() -> (w396:u32)
                        n289 = Unbundle By Name(w388) -> ("WV OnLine TEC"=w387:dbl)
                        n290 = local read "Number of Accumulates"() -> (w394:u32)
                        n291 = Unbundle By Name(w388) -> ("HSRL TEC"=w386:dbl)
                        n292 = local read "WV Online Read (nm)"() -> (w389:dbl)
                        n293 = local write "DataOpen"(TRUE ("DataOpen")) -> ()
                        n294 = local read "Number of Bins"() -> (w395:u32)
                        n295 = local read "HSRL Read (nm)"() -> (w390:dbl)
                        n296 = local read "Online Pulse Energy"() -> (w417:dbl)
                        n297 = local read "CH 0 Bin Readings"() -> (w419:dbl[])
                        n298 = To Double Precision Float(number=w396) -> (double precision float=w391:dbl)
                        n299 = To Double Precision Float(number=w395) -> (double precision float=w392:dbl)
                        n300 = To Double Precision Float(number=w394) -> (double precision float=w393:dbl)
                        n301 = local read "CH 2 Bin Readings"() -> (w416:dbl[])
                        n302 = call "Julian_Date_2.vi"() -> ("Julian Date"=w418:dbl)  [unwired: 11 in]
                        n303 = Build Array (concatenate)(w418, w389, w387, w417, w391, w392, w393, w419) -> (w411:dbl[])
                        n304 = Build Array (concatenate)(w418, w390, w386, w417, w391, w392, w393, w416) -> (w401:dbl[])
                        n305 = local read "NF_On_Ref"() -> (w399:refnum<file>)
                        n306 = local read "FF_On_Ref"() -> (w415:refnum<file>)
                        n307 = local read "NF_On_Ptr"() -> (w400:i64)
                        n308 = local read "FF_On_Ptr"() -> (w414:i64)
                        n309 = Set File Position(offset (in bytes) (0)=w414, refnum=w415) -> (refnum out=w412:refnum<file>, error out=w409:errorcluster)  [unwired: 2 in]
                        n310 = Set File Position(offset (in bytes) (0)=w400, refnum=w399) -> (refnum out=w405:refnum<file>, error out=w403:errorcluster)  [unwired: 2 in]
                        n311 = Write to Binary File(file (use dialog)=w405, data=w401, error in=w403, 5:FALSE ("prepend array or string size? (T)")) -> (refnum out=w404:refnum<file>, error out=w402:errorcluster)  [unwired: 2 in, 1 out]
                        n312 = Write to Binary File(file (use dialog)=w412, data=w411, error in=w409, 5:FALSE ("prepend array or string size? (T)")) -> (refnum out=w410:refnum<file>, error out=w408:errorcluster)  [unwired: 2 in, 1 out]
                        n313 = Get File Position(4:w402, 7:w404) -> (2:w398:i64)  [unwired: 2 out]
                        n314 = Get File Position(4:w408, 7:w410) -> (2:w407:i64)  [unwired: 2 out]
                        n315 = local write "NF_On_Ptr"(w398) -> ()
                        n316 = local write "FF_On_Ptr"(w407) -> ()
                      }
                    }
                  }
                }
              }
              frame #3 {
                # "Frame 3: Read offline data, calculate aerosol data, and plot offline and normalized relative backscatter\nFrame 4:\nFrame 5: Save the offline data and related information"
                # "Frame 0: Read the offline wavelength and lock if necessary, Switch to online DBR\nFrame 1: Read the output power from the Newport power meter\nFrame 2: Wait 'Scalar Wait Time' for buffers to clear of online contiminated data"
                # "offline"
                n317 = stacked-sequence {
                  frame #0 {
                    # "Following Locking the Offline wavelength, check and lock the HSRL 780 nm wavelength"
                    # "Every 60 data collection cycles, read the offline DBR wavelength, and if outside of wavelength tolerance, adjust DBR current until within tolerance"
                    n318 = local read "L_Count"() -> (w421:i32)
                    n319 = Quotient & Remainder(x=w421, y=60.0) -> (x-y*floor(x/y)=w422:dbl)  [unwired: 1 out]
                    n320 = Equal To 0?(x=w422) -> (x = 0?=w420:bool)
                    n321 = case shown="True" w420 {
                      frame False {
                      }
                      frame True {
                        n322 = flat-sequence {
                          frame #0 {
                            n323 = while {
                              i -> [w427]
                              stop <- w425 stop-if-true
                              # "If WL difference is within tolerance, stop looping, and illuminate 'Wavelength Lock Offline' indicator"
                              # "Frame 2: Decrement DBR if above tolerance\nFrame 3: Increment DBR if below tolerance"
                              # "Frame 0: Read the wavelength from the wavemeter\nFrame 1: Calculate the difference between desired and actual wavelength"
                              # "Continue reading and adjusting offline DBR until within locking tolerance"
                              n324 = stacked-sequence {
                                tunnel: w427 -> [w429 _ _ _ _]
                                tunnel: [_ _ w443 _ _] -> w424
                                frame #0 {
                                n325 = Equal To 0?(x=w429) -> (x = 0?=w428:bool)
                                n326 = case shown="True" w428 {
                                frame False {
                                }
                                frame True {
                                # "Set the TSOA switch to\namplify the offline wavelength"
                                n327 = Build Array(TRUE ("Boolean")) -> (w431:bool[])
                                n328 = call-poly <vilib>:"DAQmx Write.vi"("task/channels in"=refnum<k21> "BristolWM", "data"=w431) -> ()  [unwired: 11 in, 3 out]
                                n329 = Wait (ms)(milliseconds to wait=u32 3200) -> ()  [unwired: 1 out]
                                }
                                }
                                }
                                frame #1 {
                                # "Reading the wavelength from the wavemeter"
                                n330 = flat-sequence {
                                tunnel: [w436] -> w435
                                tunnel: w435 -> [w439]
                                tunnel: [w438] -> w434
                                tunnel: w434 -> [w442]
                                frame #0 {
                                n331 = local read "Bristol In"() -> (w437:i32)
                                n332 = dll-call lib="C:/Users/eol-lidar/Desktop/20171016_WVDIALLabviewSlimmed/DLLs/CLDevIface.dll" fn="CLOpenUSBSerialDevice"("commPort"=w437) -> ("return type"=w436:i32)  [unwired: 4 in, 2 out]
                                }
                                frame #1 {
                                n333 = dll-call lib="C:/Users/eol-lidar/Desktop/20171016_WVDIALLabviewSlimmed/DLLs/CLDevIface.dll" fn="CLGetLambdaReading"("devHandle"=w439) -> ("return type"=→"WV Offline Read (nm)":dbl, "devHandle"=w438:i32)  [unwired: 3 in, 2 out]
                                }
                                frame #2 {
                                n334 = dll-call lib="C:/Users/eol-lidar/Desktop/20171016_WVDIALLabviewSlimmed/DLLs/CLDevIface.dll" fn="CLCloseDevice"("commPort"=w442) -> ("return type"=w441:i32)  [unwired: 4 in, 2 out]
                                n335 = local write "Bristol Out"(w441) -> ()
                                }
                                }
                                }
                                frame #2 {
                                # "Calculating the difference between the actual and desired online wavelength"
                                n336 = local read "Offline_Tol"() -> (w445:dbl)
                                n337 = local read "WV Offline Read (nm)"() -> (w451:dbl)
                                n338 = Multiply(x=-1.0, y=w445) -> (x*y=w444:dbl)
                                n339 = Subtract(x=w451, y="WV Offline Set (nm)") -> (x-y=w447:dbl)
                                "Oflline_Diff" <- w447
                                n340 = Greater?(x=w447, y=w444) -> (0:w448:bool)
                                n341 = Less?(x=w447, y=w445) -> (x < y?=w449:bool)
                                n342 = And(x=w448, y=w449) -> (x .and. y?=w443:bool)
                                "WV Oflline Locked" <- w443
                                n343 = case shown="True" w443 {
                                frame False {
                                }
                                frame True {
                                # "Set the Wavemeter switch to\nthe HSRL wavelength"
                                n344 = Build Array(TRUE ("Boolean")) -> (w453:bool[])
                                n345 = call-poly <vilib>:"DAQmx Write.vi"("task/channels in"=refnum<k21> "HSRL_WV_switch", "data"=w453) -> ()  [unwired: 11 in, 3 out]
                                n346 = Wait (ms)(milliseconds to wait=u32 3200) -> ()  [unwired: 1 out]
                                }
                                }
                                }
                                frame #3 {
                                # "If the wavelength difference is greater that 0.0002 nm, decrement the \nDBR current by 0.01 mA"
                                n347 = local read "Oflline_Diff"() -> (w458:dbl)
                                n348 = Greater Or Equal?(x=w458, y="Offline_Tol") -> (x >= y?=w457:bool)
                                n349 = case shown="True" w457 {
                                frame False {
                                # "Wavelength difference is not greater than 0.0002 nm, do nothing"
                                }
                                frame True {
                                # "Generating a command string\nto decrement the current"
                                n350 = local read "Settings"() -> (w465:T6)
                                n351 = Unbundle By Name(w465) -> ("WV Offline TEC"=w463:dbl)
                                n352 = Subtract(x=w463, y="temp step size") -> (x-y=w462:dbl)
                                n353 = local read "Device In"() -> (w460:refnum<visa-resource-name>)
                                n354 = Bundle By Name(cluster=w465, "WV Offline TEC"=w462, "Module"=T12."WV Offline TEC") -> (w466:T6)
                                n355 = call "TL_Driver_v2.vi"("Device In"=w460, "Commands"=T9."SET", "Settings"=w466) -> ("Readings"=w467:T7)  [unwired: 9 in, 3 out]
                                n356 = local write "Settings"(w466) -> ()
                                n357 = local write "Readings"(w467) -> ()
                                }
                                }
                                }
                                frame #4 {
                                # "If WL difference is < 0.0002 nm, increment the DBR temperature"
                                n358 = local read "Oflline_Diff"() -> (w470:dbl)
                                n359 = Less Or Equal?(x=w470, y=-0.0001) -> (x <= y?=w468:bool)
                                n360 = case shown="True" w468 {
                                frame False {
                                # "WL difference is no <= to -0.0002 nm, do nothing"
                                }
                                frame True {
                                # "Generating a command string\nto decrement the current"
                                # "WL difference is less than 0.0002 nm,\nincrement the DBR current by 0.01 mA"
                                n361 = local read "Settings"() -> (w478:T6)
                                n362 = Unbundle By Name(w478) -> ("WV Offline TEC"=w476:dbl)
                                n363 = local read "temp step size"() -> (w472:dbl)
                                n364 = Add(x=w476, y=w472) -> (x+y=w475:dbl)
                                n365 = local read "Device In"() -> (w473:refnum<visa-resource-name>)
                                n366 = Bundle By Name(cluster=w478, "WV Offline TEC"=w475, "Module"=T12."WV Offline TEC") -> (w479:T6)
                                n367 = call "TL_Driver_v2.vi"("Device In"=w473, "Commands"=T9."SET", "Settings"=w479) -> ("Readings"=w477:T7)  [unwired: 9 in, 3 out]
                                n368 = local write "Settings"(w479) -> ()
                                n369 = local write "Readings"(w477) -> ()
                                }
                                }
                                }
                              }
                              n370 = Or(x=w424, y="Cancel Offline") -> (x .or. y?=w425:bool)
                            }
                          }
                          frame #1 {
                            n371 = while {
                              i -> [w483]
                              stop <- w481 stop-if-true
                              # "If WL difference is within tolerance, stop looping, and illuminate 'Wavelength Lock Offline' indicator"
                              # "Frame 2: Decrement DBR if above tolerance\nFrame 3: Increment DBR if below tolerance"
                              # "Frame 0: Read the wavelength from the wavemeter\nFrame 1: Calculate the difference between desired and actual wavelength"
                              # "Continue reading and adjusting offline DBR until within locking tolerance"
                              n372 = stacked-sequence {
                                tunnel: w483 -> [w485 _ _ _ _]
                                tunnel: [_ _ w498 _ _] -> w480
                                frame #0 {
                                n373 = Equal To 0?(x=w485) -> (x = 0?=w484:bool)
                                n374 = case shown="True" w484 {
                                frame False {
                                }
                                frame True {
                                # "Set the Wavemeter to\nthe non HSRL wavelength"
                                n375 = Build Array(TRUE ("Boolean")) -> (w486:bool[])
                                n376 = call-poly <vilib>:"DAQmx Write.vi"("task/channels in"=refnum<k21> "HSRL_WV_switch", "data"=w486) -> ()  [unwired: 11 in, 3 out]
                                }
                                }
                                }
                                frame #1 {
                                # "Reading the wavelength from the wavemeter"
                                n377 = flat-sequence {
                                tunnel: [w491] -> w490
                                tunnel: w490 -> [w494]
                                tunnel: [w493] -> w489
                                tunnel: w489 -> [w497]
                                frame #0 {
                                n378 = local read "Bristol In"() -> (w492:i32)
                                n379 = dll-call lib="C:/Users/eol-lidar/Desktop/20171016_WVDIALLabviewSlimmed/DLLs/CLDevIface.dll" fn="CLOpenUSBSerialDevice"("commPort"=w492) -> ("return type"=w491:i32)  [unwired: 4 in, 2 out]
                                }
                                frame #1 {
                                n380 = dll-call lib="C:/Users/eol-lidar/Desktop/20171016_WVDIALLabviewSlimmed/DLLs/CLDevIface.dll" fn="CLGetLambdaReading"("devHandle"=w494) -> ("return type"=→"HSRL Read (nm)":dbl, "devHandle"=w493:i32)  [unwired: 3 in, 2 out]
                                }
                                frame #2 {
                                n381 = dll-call lib="C:/Users/eol-lidar/Desktop/20171016_WVDIALLabviewSlimmed/DLLs/CLDevIface.dll" fn="CLCloseDevice"("commPort"=w497) -> ("return type"=w496:i32)  [unwired: 4 in, 2 out]
                                n382 = local write "Bristol Out"(w496) -> ()
                                }
                                }
                                }
                                frame #2 {
                                # "Calculating the difference between the actual and desired online wavelength"
                                n383 = local read "HSRL_Tol"() -> (w500:dbl)
                                n384 = local read "HSRL Read (nm)"() -> (w506:dbl)
                                n385 = Multiply(x=-1.0, y=w500) -> (x*y=w499:dbl)
                                n386 = Subtract(x=w506, y="HSRL Set (nm)") -> (x-y=w502:dbl)
                                "HSRL_Diff" <- w502
                                n387 = Greater?(x=w502, y=w499) -> (0:w503:bool)
                                n388 = Less?(x=w502, y=w500) -> (x < y?=w504:bool)
                                n389 = And(x=w503, y=w504) -> (x .and. y?=w498:bool)
                                "HSRL Locked" <- w498
                                n390 = case shown="True" w498 {
                                frame False {
                                }
                                frame True {
                                # "Set the Wavementer switch to WV Online"
                                n391 = Build Array(FALSE ("Boolean")) -> (w508:bool[])
                                n392 = Build Array(FALSE ("Boolean")) -> (w512:bool[])
                                n393 = call-poly <vilib>:"DAQmx Write.vi"("task/channels in"=refnum<k21> "BristolWM", "data"=w512) -> ("error out"=w507:errorcluster)  [unwired: 11 in, 2 out]
                                n394 = call-poly <vilib>:"DAQmx Write.vi"("task/channels in"=refnum<k21> "HSRL_WV_switch", "data"=w508, "error in"=w507) -> ()  [unwired: 10 in, 3 out]
                                n395 = Wait (ms)(milliseconds to wait=u32 3200) -> ()  [unwired: 1 out]
                                }
                                }
                                }
                                frame #3 {
                                # "If the wavelength difference is greater that 0.0002 nm, decrement the \nDBR current by 0.01 mA"
                                n396 = local read "HSRL_Diff"() -> (w517:dbl)
                                n397 = Greater Or Equal?(x=w517, y="HSRL_Tol") -> (x >= y?=w516:bool)
                                n398 = case shown="True" w516 {
                                frame False {
                                # "Wavelength difference is not greater than 0.0002 nm, do nothing"
                                }
                                frame True {
                                # "Generating a command string\nto decrement the current"
                                n399 = local read "Settings"() -> (w524:T6)
                                n400 = local read "temp step size"() -> (w518:dbl)
                                n401 = Unbundle By Name(w524) -> ("HSRL TEC"=w523:dbl)
                                n402 = Subtract(x=w523, y=w518) -> (x-y=w522:dbl)
                                n403 = local read "Device In"() -> (w520:refnum<visa-resource-name>)
                                n404 = Bundle By Name(cluster=w524, "HSRL TEC"=w522, "Module"=T12."HSRL TEC") -> (w525:T6)
                                n405 = call "TL_Driver_v2.vi"("Device In"=w520, "Commands"=T9."SET", "Settings"=w525) -> ("Readings"=w526:T7)  [unwired: 9 in, 3 out]
                                n406 = local write "Settings"(w525) -> ()
                                n407 = local write "Readings"(w526) -> ()
                                }
                                }
                                }
                                frame #4 {
                                # "If WL difference is < 0.0002 nm, increment the DBR temperature"
                                n408 = local read "HSRL_Diff"() -> (w529:dbl)
                                n409 = Less Or Equal?(x=w529, y=-0.0001) -> (x <= y?=w527:bool)
                                n410 = case shown="True" w527 {
                                frame False {
                                # "WL difference is no <= to -0.0002 nm, do nothing"
                                }
                                frame True {
                                # "Generating a command string\nto decrement the current"
                                # "WL difference is less than 0.0002 nm,\nincrement the DBR current by 0.01 mA"
                                n411 = local read "Settings"() -> (w537:T6)
                                n412 = local read "temp step size"() -> (w530:dbl)
                                n413 = Unbundle By Name(w537) -> ("HSRL TEC"=w535:dbl)
                                n414 = Add(x=w535, y=w530) -> (x+y=w534:dbl)
                                n415 = local read "Device In"() -> (w532:refnum<visa-resource-name>)
                                n416 = Bundle By Name(cluster=w537, "HSRL TEC"=w534, "Module"=T12."HSRL TEC") -> (w538:T6)
                                n417 = call "TL_Driver_v2.vi"("Device In"=w532, "Commands"=T9."SET", "Settings"=w538) -> ("Readings"=w536:T7)  [unwired: 9 in, 3 out]
                                n418 = local write "Settings"(w538) -> ()
                                n419 = local write "Readings"(w536) -> ()
                                }
                                }
                                }
                              }
                              n420 = Or(x=w480, y="Cancel HSRL") -> (x .or. y?=w481:bool)
                            }
                          }
                        }
                      }
                    }
                  }
                  frame #1 {
                    # "Reading the power meter"
                    # "Updating the pulse energy plot"
                    # "Converting to pulse energy"
                    # "Reading the offline output power, converting to pulse energy,  and updating the Pulse energy plot"
                    n421 = local read "SampleSize"() -> (w541:i32)
                    n422 = local read "Newport Device Key"() -> (w542:string)
                    n423 = local read "Online Pulse Energy"() -> (w548:dbl)
                    n424 = local read "Offline Pulse Energy"() -> (w547:dbl)
                    n425 = local read "NewportRef"() -> (w539:refnum<k24>)
                    n426 = Number To Decimal String(number=w541) -> (decimal integer string=w543:string)  [unwired: 1 in]
                    n427 = invoke class="PowerMeterCommands" method="PerformDAQ"(reference=w539, "deviceKey"=w542, "interval"="1", "sampleSize"=w543) -> ("PerformDAQ"=w544:dbl[])  [unwired: 2 in, 5 out]
                    n428 = Bundle("Online Pulse Energy"=w548, "Offline Pulse Energy"=w547) -> (w546:T15)  [unwired: 1 in]
                    n429 = local write "Pulse Energy (Micro Joule)"(w546) -> ()
                    n430 = call-poly <vilib>:"Mean.vi"("X"=w544) -> ("mean"=w540:dbl)  [unwired: 1 out]
                    n431 = Multiply(x=w540, y=1000.0) -> (x*y=w553:dbl)
                    n432 = Divide(x=w553, y=0.05) -> (x/y=w551:dbl)
                    n433 = Divide(x=w551, y=7.0) -> (x/y=→"Offline Pulse Energy":dbl)
                  }
                  frame #2 {
                    # "Added in the ability to interactively control the ThorLab  setting (just etalon temp for now)"
                    # "Wait 'Scalar Wait Time' for buffers to clear of online contiminated offline data"
                    n434 = disable-structure shown="Disabled" {
                      frame Disabled {
                        # "Wait 'Scalar Wait Time'"
                        n435 = local read "Scalar Wait Time"() -> (w570:u32)
                        n436 = Wait (ms)(milliseconds to wait=w570) -> ()  [unwired: 1 out]
                      }
                      frame Enabled {
                      }
                    }
                    n437 = event shown="[2] \"Settings.HSRL Etalon TEC\": Value Change" {
                      selector: _ -> [_ _ _]
                      dyn-events: _ -> [_ _ _]
                      timeout: 1 -> [_ _ _]
                      event Timeout {
                        n438 = event-data() -> ()  [unwired: 1 in, 2 out]
                      }
                      event "Settings.WV Etalon TEC": Value Change {
                        # "Generating a command string\nto update the etalon"
                        n439 = event-data() -> ()  [unwired: 1 in, 5 out]
                        n440 = local read "Settings"() -> (w560:T6)
                        n441 = Unbundle By Name(w560) -> ("WV Etalon TEC"=w562:dbl)
                        n442 = local read "Device In"() -> (w556:refnum<visa-resource-name>)
                        n443 = Bundle By Name(cluster=w560, "WV Etalon TEC"=w562, "Module"=T12."WV Etalon TEC") -> (w558:T6)
                        n444 = call "TL_Driver_v2.vi"("Device In"=w556, "Commands"=T9."SET", "Settings"=w558) -> ("Readings"=w559:T7)  [unwired: 9 in, 3 out]
                        n445 = local write "Readings"(w559) -> ()
                        n446 = local write "Settings"(w558) -> ()
                      }
                      event "Settings.HSRL Etalon TEC": Value Change {
                        # "Generating a command string\nto update the etalon"
                        n447 = event-data() -> ()  [unwired: 1 in, 5 out]
                        n448 = local read "Settings"() -> (w567:T6)
                        n449 = Unbundle By Name(w567) -> ("HSRL Etalon TEC"=w569:dbl)
                        n450 = local read "Device In"() -> (w563:refnum<visa-resource-name>)
                        n451 = Bundle By Name(cluster=w567, "HSRL Etalon TEC"=w569, "Module"=T12."HSRL Etalon TEC") -> (w565:T6)
                        n452 = call "TL_Driver_v2.vi"("Device In"=w563, "Commands"=T9."SET", "Settings"=w565) -> ("Readings"=w566:T7)  [unwired: 9 in, 3 out]
                        n453 = local write "Readings"(w566) -> ()
                        n454 = local write "Settings"(w565) -> ()
                      }
                    }
                  }
                  frame #3 {
                    w587 = 1
                    w616 = 1 ("dimension size")
                    # "Plotting the normalized relative \nbackscatter"
                    # "Calculating the normalized relative backscatter"
                    # "File path in MATLAB script is of old dial is:\nF:\\Micropulse DIAL\\Micropulse DIAL Matlab\\\nFinal Overlap Function.mat')];"
                    # "Read in latest scalar card data from \n'Scalar Data' global variable that \nscaler.vi is writing to, then wait 1 sec\nfor next batch of data"
                    # "Calculating/Plotting smoothed data,\ncross sections etc."
                    # "Pick off data with\nout header"
                    # "Calculate mean bin by bin mean"
                    # "Reading in 'Integration Period (Seconds)' of data"
                    # "Read the offline data from the scalar card, perform smoothing, calculate normalized relative backscatter, and plot"
                    # "Collects Data From Card,\nSends It To The Chart,\nAnd Saves A Copy As A\nFile If Option Selected On\nFront Panel"
                    n455 = local read "Total DIAL Integration Time (Minutes)"() -> (w632:i32)
                    n456 = local read "bins"() -> (w571:u32)
                    n457 = for {
                      N: "Data Reads (number of loops)" -> [_]
                      tunnel: [w644] -> w607 mode=indexing
                      tunnel: [w640] -> w606 mode=indexing
                      tunnel: w571 -> [w641]
                      n458 = global read "AMCS_Data.vi" "AMCS_Data"() -> (w647:u16[][])
                      n459 = disable-structure shown="Disabled" {
                        frame Disabled {
                          n460 = global read "Scalar_Data_4.vi" "Scalar Data 4"() -> ()  [unwired: 1 out]
                          n461 = global read "Scalar_Data_2.vi" "Scalar Data 2"() -> ()  [unwired: 1 out]
                        }
                        frame Enabled {
                        }
                      }
                      n462 = Index Array(array=w647, index (row) #1=1 ("index (row)"), index (row) #2=3 ("index (row)")) -> (element #1=w646:u16[], element #2=w643:u16[])  [unwired: 2 in]
                      n463 = Array Subset(array=w643, index=0, length=w641) -> (w640:u16[])
                      n464 = Array Subset(array=w646, index=0, length=w641) -> (w644:u16[])
                    }
                    n465 = Divide(x=w632, y="Data Reads (number of loops)") -> (x/y=w630:dbl)
                    n466 = local read "Total Aerosol Integration Time (Minutes)"() -> (w633:dbl)
                    n467 = Multiply(x=w630, y=60.0) -> (x*y=w620:dbl)
                    n468 = local read "background length"() -> (w611:i32)
                    n469 = local read "background start"() -> (w612:u32)
                    n470 = Transpose 2D Array(2D array=w607) -> (transposed array=w638:u16[][])
                    n471 = Transpose 2D Array(2D array=w606) -> (transposed array=w625:u16[][])
                    n472 = Divide(x=w633, y="Data Reads (number of loops)") -> (x/y=w634:dbl)
                    n473 = for {
                      N: w571 -> [_]
                      tunnel: w638 -> [w653] mode=indexing
                      tunnel: [w652] -> w639 mode=indexing
                      tunnel: w625 -> [w651] mode=indexing
                      tunnel: [w650] -> _ mode=indexing
                      tunnel: [w650] -> w622 mode=indexing
                      n474 = call-poly <vilib>:"Mean.vi"("X"=w653) -> ("mean"=w652:dbl)  [unwired: 1 out]
                      n475 = call-poly <vilib>:"Mean.vi"("X"=w651) -> ("mean"=w650:dbl)  [unwired: 1 out]
                    }
                    n476 = Multiply(x=w634, y=60.0) -> (x*y=w603:dbl)
                    n477 = Array Subset(array=w622, index=w616, length=w571) -> (w623:dbl[])
                    "CH3 Bin Readings" <- w623
                    n478 = Array Subset(array=w639, index=w616, length=w571) -> (w621:dbl[])
                    "CH1  Bin Readings" <- w621
                    n479 = Array Subset(array=w623, index=w612, length=w611) -> (w624:dbl[])
                    n480 = Array Subset(array=w621, index=w612, length=w611) -> (w637:dbl[])
                    n481 = local read "Smoothed Bins"() -> (w608:dbl)
                    n482 = call-poly <vilib>:"Mean.vi"("X"=w624) -> ("mean"=w593:dbl)  [unwired: 1 out]
                    n483 = call-poly <vilib>:"Mean.vi"("X"=w637) -> ("mean"=w598:dbl)  [unwired: 1 out]
                    n484 = local read "Index"() -> (w604:i32)
                    n485 = Subtract(x=w623, y=w593) -> (x-y=w605:dbl[])
                    n486 = Subtract(x=w621, y=w598) -> (x-y=w619:dbl[])
                    n487 = call "Ring Buffer CH1 short rev2.vi"("Index"=w604, "Profiles to Average"=w620, "Input Array"=w619) -> ("AvgArray"=w636:dbl[], "RingBufferOut"=→"CH1 RingBuffer long":dbl[][])  [unwired: 7 in]
                    n488 = call "Ring Buffer CH3 short rev2.vi"("Index"=w604, "Profiles to Average"=w603, "Input Array"=w605) -> ("AvgArray"=w614:dbl[], "RingBufferOut"=→"CH3 RingBuffer short":dbl[][])  [unwired: 7 in]
                    n489 = Reshape Array(w619, w616, w571) -> (→"CH 1 (WV off) counts display":dbl[][])
                    n490 = Reshape Array(w605, w616, w571) -> (→"CH 3 (HSRL comb) counts display":dbl[][])
                    n491 = local read "Time Resolution Per Bin(ns)"() -> (w594:u32)
                    n492 = local read "Number of Accumulates"() -> (w592:u32)
                    n493 = call "Smooth Arrray.vi"("smooth size"=w608, "Raw Array"=w636) -> ("Smoothed Array"=w572:dbl[])  [unwired: 9 in]
                    "CH1 (WV off) smooth" <- w572
                    n494 = call "Smooth Arrray.vi"("smooth size"=w608, "Raw Array"=w614) -> ("Smoothed Array"=w610:dbl[])  [unwired: 9 in]
                    "CH3 (HSRL combined) smooth" <- w610
                    n495 = local read "Temperature (C)"() -> (w629:dbl)
                    n496 = local read "Pressure (mb)"() -> (w628:dbl)
                    n497 = To Double Precision Float(number=w592) -> (double precision float=w591:dbl)
                    n498 = To Double Precision Float(number=w594) -> (double precision float=w590:dbl)
                    n499 = Reciprocal(x=w590) -> (1/x=w601:dbl)
                    n500 = script code="%accum_num=10000;     % scaler card setting number of accumulations\nt_bin = t_bin_in/1e9                 % scaler card setting time per bin\n%t_d = 37.3e-9;                % APD dead time from spec sheet\n\n% conversion from accumulated counts to count rate  (c/s)\nc_convert = 1./t_bin./accum_num;\nCR_WV = p_raw_WV.*c_convert;\nCR_HSRL = p_raw_HSRL.*c_convert;\nCR_total_WV = (p_raw_WV+b_WV).*c_convert;\nCR_total_HSRL = (p_raw_HSRL+b_HSRL).*c_convert;\nb_CR_WV =b_WV.*c_convert;\nb_CR_HSRL =b_HSRL.*c_convert;\n \n% create a range array\nsize_p =  size(p_raw_WV,2);\ngate = t_bin*3e8/2;\nr = (gate:gate:size_p*gate)./1e3; \n   \n%APD correction factor\n D_WV = 1./(1-(t_d*CR_total_WV));\n D_HSRL = 1./(1-(t_d*CR_total_HSRL));\n\n %Calculating normalize relative backscatter profile\n nrb_WV = CR_WV.*D_WV.*r.^2.*1e-6;\n nrb_HSRL = CR_HSRL.*D_HSRL.*r.^2.*1e-6;"("E"=6.0 ("Real"), "temp"=w629, "press"=w628, "p_raw_WV"=w572, "b_WV"=w598, "b_HSRL"=w593, "p_raw_HSRL"=w610, "accum_num"=w591, "t_d"="dead time", "t_bin_in"=w590) -> ("nrb_WV"=w580:cdb[], "D_WV"=w577:dbl[], "nrb_HSRL"=w579:cdb[], "D_HSRL"=w576:dbl[])  [unwired: 1 in, 1 out]
                    n501 = Divide(x=w601, y=w591) -> (x/y=w599:dbl)
                    n502 = Multiply(x=1000000000.0, y=w599) -> (x*y=w596:dbl)
                    n503 = Multiply(x=w596, y=w598) -> (x*y=w597:dbl)
                    n504 = Multiply(x=w596, y=w593) -> (x*y=w595:dbl)
                    n505 = Bundle(w597, w595) -> (→"?":cluster{dbl, dbl})  [unwired: 1 in]
                    n506 = local read "bins"() -> (w586:u32)
                    n507 = local read "Altitude Array (km)"() -> (w582:dbl[])
                    n508 = Build Array(w580, w579) -> (w584:cdb[][])
                    n509 = Build Array(w577, w576) -> (w575:dbl[][])
                    n510 = Reshape Array(w579, w587, w586) -> (→"NRB HSRL Combined":cdb[][])
                    n511 = Reshape Array(w580, w587, w586) -> (→"NRB WV Offline":cdb[][])
                    n512 = Build Array(w582, w582) -> (w581:dbl[][])
                    n513 = call "Convert to Dynamic Data7"("2D Array"=w575) -> ("Dynamic Data Type"=w574:dynamicdata)  [unwired: 3 in]
                    n514 = call "Convert to Dynamic Data3"("2D Array"=w584) -> ("Dynamic Data Type"=w583:dynamicdata)  [unwired: 3 in]
                    n515 = call "Convert to Dynamic Data4"("2D Array"=w581) -> ("Dynamic Data Type"=w578:dynamicdata)  [unwired: 3 in]
                    n516 = call "Build XY Graph2"("Y Input"=w578, "X Input"=w583) -> ("XY Graph"=→"NRB plot":cluster{"Y":dbl[], "Y":dbl[]}[])  [unwired: 3 in, 6 out]
                    n517 = call "Build XY Graph4"("Y Input"=w578, "X Input"=w574) -> ("XY Graph"=→"Correction":cluster{"Y":dbl[], "Y":dbl[]}[])  [unwired: 3 in, 6 out]
                  }
                  frame #4 {
                    # "REPLACE WITH NEW AGILTRON TASK!"
                    # "Toggle Agiltron switch to online DBR"
                    n518 = disable-structure shown="Disabled" {
                      frame Disabled {
                        # "ABSORBING"
                        n519 = flat-sequence {
                          frame #0 {
                            # "Third one"
                            # "Command the switch to switch to position 1\ncorresponding to the online DBR"
                            # "Hex string command \ncorrespond to online"
                            n520 = local read "Switch Comm Port"() -> (w657:refnum<visa-resource-name>)
                            n521 = VISA Write(VISA resource name=w657, write buffer="\u0001\u0012\u0000\u0002") -> ()  [unwired: 1 in, 3 out]
                          }
                        }
                        n522 = Build Array(FALSE ("Boolean")) -> (w656:bool[])
                        n523 = call-poly <vilib>:"DAQmx Write.vi"("task/channels in"=refnum<k21> "AgiltronSwitch", "data"=w656) -> ()  [unwired: 11 in, 3 out]
                      }
                      frame Enabled {
                      }
                    }
                  }
                  frame #5 {
                    # "If 'Save Data?' is true, save all relavant offline info"
                    n524 = local read "Save Data?"() -> (w659:bool)
                    n525 = case shown="True" w659 {
                      frame False {
                        # "'Save Data?' is false, do nothing"
                      }
                      frame True {
                        # "Write only one data file at this time"
                        # "Retrive Julian Date"
                        # "'Save Data?' is true, save offline data to the Data Disk"
                        n526 = local read "Readings"() -> (w660:T7)
                        n527 = Unbundle By Name(w660) -> ("WV Offline TEC"=w661:dbl)
                        n528 = Unbundle By Name(w660) -> ("HSRL TEC"=w662:dbl)
                        n529 = local read "HSRL Read (nm)"() -> (w663:dbl)
                        n530 = local read "WV Offline Read (nm)"() -> (w684:dbl)
                        n531 = local read "Relative Humdity (%)"() -> (w688:dbl)
                        n532 = local read "CH3 Bin Readings"() -> (w682:dbl[])
                        n533 = local read "CH1  Bin Readings"() -> (w689:dbl[])
                        n534 = local read "Offline Pulse Energy"() -> (w685:dbl)
                        n535 = local read "Temperature (C)"() -> (w686:dbl)
                        n536 = local read "Pressure (mb)"() -> (w687:dbl)
                        n537 = call "Julian_Date_2.vi"() -> ("Julian Date"=w683:dbl)  [unwired: 11 in]
                        n538 = Build Array (concatenate)(w683, w684, w661, w685, w686, w687, w688, w689) -> (w668:dbl[])
                        n539 = Build Array (concatenate)(w683, w663, w662, w685, w686, w687, w688, w682) -> (w665:dbl[])
                        n540 = local read "FF_Off_Ref"() -> (w670:refnum<file>)
                        n541 = local read "NF_Off_Ref"() -> (w667:refnum<file>)
                        n542 = local read "FF_Off_Ptr"() -> (w669:i64)
                        n543 = local read "NF_Off_Ptr"() -> (w666:i64)
                        n544 = Set File Position(offset (in bytes) (0)=w669, refnum=w670) -> (refnum out=w681:refnum<file>, error out=w679:errorcluster)  [unwired: 2 in]
                        n545 = Set File Position(offset (in bytes) (0)=w666, refnum=w667) -> (refnum out=w677:refnum<file>, error out=w675:errorcluster)  [unwired: 2 in]
                        n546 = Write to Binary File(file (use dialog)=w681, data=w668, error in=w679, 5:FALSE ("prepend array or string size? (T)")) -> (refnum out=w680:refnum<file>, error out=w678:errorcluster)  [unwired: 2 in, 1 out]
                        n547 = Write to Binary File(file (use dialog)=w677, data=w665, error in=w675, 5:FALSE ("prepend array or string size? (T)")) -> (refnum out=w676:refnum<file>, error out=w674:errorcluster)  [unwired: 2 in, 1 out]
                        n548 = Get File Position(4:w678, 7:w680) -> (2:w671:i64)  [unwired: 2 out]
                        n549 = Get File Position(4:w674, 7:w676) -> (2:w664:i64)  [unwired: 2 out]
                        n550 = local write "FF_Off_Ptr"(w671) -> ()
                        n551 = local write "NF_Off_Ptr"(w664) -> ()
                      }
                    }
                  }
                }
              }
              frame #4 {
                n552 = First Call?() -> (First Call?: T/F=w692:bool)
                n553 = Or(x="calculate absorption cross sections", y=w692) -> (x .or. y?=w690:bool)
                n554 = case shown="True" w690 {
                  frame False {
                  }
                  frame True {
                    # "calculate absorption cross sections from HITRAN data base"
                    n555 = local read "WV Offline Set (nm)"() -> (w696:dbl)
                    n556 = local read "WV Online Read (nm)"() -> (w699:dbl)
                    n557 = local read "CH1 (WV off) smooth"() -> (w700:dbl[])
                    n558 = local read "Temperature (C)"() -> (w698:dbl)
                    n559 = local read "Pressure (mb)"() -> (w697:dbl)
                    n560 = local read "gate size"() -> (w693:dbl)
                    n561 = script code="hitran = dlmread('C:\\Users\\eol-lidar\\Desktop\\20171016_WVDIALLabviewSlimmed\\HiranData\\815nm_841nm_HITRAN_2008.csv', ',',[1 1 1676 8]);\n\n%hitran = dlmread('C:\\Users\\H2ODial\\Desktop\\Shared Telescope WV DIAL Code\\Libraries and VIs\\815nm_841nm_HITRAN_2008.csv', ',',[1 1 1676 8]);\n%hitran = dlmread('C:\\Users\\H2ODial\\Desktop\\Shared Telescope WV DIAL Code\\Libraries and VIs\\824nm_841nm_H2O.csv', ',',[0 1 352 7]);\n%hitran = dlmread('C:\\Users\\H2ODial\\Desktop\\Shared Telescope WV DIAL Code\\Libraries and VIs\\824nm_841nm_H2O_Spectral_Calc.csv', ',',[1 1 1209 7]);\n\n%Range vector in meters\n%range = ([75:75:size(Online,2)*75]);\ntest = size(Online,2);\nrange = ([gate_size:gate_size:test.*gate_size]); \n\nif lambda< 828\nlambda=828.195;\nelse\nlambda=lambda;\nend;\n\n%%\n\n%Voigt profile calculation\nWNmin = 1/(828+4)*1e7;  % 832.0 nm converted to wavenumber\nWNmax = 1/(828-4)*1e7;  % 824.0 nm converted to wavenumber\n\n%Find lines from WNmin to WNmax to calculate voigt profile\nline_indices = hitran(1:size(hitran,1),1)>WNmin & hitran(1:size(hitran,1),1)<WNmax;\n\nline = double(hitran(line_indices, 1:size(hitran,2)));\n\n%Calculate temperature and pressure profile\nT0 = 273+25; % surface temperature\nT0 = 273+T0_C;\nT = T0-0.0065.*range; % set to match the sounding\n\n% pressure in atmospheres\nP0  = 0.83; % surface pressure\nP0  = P0_mb/1000*0.986; %pressure in mb converted to atm\nP = P0.*(T0./T).^-5.5;   % set this value to match sounding\n\nT00 = 296;              % HITRAN reference temperature [K]\nP00 = 1;                % HITRAN reference pressure [atm]\nnu0_0 = line(:,1);      % absorption line center wavenumber from HITRAN [cm^-1]\nS0 = line(:,2);         % initial linestrength from HITRAN [cm^-1/(mol*cm^-2)]   \ngammal0 = line(:,4);    % air-broadened halfwidth at T_ref and P_ref from HITRAN [cm^-1/atm]\ngamma_s = line(:,5);    % self-broadened halfwidth at T_ref and P_ref from HITRAN [cm^-1/atm]\nE = line(:,6);          % ground state transition energy from HITRAN [cm^-1]  \nalpha = line(:,7);      % linewidth temperature dependence factor from HITRAN\ndelta = line(:,8);      % pressure shift from HiTRAN [cm^-1 atm^-1]\nnu_on = 1/(lambda)*1e7;\nnu_off = 1/(lambda_off)*1e7;\n\nfor i = 1:size(Online,2); % calculate the absorption cross section at each range\n  \n    nu0 = nu0_0+delta.*(P(i)./P00); % unclear if it should be Pi/P00  \n    gammal = gammal0.*(P(i)./P00).*((T00./T(i)).^alpha);    %Calculate Lorentz lineweidth at P(i) and T(i)\n\n    const.m = 18.015E-3./6.022E23; % mass of a single water molecule\n    const.k_B = 1.3806488e-23; % (J/K)\n    const.c = 299792458; % (m/s) (exact)\n \n    gammad = (nu0).*((2.0.*const.k_B.*T(i).*log(2.0))./(const.m.*const.c^2)).^(0.5);  %Calculate HWHM Doppler linewidth at T(i)\n     \n    % term 1 in the Voigt profile\n    y = (gammal./gammad).*((log(2.0)).^(0.5));\n    \n    % term 2 in the Voigt profile\n    x_on = ((nu_on-nu0)./gammad).*(log(2.0)).^(0.5);\n    x_off = ((nu_off-nu0)./gammad).*(log(2.0)).^(0.5);\n    \n    %setting up Voigt convolution\n    t = (-(size(line,1))/2:1:size(line,1)/2-1); %set up the integration spectral step size\n    t = repmat(t',1,length(x_on))';\n    x_on = repmat(x_on,1,length(t));\n    x_off = repmat(x_off,1,length(t));\n    y = repmat(y,1,length(t));\n    f_on = (exp(-t.^2.0))./(y.^2.0+(x_on-t).^2.0);  % combined Voigt term 1 and 2\n    f_off = (exp(-t.^2.0))./(y.^2.0+(x_off-t).^2.0);\n    %Voigt integration over all of the lines at the on and offline locations\n    z_on = trapz(t(1,:),f_on,2);\n    z_off =  trapz(t(1,:),f_off,2);\n    integral_on = z_on;\n    integral_off = z_off;\n    %Calculate linestrength at temperature T\n    S = S0.*((T00./T(i)).^(1.5)).*exp(1.439.*E.*((1./T00)-(1./T(i))));\n \n    %Calculate the Voigt profile\n    K_on = (y(:,1)./pi).*integral_on;\n    K_off = (y(:,1)./pi).*integral_off;\n    \n    %Calculate the Voigt profile absorption cross section [cm^2]\n    sigmav_on = S.*(1./gammad).*(((log(2.0))./pi).^(0.5)).*K_on; %.*far_wing_on;\n    sigmav_off = S.*(1./gammad).*(((log(2.0))./pi).^(0.5)).*K_off; %.*far_wing_off;\n    \n    %Sum contributions from all of the surrounding lines\n    sigma_on_total(i) = sum(sigmav_on);\n    sigma_off_total(i) = sum(sigmav_off);\n    \nend;"("lambda"=w699, "lambda_off"=w696, "P0_mb"=w697, "T0_C"=w698, "Online"=w700, "gate_size"=w693) -> ("sigma_on_total"=→"sigma_on_total":dbl[], "sigma_off_total"=→"sigma_off_total":dbl[])  [unwired: 1 in, 1 out]
                  }
                }
              }
              frame #5 {
                # "normalization factor\nfrom 300 to 450m"
                # "OPTICAL DEPTH PLOT"
                # "Data Processing Far Channel"
                # "Calculating the range resolved water vapor number density and plotting"
                n562 = local read "gate size"() -> (w715:dbl)
                n563 = local read "CH3 (HSRL combined) smooth"() -> (w755:dbl[])
                n564 = local read "CH2 (molecular) smoothed"() -> (w754:dbl[])
                n565 = local read "CH0 (WV on) smoothed"() -> (w734:dbl[])
                n566 = local read "CH1 (WV off) smooth"() -> (w733:dbl[])
                n567 = local read "Temperature (C)"() -> (w713:dbl)
                n568 = local read "sigma_off_total"() -> (w757:dbl[])
                n569 = local read "sigma_on_total"() -> (w756:dbl[])
                n570 = local read "Pressure (mb)"() -> (w714:dbl)
                n571 = script code="backscatter_ratio = combined./molecular;\n\n% calculate the temp and pressure profiles from surface measurement\nT0 = 273+T0_C;\n% create a range array\n range = ([0:gate_size:(size(combined,2)-1)*gate_size]); \n T = T0-0.0065.*range; \n P0  = P0_mb/1000*0.986; %pressure in mb converted to atm\n P = P0.*(T0./T).^-5.5;   \n const.k_B = 1.363806488e-23; % (J/K)\n const.k_B = 1.363806488e-23*9.89*10^-6; % (atm m^3/K)\n% backscatter coefficient in m^-1 sr^-1\nbeta_m_profile = 5.45.*10^(-32).*(550/780.2)^4.*P./(T.*const.k_B);\n\nbeta_m_array = repmat(beta_m_profile, size(backscatter_ratio,1), 1);\nbeta_bs = ((backscatter_ratio.*receiver_scale_factor)-1).*beta_m_profile"("molecular"=w754, "combined"=w755, "gate_size"=w715, "T0_C"=w713, "P0_mb"=w714, "receiver_scale_factor"="Receiver Scale Factor") -> ("beta_bs"=w701:dbl[], "beta_m_profile"=w703:dbl[])  [unwired: 1 in, 2 out]
                n572 = script code="%Time averaging in seconds.  600 Seconds =10 minutes\ntemporal_average = 600;\n%Spatial averaging in bins.  150 meters\nspatial_average = 150./gate_size;\n%Creating r and r+deltar vectors..this can also be acsomplished using the diff command\np_oni = Online(:,1:size(Online,2)-1);\np_onii = Online(:,2:size(Online,2));\np_offi = Offline(:,1:size(Offline,2)-1);\np_offii = Offline(:,2:size(Offline,2));\nInside = (p_oni.*p_offii)./(p_onii.*p_offi);\ndel_cross = 1./(2.*(sigma_on_total(1:size(Online,2)-1)-sigma_off_total(1:size(Offline,2)-1)).*gate_size*100);\ndel_cross(isinf(del_cross)) = 0;\n%Calculating Number density\nN = del_cross.*log(Inside);\n%Spatial smoothing of the profiles\nfilter1 = ones(1,4)./4;\nN_1 = N;\nN_1_avg = filter2(filter1,N_1);\nfilter1 = ones(1,10)./10;\nN_2 = N;\nN_2_avg = filter2(filter1,N_2);\nN_new = zeros(size(N,1),size(N,2));\n%Using different averaging windows for different altitudes \nN_avg=[N_1_avg(:,1:40)';N_2_avg(:,41:size(N,2))']';\nw = N_avg.*1e6.*18.015./6.022e23"("Online"=w734, "Offline"=w733, "sigma_on_total"=w756, "sigma_off_total"=w757, "gate_size"=w715) -> ("N_avg"=w717:cdb[], "w"=w718:cdb[])  [unwired: 1 in, 1 out]
                n573 = local read "Number of Bins"() -> (w723:u32)
                n574 = local read "Altitude Array (km)"() -> (w702:dbl[])
                n575 = local read "Time Resolution Per Bin(ns)"() -> (w732:u32)
                n576 = local read "Number of Bins"() -> (w711:u32)
                n577 = Logarithm Base 10(1:w701) -> (0:w708:dbl[])
                n578 = Reshape Array(w718, 1, w723) -> (→"Absolute Humdity":cdb[][])
                n579 = Build Array(w703, w701) -> (w705:dbl[][])
                n580 = Reshape Array(w708, 1, w711) -> (→"Backscatter coef":dbl[][])
                n581 = call "Convert to Dynamic Data9"("Array"=w717) -> ("Dynamic Data Type"=w721:dynamicdata)  [unwired: 3 in]
                n582 = To Double Precision Float(number=w732) -> (double precision float=w753:dbl)
                n583 = call "Convert to Dynamic Data6"("Array"=w718) -> ("Dynamic Data Type"=w719:dynamicdata)  [unwired: 3 in]
                n584 = Multiply(x=0.15, y=w753) -> (x*y=w751:dbl)
                n585 = call "Convert to Dynamic Data8"("Array"=w702) -> ("Dynamic Data Type"=w722:dynamicdata)  [unwired: 3 in]
                n586 = call "Convert to Dynamic Data5"("Array"=w702) -> ("Dynamic Data Type"=w720:dynamicdata)  [unwired: 3 in]
                n587 = call "Build XY Graph"("Y Input"=w722, "X Input"=w721) -> ("XY Graph"=→"Water Vapor Number Density":cluster{"Y":dbl[], "Y":dbl[]}[])  [unwired: 3 in, 6 out]
                n588 = call "Build XY Graph3"("Y Input"=w720, "X Input"=w719) -> ("XY Graph"=→"Absolute Humidity":cluster{"Y":dbl[], "Y":dbl[]}[])  [unwired: 3 in, 6 out]
                n589 = Divide(x=300.0, y=w751) -> (x/y=w748:dbl)
                n590 = Divide(x=450.0, y=w751) -> (x/y=w747:dbl)
                n591 = call "Convert to Dynamic Data11"("2D Array"=w705) -> ("Dynamic Data Type"=w704:dynamicdata)  [unwired: 3 in]
                n592 = call "Convert to Dynamic Data10"("Array"=w702) -> ("Dynamic Data Type"=w706:dynamicdata)  [unwired: 3 in]
                n593 = To Long Integer(number=w748) -> (32bit integer=w746:i32)
                n594 = To Long Integer(number=w747) -> (32bit integer=w745:i32)
                n595 = Decrement(x=w746) -> (x-1=w743:i32)
                n596 = Decrement(x=w745) -> (x-1=w744:i32)
                n597 = call "Build XY Graph5"("Y Input"=w706, "X Input"=w704) -> ("XY Graph"=→"aerosol profile":cluster{"Y":dbl[], "Y":dbl[]}[])  [unwired: 3 in, 6 out]
                n598 = Array Subset(array=w734, index=w743, length=w744) -> (w742:dbl[])
                n599 = Array Subset(array=w733, index=w743, length=w744) -> (w741:dbl[])
                n600 = call-poly <vilib>:"Mean.vi"("X"=w742) -> ("mean"=w740:dbl)  [unwired: 1 out]
                n601 = call-poly <vilib>:"Mean.vi"("X"=w741) -> ("mean"=w739:dbl)  [unwired: 1 out]
                n602 = Divide(x=w740, y=w739) -> (x/y=w738:dbl)
                n603 = Multiply(x=w733, y=w738) -> (x*y=w737:dbl[])
                n604 = Divide(x=w734, y=w737) -> (x/y=w736:dbl[])
                n605 = Natural Logarithm(1:w736) -> (0:w735:dbl[])
                n606 = Multiply(x=-1.0, y=w735) -> (x*y=w729:dbl[])
                n607 = call "Convert to Dynamic Data"("Array"=w729) -> ("Dynamic Data Type"=w731:dynamicdata)  [unwired: 3 in]
                n608 = call "Convert to Dynamic Data2"("Array"=w702) -> ("Dynamic Data Type"=w728:dynamicdata)  [unwired: 3 in]
                n609 = call "Build OD Plot"("Y Input"=w728, "X Input"=w731) -> ("XY Graph"=→"Optical Depth":cluster{"Y":dbl[], "Y":dbl[]}[])  [unwired: 3 in, 6 out]
              }
            }
          }
        }
        "L_Count" <- w129
      }
    }
  }
  n610 = case shown="True" w3 {
    frame False {
    }
    frame True {
      # "close data files"
      n611 = local read "NF_Off_Ref"() -> (w759:refnum<file>)
      n612 = local read "NF_On_Ref"() -> (w760:refnum<file>)
      n613 = local read "FF_Off_Ref"() -> (w761:refnum<file>)
      n614 = local read "FF_On_Ref"() -> (w762:refnum<file>)
      n615 = local read "WS_On/Off"() -> (w758:bool)
      n616 = case shown="True" w758 {
        frame False {
        }
        frame True {
          n617 = local read "WS visa"() -> (w763:refnum<visa-resource-name>)
          n618 = call "T_RH_P.vi"("VISA in"=w763, "WS_Commands"=enum16{"OpenWS", "ReadTRHP", "CloseWS"}."CloseWS") -> ()  [unwired: 11 in, 3 out]
        }
      }
      n619 = Close File(refnum=w762) -> ()  [unwired: 1 in, 2 out]
      n620 = Close File(refnum=w761) -> ()  [unwired: 1 in, 2 out]
      n621 = Close File(refnum=w760) -> ()  [unwired: 1 in, 2 out]
      n622 = Close File(refnum=w759) -> ()  [unwired: 1 in, 2 out]
    }
  }
  "FileHour" <- -1 ("FileHour")
  "DataOpen" <- FALSE
